vi "Gel Tugging Force Mode_Controller v15.20.vi"() -> ()   [LabVIEW 2015]
doc: "This example demonstrates how to continuously acquire voltage measurements from a DAQmx device using hardware timed, single point reads using a timed loop structure. The timed loop is controlled by the sample clock of the DAQ device. The device will read data on each tick of the sample clock. If an additional sample clock tick occurs before the current data point is read from the device or if the timed loop does not receive any sample clock ticks, a dialog will indicate that this has happened. \n\nHardware Timed Single Point acquisition works best when using a deterministic operating system (such as LabVIEW Real-Time). Because of the less deterministic nature of general purpose operating systems (such as Microsoft Windows), the software loop will not always take the exact same amount of time to execute, and this may lead to the occasional missed sample clock. \n\nFor instructions on how to connect your signals to the DAQ device, refer to your device documentation."
uses:
  <vilib>/Platform/TimedLoop/XDataNode/timing_clust.ctl
  <vilib>/Platform/TimedLoop/XDataNode/nitl_modes.ctl
  <vilib>/Platform/TimedLoop/XDataNode/wakeup.ctl
  <vilib>/dex/Flush And Wait Empty Condition.ctl
  <vilib>/DAQmx/read.llb/DAQmx Read (Analog 1D DBL NChan 1Samp).vi
  <vilib>/DAQmx/write.llb/DAQmx Write (Analog DBL 1Chan 1Samp).vi
  <vilib>/DAQmx/read.llb/DAQmx Read (Analog 2D DBL NChan NSamp).vi
  <vilib>/Analysis/baseanly.llb/Mean (DBL).vi
  <vilib>/DAQmx/create/channels.llb/DAQmx Create Channel (AI-Voltage-Basic).vi
  <vilib>/DAQmx/create/channels.llb/DAQmx Create Channel (AO-Voltage-Basic).vi
  <vilib>/DAQmx/configure/timing.llb/DAQmx Timing (Sample Clock).vi
  <vilib>/DAQmx/create/timing.llb/DAQmx Create Timing Source (Control Loop From Task).vi
  <vilib>/DAQmx/miscellaneous.llb/DAQmx Fill In Error Info.vi
  <vilib>/addons/control/pid/pid.llb/PID (DBL).vi
  <vilib>/addons/control/pid/pid.llb/PID Gain Schedule (DBL).vi
  <vilib>/platform/TimedLoop/XDataNode/XDataNode.xnode
  <vilib>/Analysis/NI_AALBase.lvlib
  <vilib>/addons/control/pid/NI_PID_pid.lvlib
  <vilib>/Platform/TimedLoop/XDataNode/XDNodeRunTimeDep.lvlib
  <vilib>/ptbypt/NI_PtbyPt.lvlib
panel:
  in  "1st OFF Length (s)":dbl=2.0
  out "Calibrating Sensor":bool
  out "Waveform Graph 2":dbl[](graph)
  in  "Ramp Total Interval (ms)":u32=490
  in  "# Ramp Steps":u32=7
  in  "9.            Step(s) Force Ramp in              (ms)?":bool=TRUE
  in  "ON":dbl=3.0
  out "DigitalTrigger":bool
  out "Corrective \nNull Flux (Gs)":dbl
  in  "7. Correct Null Flux after Cycle #1?":bool=TRUE
  out "# of Data Points":i64
  out "Loop Index":i32
  in  "6. Mini DeGauss cycles in OFF segments?":bool
  in  "Measure Flux Sensor Zero?":bool=TRUE
  out "PID gains ON Chosen":T1
  in  "Keep Null Flux Running \n       Until Next Step? 2":bool
  in  "Start Null Flux Adjustment 2":bool
  out "PID gains OFF Chosen":T1
  in  "Tweaked PID gains ON":T1={"proportional gain (Kc)"=0.7, "integral time (Ti, min)"=3.5e-06, "derivative time (Td, min)"=0.0}
  in  "Tweaked PID gains OFF":T1={"proportional gain (Kc)"=0.078, "integral time (Ti, min)"=3.5e-06, "derivative time (Td, min)"=0.0}
  out "Ready?":bool
  in  "4. Aggressiveness:":i32(listbox)
  out "of":i32
  in  "3. PID Parameters:":i32(listbox)
  out "ON Absolute\nFlux Setpoint (Gs)":dbl
  out "Suggested PID gains OFF":T1
  out "Suggested PID gains ON":T1
  out "Measured Magnetic Sensor 1 Zero, Mean (V)":dbl format="%_7g"
  in  "OFF (s)":dbl=4.0
  out "Round:":i32
  out "Ready?":bool
  out "Ready?":bool
  in  "Proceed with Parameters":bool
  out "Final Flux Running at End?":bool
  out "Sensor Sensitivity \n(V/Gs)":dbl
  in  "1. Sensor:":i32(listbox)
  out "Ready?":bool
  in  "2. Needle:":i32(listbox)
  in  "Proceed with Selection":bool
  in  "Ready?&\nData Logger Running":bool
  out "Null Flux \nCurrently\nRunning?":bool
  out "Real-Time Flux Control Currently Running?":bool
  out "Ready?":bool
  out "DeGaussing?":bool
  in  "Start DeGaussing":bool
  in  "Start Null Flux Adjustment":bool
  in  "1. Number of rounds":i32=3
  in  "Post-Wave Null Flux Interval (s)":dbl=4.0 format="%#_13g"
  in  "Pre-Wave Null Flux Interval (s)":dbl format="%#_13g"
  in  "8. Keep Final Flux Running at End?":bool=TRUE
  out "Flux Control Sequence Running & Uploading Data?":bool
  in  "3. Keep Null Flux Running \n       Until Next Step?":bool=TRUE
  in  "2. Adjust Magnetic Flux (GS):":dbl=3.5 min=-350.0 max=350.0 step=0.02 format="%#_13g"
  in  "4. Click Rocker to finish Null Flux Adjustment":bool
  in  "Number of Cycles":i32=3
  in  "Flux ON relative setpoint (Gs)":dbl=-175.0 format="%#_13g"
  # "For Gel Tugging Experiments v15.20 (Controlled-Flux or Force Mode)"
  # "WARNING: This program crashes the first 2 or 3 times it runs after the target has been shut down. \nWARNING: Do NOT run the power supply unattended with the needle attached. Always look at the amount of current periodically."
  # "Step 0-1: Place the needle at Z ~ 7000 micron in the field of view. Inclincation Angle= 25º for HyMu80#1 Needle"
  # "(Hit \"Enter\" \nor Toggle)"
  # "Step 0-2: DeGauss Needle:"
  # "Step 0-3: Measure the Value of Flux Sensor \"Zero\"?"
  # "Yes"
  # "No"
  # "(Note: Check if it is around 2.47±0.02 (V)):"
  # "Step 1: Choose Sensor & \nNeedle/PID Parameters\nfor This Experiment:"
  # "Step 2: Adjust Flux: \n(in Real-Time)"
  # "(Hit \"Enter\" \nor Toggle)"
  # "Yes"
  # "No"
  # "Make sure upper side of Rocker\n is pressed down before Program Starts"
  # "Step 3: Specify Control \n     Sequence Parameters:"
  # "1. Pre-Wave Null Flux Interval (s) (choose 0 if none desired):"
  # "2. Length of 2nd to end OFF"
  # "& ON"
  # "segments (s)."
  # "Length of 1st OFF"
  # "3. Number of OFF & ON Square-Wave Cycles:"
  # "Note 1: Use Negative Flux for waves in opposite direction\nNote 2: Linear Range is (±0-175 Gs) for Null Flux + Flux ON Setpoint\nNote 3: Check ON Absolute Flux Setpoint & PID Gains on first run.\nSometimes they can be glitchy. Abort & Re-run"
  # "4. Flux ON relative setpoint (Gs):"
  # "5. Post-Wave Null Flux Inteval (s) (choose 0 if none desired):"
  # "No"
  # "Yes"
  # "No"
  # "Yes"
  # "No"
  # "Yes"
  # "No"
  # "Yes"
  # "Step 4: Do you want to tweak these PID parameters?"
  # "Yes"
  # "No"
  # "vs."
  # "Step 5: Run Data Logger: Gel Tugging Force Mode_Data Logger_Auto-Manual Triggers v15.20.vi\n            Needs to be running to start the control sequence"
  # "Step 6-1: Lower the needle to the desired level for the experiment. Z ~ 3400 microns with TI-SH-U stage.\nStep 6-2: Click TRGR or Run Macro in Nikon Elements"
  # "datapoints uploaded"
  # "out of"
  # "Close the VI and start over. The VI sometimes freezes upon subsequent runs"
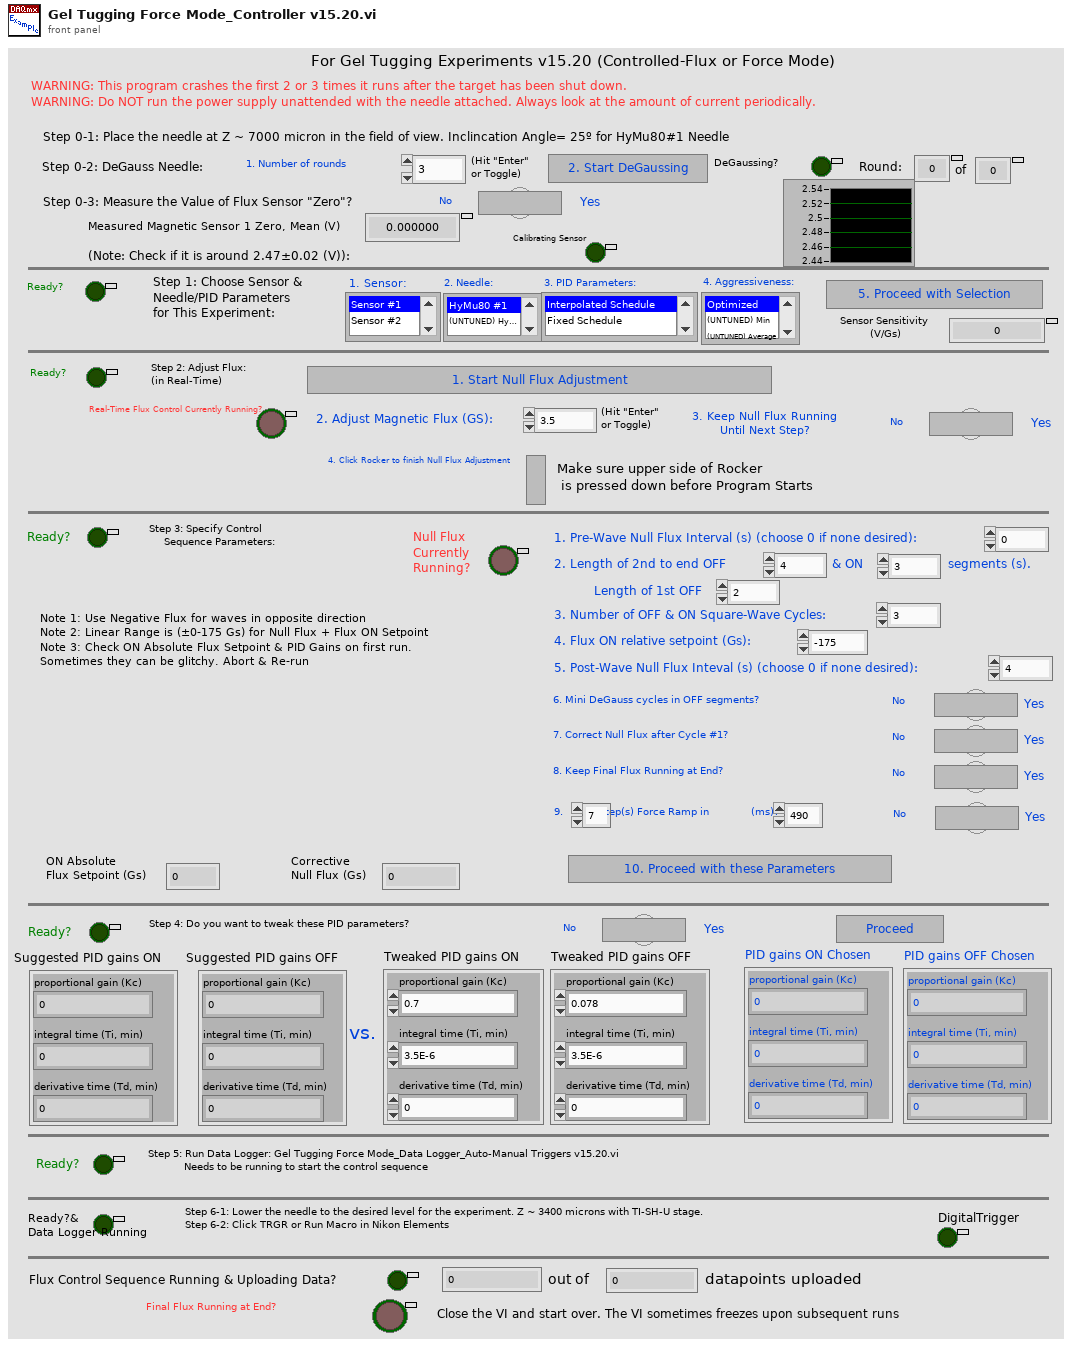
[diagram p1: front panel]
types:
  T1 = cluster{"proportional gain (Kc)":dbl, "integral time (Ti, min)":dbl, "derivative time (Td, min)":dbl}
  T2 = cluster{"PID gains":cluster{"proportional gain (Kc)":dbl, "integral time (Ti, min)":dbl, "derivative time (Td, min)":dbl}, "max value":dbl}[]
  T3 = typedef "XDNodeRunTimeDep.lvlib/timing_clust.ctl" = cluster{"Expected End [f-1]":u64, "Actual End [f-1]":u64, "Finished Late? [f-1]":bool, "Expected End [i-1]":u64, "Actual End [i-1]":u64, "Finished Late? [i-1]":bool, "Expected Start [i]":u64, "Actual Start [i]":u64, "Expected Start [f]":u64, "Actual Start [f]":u64, "Source Name":string, "Structure Name":string, "Period":i64, "Deadline":i64, "Offset":i64, "Start":i64, "Priority":i32, "Timeout":i32, "Mode":T4, "Wakeup Reason":T5, "Error":errorcluster, "Source Type":string, "Secondary Source Type":string, "Global End Time":u64, "Global Start Time":u64, "Frame Duration":u64, "Iteration Duration":u64, "Assigned CPU":i32, "I/O Scan Engine Mode":u32}
  T4 = typedef "XDNodeRunTimeDep.lvlib/nitl_modes.ctl" = enum32{"No Change", "Process missed periods, maintain original phase", "Discard missed periods, maintain original phase", "Process missed periods, ignore original phase", "Discard missed periods, ignore original phase"}
  T5 = typedef "XDNodeRunTimeDep.lvlib/wakeup.ctl" = enum32{"Normal", "Aborted", "Asynchronous wakeup", "Timing source error", "Timed loop error", "Timeout"}
  T6 = cluster{"Max/Min \ncontroller outputs":dbl, "output low":dbl}
  T7 = cluster{"PID gains":cluster{"proportional gain (Kc)":dbl, "integral time (Ti, min)":dbl, "derivative time (Td, min)":dbl}, "max value":dbl}
  T8 = typedef "Flush And Wait Empty Condition.ctl" = u8
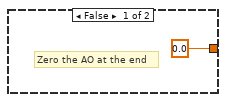
[diagram p2: hidden frame]
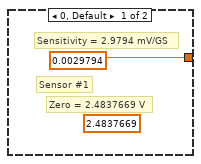
[diagram p4: hidden frame]
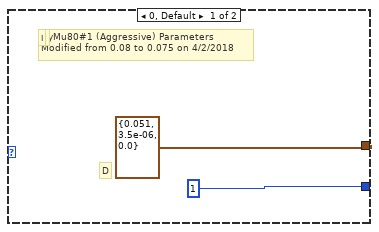
[diagram p5: hidden frame]
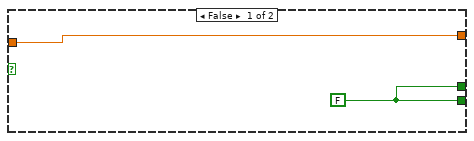
[diagram p6: hidden frame]
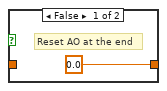
[diagram p7: hidden frame]
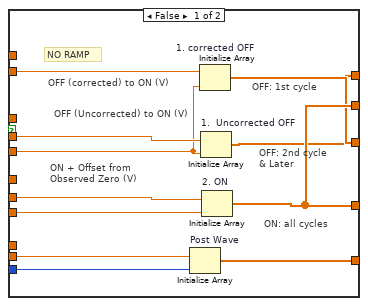
[diagram p9: hidden frame]
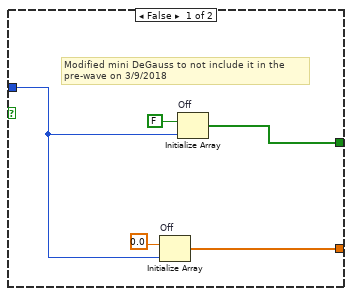
[diagram p11: hidden frame]
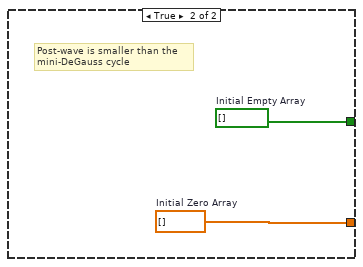
[diagram p12: hidden frame]
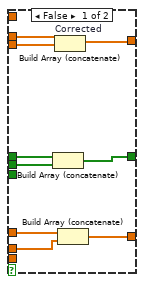
[diagram p14: hidden frame]
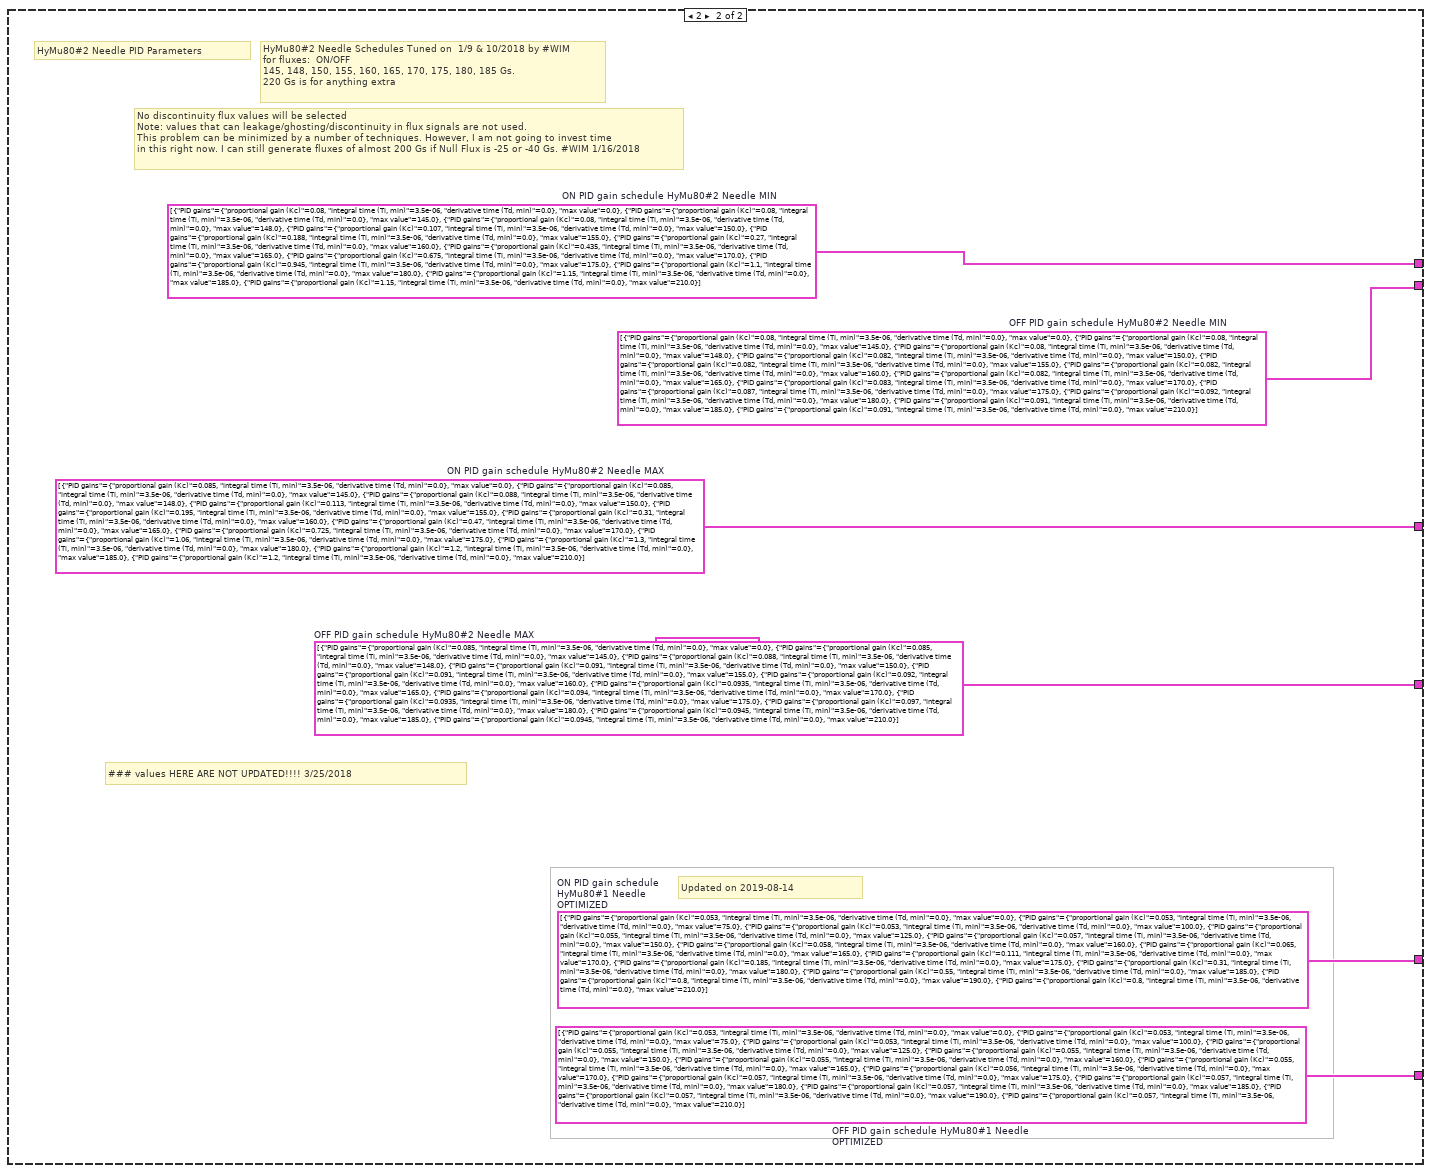
[diagram p18: hidden frame]
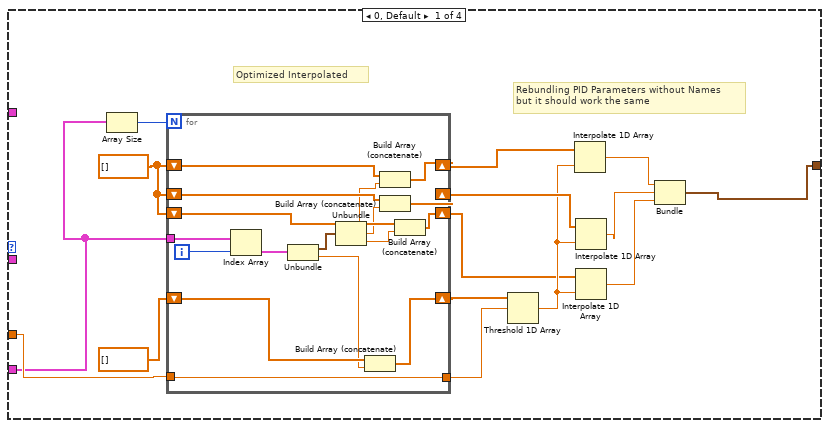
[diagram p19: hidden frame]
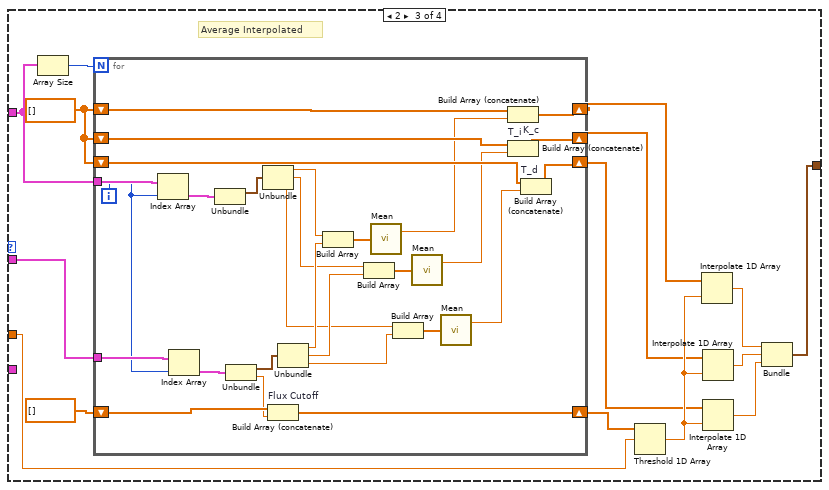
[diagram p20: hidden frame]
diagram:
  (unwired) T2 [{"PID gains"={"proportional gain (Kc)"=0.07, "integral time (Ti, min)"=3.5e-06, "derivative time (Td, min)"=0.0}, "max value"=0.0}, {"PID gains"={"proportional gain (Kc)"=0.07, "integral time (Ti, min)"=3.5e-06, "derivative time (Td, min)"=0.0}, "max value"=143.0}, {"PID gains"={"proportional gain (Kc)"=0.078, "integral time (Ti, min)"=3.5e-06, "derivative time (Td, min)"=0.0}, "max value"=148.0}, {"PID gains"={"proportional gain (Kc)"=0.078, "integral time (Ti, min)"=3.5e-06, "derivative time (Td, min)"=0.0}, "max value"=150.0}, {"PID gains"={"proportional gain (Kc)"=0.078, "integral time (Ti, min)"=3.5e-06, "derivative time (Td, min)"=0.0}, "max value"=155.0}, {"PID gains"={"proportional gain (Kc)"=0.078, "integral time (Ti, min)"=3.5e-06, "derivative time (Td, min)"=0.0}, "max value"=160.0}, {"PID gains"={"proportional gain (Kc)"=0.078, "integral time (Ti, min)"=3.5e-06, "derivative time (Td, min)"=0.0}, "max value"=165.0}, {"PID gains"={"proportional gain (Kc)"=0.078, "integral time (Ti, min)"=3.5e-06, "derivative time (Td, min)"=0.0}, "max value"=170.0}, {"PID gains"={"proportional gain (Kc)"=0.081, "integral time (Ti, min)"=3.5e-06, "derivative time (Td, min)"=0.0}, "max value"=175.0}, {"PID gains"={"proportional gain (Kc)"=0.081, "integral time (Ti, min)"=3.5e-06, "derivative time (Td, min)"=0.0}, "max value"=180.0}, {"PID gains"={"proportional gain (Kc)"=0.085, "integral time (Ti, min)"=3.5e-06, "derivative time (Td, min)"=0.0}, "max value"=185.0}, {"PID gains"={"proportional gain (Kc)"=0.086, "integral time (Ti, min)"=3.5e-06, "derivative time (Td, min)"=0.0}, "max value"=190.0}, {"PID gains"={"proportional gain (Kc)"=0.086, "integral time (Ti, min)"=0.01, "derivative time (Td, min)"=0.0}, "max value"=195.0}, {"PID gains"={"proportional gain (Kc)"=0.086, "integral time (Ti, min)"=0.01, "derivative time (Td, min)"=0.0}, "max value"=220.0}]  # OFF PID gain schedule HyMu80#1 Needle OPTIMIZED
  (unwired) T2 [{"PID gains"={"proportional gain (Kc)"=0.065, "integral time (Ti, min)"=3.5e-06, "derivative time (Td, min)"=0.0}, "max value"=0.0}, {"PID gains"={"proportional gain (Kc)"=0.065, "integral time (Ti, min)"=3.5e-06, "derivative time (Td, min)"=0.0}, "max value"=143.0}, {"PID gains"={"proportional gain (Kc)"=0.083, "integral time (Ti, min)"=3.5e-06, "derivative time (Td, min)"=0.0}, "max value"=148.0}, {"PID gains"={"proportional gain (Kc)"=0.084, "integral time (Ti, min)"=3.5e-06, "derivative time (Td, min)"=0.0}, "max value"=150.0}, {"PID gains"={"proportional gain (Kc)"=0.0875, "integral time (Ti, min)"=3.5e-06, "derivative time (Td, min)"=0.0}, "max value"=155.0}, {"PID gains"={"proportional gain (Kc)"=0.123, "integral time (Ti, min)"=3.5e-06, "derivative time (Td, min)"=0.0}, "max value"=160.0}, {"PID gains"={"proportional gain (Kc)"=0.187, "integral time (Ti, min)"=3.5e-06, "derivative time (Td, min)"=0.0}, "max value"=165.0}, {"PID gains"={"proportional gain (Kc)"=0.315, "integral time (Ti, min)"=3.5e-06, "derivative time (Td, min)"=0.0}, "max value"=170.0}, {"PID gains"={"proportional gain (Kc)"=0.46, "integral time (Ti, min)"=3.5e-06, "derivative time (Td, min)"=0.0}, "max value"=175.0}, {"PID gains"={"proportional gain (Kc)"=0.59, "integral time (Ti, min)"=3.5e-06, "derivative time (Td, min)"=0.0}, "max value"=180.0}, {"PID gains"={"proportional gain (Kc)"=0.8875, "integral time (Ti, min)"=3.5e-06, "derivative time (Td, min)"=0.0}, "max value"=185.0}, {"PID gains"={"proportional gain (Kc)"=1.04, "integral time (Ti, min)"=3.5e-06, "derivative time (Td, min)"=0.0}, "max value"=190.0}, {"PID gains"={"proportional gain (Kc)"=1.04, "integral time (Ti, min)"=0.01, "derivative time (Td, min)"=0.0}, "max value"=195.0}, {"PID gains"={"proportional gain (Kc)"=1.04, "integral time (Ti, min)"=0.01, "derivative time (Td, min)"=0.0}, "max value"=220.0}]  # ON PID gain schedule HyMu80#1 Needle OPTIMIZED
  (unwired) T2 [{"PID gains"={"proportional gain (Kc)"=0.07, "integral time (Ti, min)"=3.5e-06, "derivative time (Td, min)"=0.0}, "max value"=0.0}, {"PID gains"={"proportional gain (Kc)"=0.07, "integral time (Ti, min)"=3.5e-06, "derivative time (Td, min)"=0.0}, "max value"=116.0}, {"PID gains"={"proportional gain (Kc)"=0.078, "integral time (Ti, min)"=3.5e-06, "derivative time (Td, min)"=0.0}, "max value"=117.0}, {"PID gains"={"proportional gain (Kc)"=0.08, "integral time (Ti, min)"=3.5e-06, "derivative time (Td, min)"=0.0}, "max value"=120.0}, {"PID gains"={"proportional gain (Kc)"=0.08, "integral time (Ti, min)"=3.5e-06, "derivative time (Td, min)"=0.0}, "max value"=122.0}, {"PID gains"={"proportional gain (Kc)"=0.08, "integral time (Ti, min)"=3.5e-06, "derivative time (Td, min)"=0.0}, "max value"=125.0}, {"PID gains"={"proportional gain (Kc)"=0.08, "integral time (Ti, min)"=3.5e-06, "derivative time (Td, min)"=0.0}, "max value"=130.0}, {"PID gains"={"proportional gain (Kc)"=0.08, "integral time (Ti, min)"=3.5e-06, "derivative time (Td, min)"=0.0}, "max value"=135.0}, {"PID gains"={"proportional gain (Kc)"=0.08, "integral time (Ti, min)"=3.5e-06, "derivative time (Td, min)"=0.0}, "max value"=140.0}, {"PID gains"={"proportional gain (Kc)"=0.086, "integral time (Ti, min)"=3.5e-06, "derivative time (Td, min)"=0.0}, "max value"=145.0}, {"PID gains"={"proportional gain (Kc)"=0.096, "integral time (Ti, min)"=3.5e-06, "derivative time (Td, min)"=0.0}, "max value"=150.0}, {"PID gains"={"proportional gain (Kc)"=0.096, "integral time (Ti, min)"=3.5e-06, "derivative time (Td, min)"=0.0}, "max value"=200.0}]  # OFF PID gain schedule HyMu80#1 Needle OPTIMIZED
  (unwired) T2 [{"PID gains"={"proportional gain (Kc)"=0.07, "integral time (Ti, min)"=3.5e-06, "derivative time (Td, min)"=0.0}, "max value"=0.0}, {"PID gains"={"proportional gain (Kc)"=0.07, "integral time (Ti, min)"=3.5e-06, "derivative time (Td, min)"=0.0}, "max value"=116.0}, {"PID gains"={"proportional gain (Kc)"=0.08, "integral time (Ti, min)"=3.5e-06, "derivative time (Td, min)"=0.0}, "max value"=117.0}, {"PID gains"={"proportional gain (Kc)"=0.085, "integral time (Ti, min)"=3.5e-06, "derivative time (Td, min)"=0.0}, "max value"=120.0}, {"PID gains"={"proportional gain (Kc)"=0.115, "integral time (Ti, min)"=3.5e-06, "derivative time (Td, min)"=0.0}, "max value"=122.0}, {"PID gains"={"proportional gain (Kc)"=0.18, "integral time (Ti, min)"=3.5e-06, "derivative time (Td, min)"=0.0}, "max value"=125.0}, {"PID gains"={"proportional gain (Kc)"=0.31, "integral time (Ti, min)"=3.5e-06, "derivative time (Td, min)"=0.0}, "max value"=130.0}, {"PID gains"={"proportional gain (Kc)"=0.55, "integral time (Ti, min)"=3.5e-06, "derivative time (Td, min)"=0.0}, "max value"=135.0}, {"PID gains"={"proportional gain (Kc)"=0.95, "integral time (Ti, min)"=3.5e-06, "derivative time (Td, min)"=0.0}, "max value"=140.0}, {"PID gains"={"proportional gain (Kc)"=1.2, "integral time (Ti, min)"=3.5e-06, "derivative time (Td, min)"=0.0}, "max value"=145.0}, {"PID gains"={"proportional gain (Kc)"=1.3, "integral time (Ti, min)"=3.5e-06, "derivative time (Td, min)"=0.0}, "max value"=150.0}, {"PID gains"={"proportional gain (Kc)"=1.3, "integral time (Ti, min)"=3.5e-06, "derivative time (Td, min)"=0.0}, "max value"=200.0}]  # ON PID gain schedule HyMu80#1 Needle OPTIMIZED
  # "Note: Some quirks when running the program are: (as of 2/7/2018):\n1. First time you run it for the day, it will ask if you want to use the newer version instead of the old one already on the Remote Desktop computer\n2. Also, at the end of the first run, it will not stop. You will have to abort it. Some of the data points will be lost near the end. You might have to repeat that run.\n3. Do run the Data Reduction file or any other VIs in the DeGaussing stage. Otherwise, the program will crash."
  # "v15.20 Modified from v15.10 by Waddah Moghram on 2019-08-16 and thereafter:\n*Update based on Calibration_Core Flux Controller v11.00.vi\n\nv15.10 modified from v15.00 by  #Waddah #Moghram on 11/5/2018 and thereafter:\nTo be used with Data Logger v15.00 & Reduction v15.00: \n1. Modified it so that it can select PID gains from inside the loop\n2. Modified some PID gains at 170 Gs and higher.\n3.  Fixed the problem with the Post-wave zero Ramp 11/28/2019. WIM\n\nv 15.00 Modified from v12.00 by #Waddah #Moghram on 10/10/2018 and thereafter. To be used with Data Logger v1500 & Reduction v15.00: \n1. Replaced the Mini-DeGauss Routine with a Force Ramp (Linear vs. Steps?) since a step force function will be difficult to image-track. \n((Please refer to Linear and Step Ramps v1.00.vi for both linear and step ramps).\n*** Amount of step jump is assumed to be from ON-to-OFF and OFF-to-ON. That information is known\n2. Some of the parameters that will be used for the force ramp:\n*** Time interval: Assume that ON-to-OFF and OFF-to-ON ramps will have the same time frames.\n*** If discrete step are chosen. Choose the number of steps that it will take.\n\nv 11.00 Modified from v10.00 by #Waddah #Moghram on 4/26/2018 and thereafter. To be used with Data Logger v11.00 & Reduction v11.00: \n1. Resolve the issue of Digital Trigger automatically being released due to ground loop. Most likely due to construction that is happening around.\n* The Network digital trigger is released from the Master DAQ in the Data Logger, where it will be passed into here as a real-time global variable.\n2. For some reason, the first two runs usually crash, and the program still crashes a lot. I need to find a work around this one. \n\nv 10.00 Modified from v9.60 and v9.40 by #Waddah #Moghram on 4/4/2018 and thereafter: To be used with Data Logger v10.00 & Reduction v10.00\n1. Increased DeGauss Cycle to 2,000 milliseconds from 500 ms.\n2. Corrected the Dialog Boxes\n3. Added a switch for the Corrective Null Flux on the front panel, display it and send it to the Data Logger\n4. Corrected Mini-DeGauss Sampling Glitch where it was wired to the sampling rate directly instead of the one adjusted by the period 4/4/2018\n5. Based on a sigmoidal curve fit 4/18/2018.\nThe Equation is Y = Vmax * X^h /(K_prime + X^h), where Vmax = 10.7369, h = 1.91107, and Kprime = 3499.9. (and K_half = 71.5294))\n\n\nv 9.60 Modified from v9.50 by #Waddah #Moghram on 4/1/2018: \n1. It will correct for the Null Flux shift based on the Sigmoidal Fit that was collected from bead in front of the needle data,\nbased on a sigmoidal curve fit 4/2/2018. Experiments conducted 3/29/2018-4/2/2018. \nThe Equation is Y = Vmax * X^h /(K_prime + X^h), where Vmax = 11.4533, h = 1.69622, and Kprime = 1256.11)\n2. New Global Variable \"FluxObservedZeroGsCorrected\" to be inserted into the Data Logger v9.60\n\nv 9.50 Modified from v9.40 by #Waddah #Moghram on 3/29/2018:\n1. Used AI7 to hook up the 2nd Magnetic Sensor that will be placed in front of the sensor.\n2. Zero of 2nd Sensor is measured in the first step as well. The sensitivity is embedded in the data logger as well. \n3. Accompanies by v9.50 Data Logger.\n4. (GO BACK TO OLDER VERSION and add more details about modifications)\nFixed datapoints lost in the end due to the determinstic loop ending before the other loop. \n\nv 9.40 Modified from v9.20 by #Waddah #Moghram on 3/19/2018\n1. Removed Offset and kept amplitude +/- 10V for MiniDeGauss waveforms from inside the deterrministic loop.\n2. Shuffled the Suggested PID Loop parameters until before the \"Proceed button to allow the user to take a look at them. \n3. 3/22/2018. Reverted back to unshielded magnetic sensor, but with wire propped away from sensor.\nAlso, TI-SH-U is used and the needle is placed at Z~4600 microns for PID tuning with an inclination angle of 20 degrees\n(#OLD: 3. Re-optimized on 3/20/2018 for HyMu80#1 after shielding the sensor. The values were shifted down by 23 Gs   3/20/2018 )\n(#OLD: 4. Relocated PID Gains Selected on the front panel for more clarity 3/21/2018.)\n\nv 9.20 Modified from v9.05 and v9.10 by #Waddah #Moghram on 3/12/2018 and thereafter:\n1. It is back to OFF/ON Sequences, except first OFF segment and pre-waves have no DeGauss. It turns out to be an easy fix. \n2. Modified mini-DeGauss time \n3. Tied variables to make the wave sample properly. See notes for calculations.\n4. Turn OFF \"Null Flux Running Middle\" when control sequence starts. 3/17/2018 WIM \n5. Modified PID Parameters for #Interpolated #Optimized #HyMu80#1. Other parameters will need to be modified later on. \n6. Updated front panel to indicate inclination Angle, and Z-level for both Sensor Zero Measurement and Control Sequence.   3/18/2018\n****It turns out the PID parameters are sensitive to both z-level and inclination angle (which affect the Sensor Zero Measurement).*****\n***NOTE: First run usually does not end by itself. You will have to abort it. It will result in the loss of the last few hundred data points, but that is not too critical. Otherwise, run once, then run again. It should run smoothly every time afterwards. This is one of the quirks of working with LabVIEW. 3/18/2018\n\nv 9.05 Modified from v9.00 by #Waddah #Moghram on 3/12/2018:\n1. Modified Magnitude of Mini-DeGauss cycle from ** Maximum of (AO of Null Flux (AO_nf) or AO of ON (AO_on)) ** to **AO_nf + AO_on**\n2. The mini DeGauss oscillates about AO_nf instead of 0\n\nv 9.00 Modified from v8.40 by #Waddah #Moghram on 3/7/2018 and thereafter:\n1. It will include mini-DeGauss Cycles in the beginning of the OFF segments before PID control kicks back in. This is in an effort to minimize Magnetic Sensor hysteresis at Null Flux Observed\n(Sinusoidally Decaying Waveform Embedded in Control Sequence v1.0.vi is used for initially testing of mini-DeGauss waveforms).\n** So far, the selected waveform is about ~ 15 cycles that exponentially decay under 30 milliseconds. Used a Cosine waveform instead of sine (Sin with 90 degree phase shift).\n** Middle point is AO = 0, Magnitude between max and middle point is AO_last**    (3/12/2018)\n2. Sequence is created externally to minimize Loop calculation time. The AO Mini-DeGauss will only to be multiplied by the amplitude of the last AO out. \n3. Switched #AI6 to #AI3. Some errors with AI6 signal on the DAQ on 3/8/2018\n4. Fixed the glitch where the PID loop overreacted when the PID starts again and the Setpoint point is close to the Process variable. (Kudos to #Dr. #Selby for catching it!). on 3/8/2018\n5. Replaced \"Zero Flux\" with \"Null Flux\" for labels to avoid confusion since it is not really zero\n\nv 8.40 Modified from v8.30 by #Waddah #Moghram on 3/1/2018, and thereafter: \n1. Added a toggle to allow the re-calibration of magnetic sensor Zero or not\n2. Global Variables for DeGauss Cycles Total & Round\n3. Modified Tabbing order on 3/4/2018\n4. Fixed AO 0 initialized before PID loop to keep the value saved from \"keep Null Flux Running\" step on 3/5/2018. It was creating a blip in PID response. However, that does not seem to resolve the problem.\n\nv 8.30 Modified from v8.20 by #Waddah #Moghram on 2/22/2018:\n1. Using the measured magnetic sensor zero to create the control sequence after DeGaussing instead of the one recorded a while back inside a shielded data.\nThis is because it will change a lot over time with thermal drift and so forth. \n2. Reset the value of the sensor zero every time even no deGaussing was done.\n\nv 8.20 Modified from v8.10 by #Waddah #Moghram on 2/2/2018: \n1. This will allow the user to tweak the PID Parameters one more time before the actual experiment. This was found because it turns out that PID parameters can shift with time especially for values in the non-linear range.\n\nv. 8.10 Modified from v8.00 by #Waddah #Moghram on 1/10/2018 and thereafter:\n1. Scrapped fitted PID gains and used interpolated schedules in addition to schedules\n2. Updated PID Values for Gains and so forth.\n\nv 8.00 Modified from v7.40 by #Waddah #Moghram on 1/1/2018 and thereafter:\n1. Used the PID Gains from PID Tuning experiments \n2. Removed Normal vs. Aggressive and now will only use one set of parameters such that only one set of parameters are used\n3. Created a choice of Scheduled vs. Fitted Parameters. 1/8/2018.\n4. Fixed glitch that passed old values of waveform parameters to the global variable 1/8/2018. \n\nv 7.40 Modified from v 7.30 by #Waddah #Moghram on 12/22/2017 to including the following:\n1. Shifting the flux check and current reset only if DeGuassing Cycle required is not equal to zero. Otherwise, skip it, and keep the current running. I did this in case I need more than one run without removing the needle from the sample\n2. corrected total number of data points to allow for more than 2 seconds 1/4/2018 by #WIM\n\nv 7.30 Modified from v 7.20 by #Waddah #Moghram on 12/21/2017 to including the following:\n1. Removed Magnetic Flux Sensor Zero Calibration step, and embedded that value in the sensor section. The idea for doing that is that I want the flux values stated to be absolute. Thermal drift of sensor should not matter since PID should still work regardless of where the zero lies. Moreover, if I am accounting for the Null Flux observed, it should not matter what the absolute flux zero is.\n2. However, I kept the AO reset and used the AI2 to keep it running and also measured sensor values for 2 seconds to make sure that my values are controlled properly.\n3. Steps were re-numbered\n\nv 7.20 Modified from v7.10 by #Waddah #Moghram on 12/18/2017 to include the following:\n1. Custom-Length Waveforms. Data Reduction & Logger will be changed accordingly.\n2. Added Normal (~40 ms response time) vs. Aggressive (~22 ms response time) PID Parameters on 12/20/2017\n\nV 7.10 Modified from v7.00 by #Waddah #Moghram on 12/18/2017 to include the following:\n1. Switch order of DeGaussing & Calibrating Zero of Sensor. First Ensure that there is no residual magnetic. And secondly, reset AO just in case!\n\nv 7.00 Modified from v6.00 by #Waddah #Moghram on 12/18/2017 to include the following:\n1. Calibrated Null Flux at the beginning of the experiment without shielding to account for thermal drifts:\n*** Imported from \"01 Magnetic Sensor Zero Calibration v2.0 - Target.vi\"\n2. Included Second per Cycle\n3. Cleanup interface & Changed Step Numbers.\n\nv 6.00 Modified from v5.22 by #Waddah #Moghram on 12/5/2017 to include the following: \n1. Newer Magnetic Sensor Sensitivities: Sensor 1 is 2.9794 mV/GS and Sensor 2 is 3.0418 mV/GS\n2. Newer Magnetic Sensor Zeroes when unshielded: Sensor 1 is 2.4837669 V and Sensor 2 is 2.4928421 V\nThis program will also be used also to tune the PID in addition Magnetic Needle Choices\nOn 12/13/2017, I overhauled the interface to streamline the proceess and fixed a few glitches that allowed the program to \nchose parameters before clicking on the digital trigger\n\nv 5.22 Modified from v.5.20 by #Waddah #Moghram on 9/25/2017 to include the following:\n1. Remove prompt to calibrate the magnetic sensor and run Null Flux program\n2. Embedded the calibrated Null Flux value into the program, now that the sensor is fixed to the HyMu80 needle #1\n\n\nv5.00 modified from v.3.70 and v.4.10 by #Waddah #Moghram. It should integrate variables from both VIs.\nOther modification include:\n1. User-Defined Pre-experiment Null Flux Period\n2. User-Defined Post-experiment Null Flux Period\nModified on 8/14&15/2017 to streamline the VI even more. Ran into some Ground Loop Issues in the meantime. See Lab Notes for details.\n\nv4.10 Modified on 8/8/2017 to:\n* account for AI5 only for flux sensor values being fed to PID control.\nNotice the PID control scheme process variable is different in that it is not subtracted from the setpoint as in v.3.70 in the first PID Loop\n*modified PID parameters to the optimized ones found (subject to verification)."
  # "Re-optimized on 3/21/2018 for HyMu80#1 after shielding the sensor. The cutoff values were shifted down by ~23-27 Gs\nPreviously Optimized on 3/17/2018 for HyMu80#1 Optimized. The rest will need to be updated later\nAdded 139 Gs to keep fixed values in between 0 and 140 Gs.   Flux at 150 Gs has a response time of ~80 ms. \nAny higher PID gains will result in spike"
  # "Unshielded Previously"
  # "TOTALLY SHIELDED PARAMETERS"
  # "AI"
  # "AO"
  n1 = flat-sequence {
    tunnel: [w332] -> w96
    tunnel: [w331] -> w95
    tunnel: [w330] -> w88
    tunnel: [w329] -> w76
    tunnel: [w344] -> w104
    tunnel: w96 -> [w342]
    tunnel: w95 -> [w341]
    tunnel: w88 -> [w340]
    tunnel: [w340] -> w87
    tunnel: [w339] -> w77
    tunnel: w76 -> [w339]
    tunnel: [w354] -> w105
    tunnel: w104 -> [w354]
    tunnel: w87 -> [w353]
    tunnel: [w353] -> w86
    tunnel: [w352] -> w78
    tunnel: w77 -> [w352]
    tunnel: w105 -> [w360]
    tunnel: [w359] -> w102
    tunnel: [w358] -> w90
    tunnel: w86 -> [w358]
    tunnel: [w357] -> w79
    tunnel: w78 -> [w357]
    tunnel: [w371] -> w114
    tunnel: [w370] -> w113
    tunnel: [w369] -> w112
    tunnel: [w368] -> w103
    tunnel: w102 -> [w368]
    tunnel: w90 -> [w367]
    tunnel: [w367] -> w89
    tunnel: [w365] -> w85
    tunnel: w79 -> [w366]
    tunnel: [w366] -> w75
    tunnel: w114 -> [w413]
    tunnel: w113 -> [w412]
    tunnel: w112 -> [w411]
    tunnel: [w410] -> w108
    tunnel: [w409] -> w107
    tunnel: [w408] -> w106
    tunnel: w103 -> [w399]
    tunnel: [w397] -> w92
    tunnel: w89 -> [w397]
    tunnel: w85 -> [w396]
    tunnel: w75 -> [w395]
    tunnel: [w395] -> w73
    tunnel: [w394] -> w58
    tunnel: w108 -> [w488]
    tunnel: w107 -> [w487]
    tunnel: w106 -> [w486]
    tunnel: w92 -> [w485]
    tunnel: [w485] -> w91
    tunnel: [w484] -> w74
    tunnel: w73 -> [w484]
    tunnel: [w483] -> w59
    tunnel: w58 -> [w483]
    tunnel: [w496] -> w94
    tunnel: w91 -> [w496]
    tunnel: w74 -> [w495]
    tunnel: [w495] -> w71
    tunnel: w59 -> [w494]
    tunnel: [w494] -> w56
    tunnel: [w508] -> w101
    tunnel: [w507] -> w100
    tunnel: [w506] -> w99
    tunnel: [w505] -> w98
    tunnel: [w504] -> w97
    tunnel: w94 -> [w503]
    tunnel: [w503] -> w93
    tunnel: [w502] -> w72
    tunnel: w71 -> [w502]
    tunnel: [w501] -> w57
    tunnel: w56 -> [w501]
    tunnel: [w500] -> w11
    tunnel: [w499] -> w10
    tunnel: [w518] -> w83
    tunnel: [w535] -> w84
    tunnel: [w680] -> w82
    tunnel: [w672] -> w81
    tunnel: w101 -> [w601]
    tunnel: w100 -> [w671]
    tunnel: w99 -> [w670]
    tunnel: w98 -> [w669]
    tunnel: w97 -> [w668]
    tunnel: [w667] -> w80
    tunnel: w93 -> [w667]
    tunnel: w72 -> [w666]
    tunnel: [w666] -> w70
    tunnel: w57 -> [w665]
    tunnel: [w665] -> w55
    tunnel: [w651] -> w50
    tunnel: [w637] -> w49
    tunnel: [w616] -> w46
    tunnel: [w610] -> w43
    tunnel: w11 -> [w520]
    tunnel: w10 -> [w595]
    tunnel: [w520] -> w1
    tunnel: w84 -> [w814]
    tunnel: [w813] -> w69
    tunnel: w83 -> [_]
    tunnel: w82 -> [w810]
    tunnel: [w809] -> w67
    tunnel: [w827] -> w65
    tunnel: w81 -> [w818]
    tunnel: [w817] -> w63
    tunnel: [w826] -> w61
    tunnel: w80 -> [w832]
    tunnel: w70 -> [w831]
    tunnel: w55 -> [w811]
    tunnel: [w811] -> w53
    tunnel: [w819] -> w52
    tunnel: w50 -> [w820]
    tunnel: w49 -> [w816]
    tunnel: [w815] -> w48
    tunnel: w46 -> [w829]
    tunnel: [w829] -> w45
    tunnel: w43 -> [w828]
    tunnel: [w828] -> w42
    tunnel: [w825] -> w9
    tunnel: [w824] -> w8
    tunnel: w1 -> [w822]
    tunnel: w69 -> [w1250]
    tunnel: [w1250] -> w68
    tunnel: w67 -> [w1249]
    tunnel: [w1249] -> w66
    tunnel: w65 -> [w1247]
    tunnel: [w1243] -> w64
    tunnel: w63 -> [w1248]
    tunnel: [w1248] -> w62
    tunnel: w61 -> [w1246]
    tunnel: [w1242] -> w60
    tunnel: [w1241] -> w54
    tunnel: w53 -> [w1241]
    tunnel: w52 -> [w1240]
    tunnel: [w1240] -> w51
    tunnel: w48 -> [w1239]
    tunnel: [w1239] -> w47
    tunnel: w45 -> [w1238]
    tunnel: [w1238] -> w44
    tunnel: w42 -> [w1237]
    tunnel: [w1237] -> w41
    tunnel: w9 -> [w1234]
    tunnel: w8 -> [w1233]
    tunnel: [w1234] -> w7
    tunnel: [w1233] -> w6
    tunnel: w68 -> [w1288]
    tunnel: [w1290] -> w40
    tunnel: [w1291] -> w38
    tunnel: [w1283] -> w36
    tunnel: [w1288] -> w34
    tunnel: [w1272] -> w33
    tunnel: [w1287] -> w32
    tunnel: w66 -> [w1280]
    tunnel: [w1280] -> w30
    tunnel: [w1284] -> w28
    tunnel: w64 -> [w1284]
    tunnel: w62 -> [w1286]
    tunnel: [w1286] -> w26
    tunnel: w60 -> [w1285]
    tunnel: [w1285] -> w25
    tunnel: w54 -> [w1281]
    tunnel: [w1281] -> w24
    tunnel: w51 -> [w1279]
    tunnel: [w1279] -> w22
    tunnel: w47 -> [w1278]
    tunnel: [w1278] -> w20
    tunnel: [w1277] -> w18
    tunnel: w44 -> [w1277]
    tunnel: w41 -> [w1276]
    tunnel: [w1276] -> w17
    tunnel: w7 -> [w1274]
    tunnel: w6 -> [w1275]
    tunnel: [w1275] -> w5
    tunnel: [w1274] -> w4
    tunnel: w40 -> [w1316]
    tunnel: [w1315] -> w39
    tunnel: w38 -> [w1318]
    tunnel: [w1317] -> w37
    tunnel: w36 -> [w1320]
    tunnel: [w1319] -> w35
    tunnel: w34 -> [w1322]
    tunnel: w33 -> [w1324]
    tunnel: w32 -> [w1342]
    tunnel: [w1341] -> w31
    tunnel: w30 -> [w1328]
    tunnel: [w1327] -> w29
    tunnel: w28 -> [w1335]
    tunnel: [w1336] -> w27
    tunnel: w26 -> [w1334]
    tunnel: w25 -> [w1338]
    tunnel: w24 -> [w1340]
    tunnel: [w1339] -> w23
    tunnel: w22 -> [w1332]
    tunnel: [w1331] -> w21
    tunnel: w20 -> [w1330]
    tunnel: [w1329] -> w19
    tunnel: w18 -> [_]
    tunnel: w17 -> [w1326]
    tunnel: [w1325] -> w16
    tunnel: [w1337] -> w15
    tunnel: [w1333] -> w14
    tunnel: [w1323] -> w13
    tunnel: [w1321] -> w12
    tunnel: w5 -> [w1314]
    tunnel: w4 -> [w1313]
    tunnel: [w1312] -> w3
    tunnel: [w1311] -> w2
    tunnel: w39 -> [w1428]
    tunnel: w37 -> [w1429]
    tunnel: w35 -> [w1425]
    tunnel: w31 -> [w1391]
    tunnel: [w1411] -> w111
    tunnel: [w1394] -> w110
    tunnel: w29 -> [w1393]
    tunnel: [w1383] -> w109
    tunnel: w27 -> [w1382]
    tunnel: w23 -> [w1374]
    tunnel: w21 -> [w1381]
    tunnel: w19 -> [w1379]
    tunnel: w16 -> [w1371]
    tunnel: w15 -> [w1387]
    tunnel: w14 -> [w1389]
    tunnel: w13 -> [w1380]
    tunnel: w12 -> [w1421]
    tunnel: w3 -> [w1364]
    tunnel: w2 -> [w1362]
    tunnel: w111 -> [w1648]
    tunnel: w110 -> [w1647]
    tunnel: w109 -> [w1649]
    frame #0 {
      # "Removed the thermocouple  * AI2 is connected to Thermocouple cable."
      # "Switched Ai6 to AI3 on 3/8/2018 \nSome issues with AI6 on DEV2"
      # "1. SPECIFY the number of DeGaussing Cycle. CLICK \"Start DeGaussing.\"\n2. SPECIFY the Sensor & Needle in use for this experiment."
      n2 = One Button Dialog(message="BEFORE YOU START: \n* VERIFY these DAQ-2/Slave cables are connected as the following:\n   * AI5 is connected to Magnetic Flux \"Sensor Output - RAW\" on the Magnetic sensor box.   \n   * AI3 is connected to \"Current Sensor (1A/V)\" on the Load Box.\n   * AI7 is connected to Camera \"Exposure Sensor.\"\n   * Digital Trigger from DAQ-3/Master Output \"PF0.0\" is connected to Digital Trigger Input \"PFI0.\"\n* VERIFY these DAQ-3/Master Cables are connected as the following:\n   * Digital Trigger is connected to \"PF0.0\" BOTH \"PFI0\" on the same board and to \"PFI0\" on DAQ2/Slave.\n  \n* TURN ON power supply for half an hour. TURN ON fan control for load box (if needed).\n           WARNING: Check load is connected at the back of the load box to the back of the  power supply.\n           WARNING: Check if magnetic coil is connected to the load box if the toggle is switched to \"COIL+1OHM RESISTOR\" on the Load Box.\n           WARNING: Do NOT Position Needle in solution/cells just yet.\n           WARNING: Do NOT Position Needle in solution/cells just yet.\nIf you have not done these steps. Stop the program, then run it when ready.\n===============================\nClick OK then follow the steps", button name ("OK")="OK!") -> ()  [unwired: 1 out]
    }
    frame #1 {
      w117 = 0.0 ("DataRT Index")
      w126 = tag "Dev2/ai4, Dev2/ai5, Dev2/ai7, Dev2/ai2, Dev2/ai3"  # AI2:Dummy,AI3: Current, AI4: Dummy,AI5:Flux, AI7: Camera  Changed Ai5 to Ai1 on 2021-04-13
      w130 = FALSE ("DeGuassing Needle")
      # "Added on 4/24/2018"
      # "RESET VARIABLES"
      n3 = shared-variable ".\\Kopco PS Project Target Variables Library.lvlib\\Data Logger Running RT"(w130) -> ()  [unwired: 1 in, 1 out]
      n4 = shared-variable "NI-GenericDesktopPC-3A84958E\\Kopco PS Project Target Variables Library.lvlib\\Needle Selection Finished"(w130) -> ()  [unwired: 1 in, 1 out]
      n5 = shared-variable "NI-GenericDesktopPC-3A84958E\\Kopco PS Project Target Variables Library.lvlib\\Control Parameters Selected"(w130) -> ()  [unwired: 1 in, 1 out]
      n6 = shared-variable "NI-GenericDesktopPC-3A84958E\\Kopco PS Project Target Variables Library.lvlib\\DeGuassing Finished"(w130) -> ()  [unwired: 1 in, 1 out]
      n7 = shared-variable "NI-GenericDesktopPC-3A84958E\\Kopco PS Project Target Variables Library.lvlib\\DeGuassing Needle"(w130) -> ()  [unwired: 1 in, 1 out]
      n8 = shared-variable "NI-GenericDesktopPC-3A84958E\\Kopco PS Project Target Variables Library.lvlib\\Null Flux Selected"(w130) -> ()  [unwired: 1 in, 1 out]
      n9 = shared-variable ".\\Kopco PS Project Target Variables Library.lvlib\\Data Upload"(w130) -> ()  [unwired: 1 in, 1 out]
      n10 = shared-variable "NI-GenericDesktopPC-3A84958E\\Kopco PS Project Target Variables Library.lvlib\\Flux RT Control"(w130) -> ()  [unwired: 1 in, 1 out]
      n11 = shared-variable "NI-GenericDesktopPC-3A84958E\\Kopco PS Project Target Variables Library.lvlib\\Flux Control Sequence Running"(w130) -> ()  [unwired: 1 in, 1 out]
      n12 = shared-variable "NI-GenericDesktopPC-3A84958E\\Kopco PS Project Target Variables Library.lvlib\\Null Flux Running Middle"(w130) -> ()  [unwired: 1 in, 1 out]
      n13 = shared-variable "NI-GenericDesktopPC-3A84958E\\Kopco PS Project Target Variables Library.lvlib\\Null Flux Running End"(w130) -> ()  [unwired: 1 in, 1 out]
      n14 = shared-variable "NI-GenericDesktopPC-3A84958E\\Kopco PS Project Target Variables Library.lvlib\\Zero Flux Calibrated Found"(w130) -> ()  [unwired: 1 in, 1 out]
      n15 = shared-variable "NI-GenericDesktopPC-3A84958E\\Kopco PS Project Target Variables Library.lvlib\\PID Parameters Selected"(w130) -> ()  [unwired: 1 in, 1 out]
      n16 = shared-variable "NI-GenericDesktopPC-3A84958E\\Kopco PS Project Target Variables Library.lvlib\\Digital Trigger"(w130) -> ()  [unwired: 1 in, 1 out]
      n17 = shared-variable ".\\Kopco PS Project Target Variables Library.lvlib\\Data Logger Running"(w130) -> ()  [unwired: 1 in, 1 out]
      n18 = shared-variable ".\\Kopco PS Project Target Variables Library.lvlib\\Data RT Flux"(w117) -> ()  [unwired: 1 in, 1 out]
      n19 = shared-variable ".\\Kopco PS Project Target Variables Library.lvlib\\Data RT Exposure"(w117) -> ()  [unwired: 1 in, 1 out]
      n20 = shared-variable ".\\Kopco PS Project Target Variables Library.lvlib\\Data RT Current"(w117) -> ()  [unwired: 1 in, 1 out]
      n21 = shared-variable ".\\Kopco PS Project Target Variables Library.lvlib\\Data RT Index"(i64 0 ("DataRT Index")) -> ()  [unwired: 1 in, 1 out]
      n22 = shared-variable ".\\Kopco PS Project Target Variables Library.lvlib\\Last Current AO"(0.0 ("Last Current AO")) -> ()  [unwired: 1 in, 1 out]
      n23 = shared-variable "NI-GenericDesktopPC-3A84958E\\Kopco PS Project Target Variables Library.lvlib\\Experiment Settings Entered"(w130) -> ()  [unwired: 1 in, 1 out]
      n24 = shared-variable "NI-GenericDesktopPC-3A84958E\\Kopco PS Project Target Variables Library.lvlib\\Sensor Zero Calibrating"(w130) -> ()  [unwired: 1 in, 1 out]
      n25 = shared-variable "NI-GenericDesktopPC-3A84958E\\Kopco PS Project Target Variables Library.lvlib\\Ramp Total Interval (ms)"(i16 0 ("Ramp Total Interval (ms)")) -> ()  [unwired: 1 in, 1 out]
      n26 = shared-variable "NI-GenericDesktopPC-3A84958E\\Kopco PS Project Target Variables Library.lvlib\\Ramp Steps"(i16 0 ("Ramp Steps")) -> ()  [unwired: 1 in, 1 out]
      n27 = shared-variable "NI-GenericDesktopPC-3A84958E\\Kopco PS Project Target Variables Library.lvlib\\DeGauss Round Num"(i16 0 ("DeGauss Round Num")) -> ()  [unwired: 1 in, 1 out]
      n28 = shared-variable "NI-GenericDesktopPC-3A84958E\\Kopco PS Project Target Variables Library.lvlib\\DeGauss Total"(i16 0 ("DeGauss Total")) -> ()  [unwired: 1 in, 1 out]
      n29 = shared-variable "NI-GenericDesktopPC-3A84958E\\Kopco PS Project Target Variables Library.lvlib\\Cycles"(i16 0 ("Cycles")) -> ()  [unwired: 1 in, 1 out]
      n30 = shared-variable "NI-GenericDesktopPC-3A84958E\\Kopco PS Project Target Variables Library.lvlib\\Channels AI List"(w126) -> ()  [unwired: 1 in, 1 out]
      n31 = shared-variable "NI-GenericDesktopPC-3A84958E\\Kopco PS Project Target Variables Library.lvlib\\Sampling Rate"(30000.0 ("Sampling Rate")) -> ()  [unwired: 1 in, 1 out]
      n32 = shared-variable "NI-GenericDesktopPC-3A84958E\\Kopco PS Project Target Variables Library.lvlib\\Sensor Index Flux Core"(i8 1 ("Sensor Index Flux Core")) -> ()  [unwired: 1 in, 1 out]
      n33 = shared-variable "NI-GenericDesktopPC-3A84958E\\Kopco PS Project Target Variables Library.lvlib\\Sensor Index Camera"(i8 2 ("Sensor Index Flux Core")) -> ()  [unwired: 1 in, 1 out]
      n34 = shared-variable "NI-GenericDesktopPC-3A84958E\\Kopco PS Project Target Variables Library.lvlib\\Sensor Index Current"(i8 4 ("Sensor Index Flux Core")) -> ()  [unwired: 1 in, 1 out]
    }
    frame #2 {
      # "#STEP #0"
      n35 = while {
        tunnel: ["Start DeGaussing"] -> w131
        stop <- "Start DeGaussing" stop-if-true
      }
      n36 = shared-variable "NI-GenericDesktopPC-3A84958E\\Kopco PS Project Target Variables Library.lvlib\\DeGuassing Needle"(w131) -> ()  [unwired: 1 in, 1 out]
    }
    frame #3 {
      # "bound to \n\"DeGaussing Needle\"\nshared global variable"
      # "Bound to \n\"DeGauss Round Num\""
      # "Bound to \"DeGauss Total\""
      n37 = shared-variable "NI-GenericDesktopPC-3A84958E\\Kopco PS Project Target Variables Library.lvlib\\DeGauss Total"("1. Number of rounds") -> ()  [unwired: 1 in, 1 out]
      n38 = for {
        N: "1. Number of rounds" -> [_]
        i -> [w140]
        # "Wait half a second\nbetween repititions \nto allow the system \nto stabilize\n\nAdded by WIM on \n12/18/2017\n\nUpdated to 2 Seconds\nfrom 500 ms"
        # "First Index is 0"
        n39 = Add(x=1, y=w140) -> (x+y=w134:i32)
        n40 = shared-variable "NI-GenericDesktopPC-3A84958E\\Kopco PS Project Target Variables Library.lvlib\\DeGauss Round Num"(w134) -> ()  [unwired: 1 in, 1 out]
        n41 = Wait (ms)(milliseconds to wait=u32 2000) -> ()  [unwired: 1 out]
        n42 = flat-sequence {
          tunnel: [w152] -> w149
          tunnel: [w150] -> w148
          tunnel: w134 -> [w151]
          tunnel: [w151] -> w137
          tunnel: w149 -> [w174]
          tunnel: [w181] -> w147
          tunnel: [w173] -> w146
          tunnel: [w187] -> w145
          tunnel: w148 -> [w172]
          tunnel: [w172] -> w144
          tunnel: w137 -> [w171]
          tunnel: [w171] -> w136
          tunnel: w147 -> [w204]
          tunnel: w146 -> [w205]
          tunnel: w145 -> [w212]
          tunnel: [w211] -> w143
          tunnel: [w210] -> w142
          tunnel: [w209] -> w141
          tunnel: w144 -> [w202]
          tunnel: w136 -> [w200]
          tunnel: [w200] -> w135
          tunnel: w143 -> [w247]
          tunnel: w142 -> [w246]
          tunnel: w141 -> [w242]
          tunnel: w135 -> [_]
          frame #0 {
            w153 = 5  # Time in Seconds
            w152 = 6000  # Sampling Rate (Samples/Seconds)
            # "Step 0 DeGaussing"
            # "Hardware-Time control loop cannot keep up\nwith 50,000 Hz frequence."
            n43 = Multiply(x=w153, y=w152) -> (x*y=w154:i32)
            n44 = for "A Single DeGuassing Waveform" {
              N: w154 -> [_]
              tunnel: w152 -> [w158]
              tunnel: [w155] -> w150 mode=indexing
              i -> [w157]
              (unwired) 0.3 ("y")
              w161 = 1.0  # A_0
              w164 = 1.0  # Lambda
              w168 = 0.0  # No phase
              w169 = 60.0  # Frequency, 60 Hz
              w170 = 10.0  # 4 amps = 10V
              # "Minimized 10 V to 5 V on 3/19/2018\nadd an offset of 0.3V for now"
              # "Lambda = ln(2)/(halflife time)^2"
              n45 = To Double Precision Float(number=w157) -> (double precision float=w159:dbl)
              n46 = Divide "dT"(x=w159, y=w158) -> (x/y=w156:dbl)
              n47 = Square(x=w156) -> (x^2=w162:dbl)
              n48 = Negate(x=w162) -> (-x=w163:dbl)
              n49 = call <vilib>:"Sine Wave PtByPt.vi"("time"=w156, "phase"=w168, "frequency"=w169, "amplitude"=w170) -> ("sine wave"=w167:dbl)
              n50 = Divide(x=w163, y=w164) -> (x/y=w165:dbl)
              n51 = Exponential(1:w165) -> (0:w166:dbl)
              n52 = Multiply(x=w166, y=w161) -> (x*y=w160:dbl)
              n53 = Multiply(x=w167, y=w160) -> (x*y=w155:dbl)
            }
          }
          frame #1 {
            w182 = -1 items=["default"=-1, "RSE"=10083, "NRSE"=10078, "Differential"=10106, "Pseudodifferential"=12529] ("Terminal Configuration")
            w188 = 12522 items=["Finite Samples"=10178, "Continuous Samples"=10123, "Hardware Timed Single Point"=12522]  # Sample Mode
            w195 = 10106 items=["default"=-1, "RSE"=10083, "NRSE"=10078, "Differential"=10106, "Pseudodifferential"=12529] ("Terminal Configuration")
            w198 = 12522 items=["Finite Samples"=10178, "Continuous Samples"=10123, "Hardware Timed Single Point"=12522]  # Sample Mode
            # "Step 0 DeGaussing"
            # "Power Supply Control"
            # "Magnetic Flux Sensor Signals\nOnly initiated to control \ndeterministic loop"
            n54 = call-poly <vilib>:"DAQmx Create Virtual Channel.vi"("maximum value"=5.0 ("Max Voltage"), "minimum value"=0.0 ("Min Voltage"), "input terminal configuration"=w195, "physical channels"="Dev2/ai5") -> ("task out"=w196:refnum<k21>, "error out"=w197:errorcluster)  [unwired: 10 in]
            n55 = call-poly <vilib>:"DAQmx Create Virtual Channel.vi"("maximum value"=10.0, "minimum value"=-10.0, "output terminal configuration"=w182, "physical channels"="Dev2/ao0") -> ("task out"=w192:refnum<k21>, "error out"=w191:errorcluster)  [unwired: 10 in]
            n56 = call-poly <vilib>:"DAQmx Timing.vi"("task/channels in"=w196, "sample mode"=w198, "rate"=w174, "error in"=w197) -> ("task out"=w185:refnum<k21>, "error out"=w180:errorcluster)  [unwired: 10 in]
            n57 = call "Get Terminal Name with Device Prefix.vi"("error in"=w180, "Local Terminal Name"="ai/SampleClock", "task/channels in"=w185) -> ("error out"=w179:errorcluster, "Terminal Name with Device Prefix"=w178:tag, "task out"=w181:refnum<k21>)  [unwired: 6 in]
            n58 = call-poly <vilib>:"DAQmx Timing.vi"("task/channels in"=w192, "sample mode"=w188, "rate"=w174, "source"=w178, "error in"=w191) -> ("task out"=w175:refnum<k21>, "error out"=w176:errorcluster)  [unwired: 9 in]
            n59 = call <vilib>:"DAQmx Start Task.vi"("task/channels in"=w175, "error in"=w176) -> ("task out"=w187:refnum<k21>, "error out"=w186:errorcluster)  [unwired: 12 in]
            n60 = Merge Errors(w179, w186) -> (w173:errorcluster)
          }
          frame #2 {
            # "Step 0 DeGaussing"
            n61 = call-poly <vilib>:"DAQmx Create Timing Source.vi"("task/channels in"=w204, "sleep time (us)"=1.0, "error in"=w205) -> ("task out"=w201:refnum<k21>, "timing source out"=w203:string, "error out"=w199:errorcluster)  [unwired: 10 in]
            n62 = node-c288(w203, w199) -> (w208:T3)  [unwired: 8 in]
            n63 = timed-loop "DeGuassing Control" {
              tunnel: w201 -> [w231]
              tunnel: [w224] -> w210
              tunnel: w212 -> [w214]
              tunnel: [w229] -> w209
              tunnel: w199 -> [w228]
              tunnel: [w227] -> w211
              timing: w208 -> [_]
              timing-out: [_] -> w207
              tunnel: w202 -> [w216]
              i -> [w220]
              stop <- w213 continue-if-true
              # "PS does not turn off unless two values are written."
              # "Offset by 1 to eliminate\nextra datapoint at end"
              n64 = node-c288() -> ()  [unwired: 1 in, 1 out]
              n65 = Array Size(array=w216) -> (size(s)=w221:i32)
              n66 = Index Array "Index Array"(array=w216, index=w220) -> (element=w217:dbl)
              n67 = call-poly <vilib>:"DAQmx Read.vi"("task/channels in"=w231, "error in"=w228) -> ("task out"=w224:refnum<k21>, "error out"=w230:errorcluster)  [unwired: 11 in, 1 out]
              n68 = Less?(x=w220, y=w221) -> (x < y?=w219:bool)
              n69 = Subtract(x=w221, y=10) -> (x-y=w223:i32)
              n70 = Less?(x=w220, y=w223) -> (x < y?=w218:bool)
              n71 = case shown="True" w218 {
                tunnel: [0.0 ("output") w234] -> w215
                tunnel: w217 -> [_ w234]
                frame False {
                  # "Zero the AO at the end"
                }
                frame True {
                }
              }
              n72 = call-poly <vilib>:"DAQmx Write.vi"("task/channels in"=w214, "data"=w215, "error in"=w230) -> ("task out"=w229:refnum<k21>, "error out"=w227:errorcluster)  [unwired: 10 in, 1 out]
              n73 = Unbundle By Name(w227) -> ("status"=w232:bool)  [unwired: 2 out]
              n74 = Not Or(1:FALSE ("Stop"), 2:w232) -> (0:w225:bool)
              n75 = And(x=w225, y=w219) -> (x .and. y?=w213:bool)
              n76 = shared-variable "NI-GenericDesktopPC-3A84958E\\Kopco PS Project Target Variables Library.lvlib\\DeGuassing Needle"(w213) -> ()  [unwired: 1 in, 1 out]
              n77 = node-c288() -> ()  [unwired: 1 in, 1 out]
            }
            n78 = node-c288(w207) -> ()  [unwired: 1 out]
          }
          frame #3 {
            n79 = call <vilib>:"DAQmx Stop Task.vi"("task/channels in"=w246, "error in"=w247) -> ("task out"=w249:refnum<k21>, "error out"=w248:errorcluster)  [unwired: 12 in]
            n80 = call <vilib>:"DAQmx Clear Task.vi"("task in"=w249, "error in"=w248) -> ("error out"=w243:errorcluster)  [unwired: 13 in]
            n81 = call <vilib>:"DAQmx Stop Task.vi"("task/channels in"=w242, "error in"=w243) -> ("task out"=w245:refnum<k21>, "error out"=w244:errorcluster)  [unwired: 12 in]
            n82 = call <vilib>:"DAQmx Clear Task.vi"("task in"=w245, "error in"=w244) -> ()  [unwired: 13 in, 1 out]
          }
        }
      }
    }
    frame #4 {
      # "Step 0 Reset the Magnetic Sensor"
      n83 = case shown="True" "Measure Flux Sensor Zero?" {
        frame False {
        }
        frame True {
          w258 = 12522 items=["Finite Samples"=10178, "Continuous Samples"=10123, "Hardware Timed Single Point"=12522] ("sample mode")
          w272 = 3.0  # Time (s)
          w271 = 10000  # Samples read  per loop
          w291 = -1 items=["default"=-1, "RSE"=10083, "NRSE"=10078, "Differential"=10106, "Pseudodifferential"=12529] ("Terminal Configuration")
          w288 = 12522 items=["Finite Samples"=10178, "Continuous Samples"=10123, "Hardware Timed Single Point"=12522]  # Sample Mode
          w280 = 10106 items=["Default"=-1, "RSE"=10083, "NRSE"=10078, "Differential"=10106, "Pseudodifferential"=12529]  # input terminal configuration
          w283 = 0
          # "Changed on 3/29/2018 to include Sensor 2 placed in front of the needle. Added Global Variable \"Flux Calibrated Zero 2\""
          # "Reset AO to 0. Sometimes it overshoot after DeGaussing\nAdded by #WIM on 12/18/2017"
          # "Power Supply Control"
          n84 = shared-variable "NI-GenericDesktopPC-3A84958E\\Kopco PS Project Target Variables Library.lvlib\\Channels AI List"() -> (w274:string)  [unwired: 1 in, 1 out]
          n85 = shared-variable "NI-GenericDesktopPC-3A84958E\\Kopco PS Project Target Variables Library.lvlib\\Sampling Rate"() -> (w253:dbl)  [unwired: 1 in, 1 out]
          n86 = call-poly <vilib>:"DAQmx Create Virtual Channel.vi"("maximum value"=5.0, "minimum value"=0.0, "input terminal configuration"=w280, "physical channels"=w274) -> ("task out"=w254:refnum<k21>, "error out"=w255:errorcluster)  [unwired: 10 in]
          n87 = call-poly <vilib>:"DAQmx Create Virtual Channel.vi"("maximum value"=10.0, "minimum value"=-10.0, "output terminal configuration"=w291, "physical channels"="Dev2/ao0") -> ("task out"=w285:refnum<k21>, "error out"=w286:errorcluster)  [unwired: 10 in]
          n88 = call-poly <vilib>:"DAQmx Timing.vi"("task/channels in"=w254, "sample mode"=w258, "rate"=w253, "error in"=w255) -> ("task out"=w257:refnum<k21>, "error out"=w256:errorcluster)  [unwired: 10 in]
          n89 = Multiply "Total Samples \nper Channel"(x=w253, y=w272) -> (x*y=w273:dbl)
          n90 = call "Get Terminal Name with Device Prefix.vi"("error in"=w256, "Local Terminal Name"="ai/SampleClock", "task/channels in"=w257) -> ("error out"=w268:errorcluster, "Terminal Name with Device Prefix"=w267:tag, "task out"=w263:refnum<k21>)  [unwired: 6 in]
          n91 = call-poly <vilib>:"DAQmx Timing.vi"("task/channels in"=w285, "sample mode"=w288, "rate"=w253, "source"=w267, "error in"=w286) -> ("task out"=w293:refnum<k21>, "error out"=w292:errorcluster)  [unwired: 9 in]
          n92 = call <vilib>:"DAQmx Start Task.vi"("task/channels in"=w293, "error in"=w292) -> ("task out"=w296:refnum<k21>, "error out"=w295:errorcluster)  [unwired: 12 in]
          n93 = Merge Errors(w268, w295) -> (w261:errorcluster)
          n94 = Subtract "Almost Total"(x=w273, y=w271) -> (x-y=w270:dbl)
          n95 = shared-variable "NI-GenericDesktopPC-3A84958E\\Kopco PS Project Target Variables Library.lvlib\\Sensor Index Flux Core"() -> (w252:i8)  [unwired: 1 in, 1 out]
          n96 = call-poly <vilib>:"DAQmx Create Timing Source.vi"("task/channels in"=w263, "sleep time (us)"=1.0, "error in"=w261) -> ("task out"=w264:refnum<k21>, "timing source out"=w259:string, "error out"=w262:errorcluster)  [unwired: 10 in]
          n97 = Initialize Array(w283, w283) -> (w276:i32[])
          n98 = node-c288(w259) -> (w266:T3)  [unwired: 3 in]
          n99 = timed-loop {
            tunnel: w264 -> [w317]
            tunnel: w262 -> [w312]
            tunnel: [w318] -> w300
            shift-right: [w319] -> _
            shift-left: 0 -> [w320]
            tunnel: [w316] -> w294
            shift-right: [w314] -> w251
            shift-left: w276 -> [w309]
            tunnel: [w309] -> _
            tunnel: w296 -> [w313]
            tunnel: [w308] -> w301
            tunnel: w271 -> [w306]
            tunnel: w270 -> [w305]
            timing: w266 -> [_]
            timing-out: [_] -> w265
            shift-right: [w304] -> _
            shift-left: _ -> [_]
            tunnel: w252 -> [w302]
            i -> [w304]
            stop <- w303 continue-if-true
            w321 = 10.0  # timeout
            # "Magnetic Sensor 2"
            # "Magnetic Sensor 1"
            n100 = node-c288() -> ()  [unwired: 1 in, 1 out]
            n101 = call-poly <vilib>:"DAQmx Write.vi"("task/channels in"=w313, "data"=0.0, "error in"=w312) -> ("task out"=w308:refnum<k21>, "error out"=w311:errorcluster)  [unwired: 10 in, 1 out]
            n102 = call-poly <vilib>:"DAQmx Read.vi"("task/channels in"=w317, "number of samples per channel"=w306, "timeout"=w321, "error in"=w311) -> ("task out"=w316:refnum<k21>, "data"=w307:dbl[][], "error out"=w318:errorcluster)  [unwired: 9 in]
            n103 = Add(x=w320, y=w306) -> (x+y=w319:i32)
            n104 = Unbundle By Name(w318) -> ()  [unwired: 1 out]
            n105 = Less Or Equal?(x=w319, y=w305) -> (x <= y?=w303:bool)
            n106 = Delete From Array(array=w307, index (row)=w302) -> (deleted portion=w315:dbl[])  [unwired: 2 in, 1 out]
            n107 = shared-variable "NI-GenericDesktopPC-3A84958E\\Kopco PS Project Target Variables Library.lvlib\\Sensor Zero Calibrating"(w303) -> ()  [unwired: 1 in, 1 out]
            n108 = Build Array (concatenate)(w309, w315) -> (w314:dbl[])
            n109 = node-c288() -> ()  [unwired: 1 in, 1 out]
          }
          "Waveform Graph 2" <- w251
          n110 = node-c288(w265) -> ()  [unwired: 1 out]
          n111 = call <vilib>:"Std Deviation and Variance.vi"("X"=w251) -> ("mean"=w277:dbl)  [unwired: 1 in, 2 out]
          n112 = call <vilib>:"DAQmx Stop Task.vi"("task/channels in"=w301, "error in"=w300) -> ("task out"=w297:refnum<k21>, "error out"=w298:errorcluster)  [unwired: 12 in]
          n113 = shared-variable "NI-GenericDesktopPC-3A84958E\\Kopco PS Project Target Variables Library.lvlib\\Zero Flux Calibrated Core"(w277) -> ()  [unwired: 1 in, 1 out]
          n114 = call <vilib>:"DAQmx Clear Task.vi"("task in"=w297, "error in"=w298) -> ("error out"=w299:errorcluster)  [unwired: 13 in]
          n115 = call <vilib>:"DAQmx Stop Task.vi"("task/channels in"=w294, "error in"=w299) -> ("task out"=w282:refnum<k21>, "error out"=w281:errorcluster)  [unwired: 12 in]
          n116 = call <vilib>:"DAQmx Clear Task.vi"("task in"=w282, "error in"=w281) -> ("error out"=w275:errorcluster)  [unwired: 13 in]
          n117 = call <vilib>:"General Error Handler.vi"("error in (no error)"=w275) -> ()  [unwired: 10 in, 5 out]
        }
      }
    }
    frame #5 {
      # "Bound to \"Flux Calibrated Zero 2\" \nglobal Variable"
      # "Bound to \"Flux Calibrated Zero\" \nglobal Variable"
      # "Bound to \"DeGaussing Finished\""
      # "Ensure that the correct value is displayed\n(2.49±0.05 (V))"
      n118 = shared-variable "NI-GenericDesktopPC-3A84958E\\Kopco PS Project Target Variables Library.lvlib\\DeGuassing Finished"(TRUE ("DeGuassing Finished")) -> ()  [unwired: 1 in, 1 out]
    }
    frame #6 {
      # "Bound to \"Needle Selection Finished\" \nshared global variable."
      # "Step 1 Selecting Needle & Sensor\n& PID Parameters"
      n119 = while {
        tunnel: ["Proceed with Selection"] -> w333
        tunnel: ["2. Needle:"] -> w332
        tunnel: ["1. Sensor:"] -> w331
        tunnel: ["3. PID Parameters:"] -> w330
        tunnel: ["4. Aggressiveness:"] -> w329
        stop <- "Proceed with Selection" stop-if-true
        # "Added on 1/16/2018"
      }
      n120 = shared-variable "NI-GenericDesktopPC-3A84958E\\Kopco PS Project Target Variables Library.lvlib\\Needle Selection Finished"(w333) -> ()  [unwired: 1 in, 1 out]
    }
    frame #7 {
      # "Step 1 Selecting Needle & Sensor\n& PID Parameters"
      # "1/5/2018\nGot rid of \"normal\" PID Gains, Only kept Aggressive..\n\nFrom now on, that name will be dropped."
      # "Needle Used no needed so far\nbut might be used in future versinos\n12/20/2017"
      # "More precisely measured Magnetic Sensor value for Sensors 1 & 2 on 11/28/2017"
      # "Older Magnetic Sensitivity Measured before 11/2017 for Sensor 2 very crudely\n0.003112 V/GS.\nPreviously sensor 2 zero was 2.4942892 V based on 10-minute experiments on 7/12/2017"
      # "Coupled with Shared Variable Sensor 1"
      n121 = case shown="1" w342 {
        tunnel: [T1 {"proportional gain (Kc)"=0.051, "integral time (Ti, min)"=3.5e-06, "derivative time (Td, min)"=0.0} ("PID gains HyMu80 #1 (Aggressive)") T1 {"proportional gain (Kc)"=0.051, "integral time (Ti, min)"=3.5e-06, "derivative time (Td, min)"=0.0} ("PID gains HyMu80 #2 (Aggressive)")] -> w344
        tunnel: [i8 1 ("Needle Used") i8 2 ("Needle Used")] -> w345
        frame 0, Default {
          # "HyMu80#1 (Aggressive) Parameters\nModified from 0.08 to 0.075 on 4/2/2018"
          # "D"
          # "I"
          # "P"
        }
        frame 1 {
          # "D"
          # "I"
          # "P"
        }
      }
      n122 = case shown="1" w341 {
        tunnel: [0.0029794 0.0030418] -> w343
        frame 0, Default {
          (unwired) 2.4837669
          # "Zero = 2.4837669 V"
          # "Sensor #1"
          # "Sensitivity = 2.9794 mV/GS"
        }
        frame 1 {
          (unwired) 2.4928421
          # "Zero = 2.4928421 V"
          # "Sensor #2"
          # "Sensor 2 = 3.0418 mV/GS"
        }
      }
      n123 = shared-variable "NI-GenericDesktopPC-3A84958E\\Kopco PS Project Target Variables Library.lvlib\\Sensor Sensitivity Core"(w343) -> ()  [unwired: 1 in, 1 out]
      n124 = shared-variable "NI-GenericDesktopPC-3A84958E\\Kopco PS Project Target Variables Library.lvlib\\Needle Used"(w345) -> ()  [unwired: 1 in, 1 out]
    }
    frame #8 {
      w356 = "1. SET-UP & RUN \"LIVE-FAST\" image acquisition in Nikon Elements. \n2. POSITION the magnetic needle in the glycerol sample within 100 micron of several beads. (Please refer to latest calibration protocol for more details). \n3. Click OK then follow the Steps 3:\n      1. CLICK \"Start Null Flux Adjustment.\"\n      2. Adjust the Magnetic Flux until beads are no longer attacted to the needle.\n      3. Select if you want the flux to stay running until the control sequence is used in Step 4\n      3. CLICK \"FINISH Null Flux Adjustment?\" to Move to Step 4 \n"  # 1. SET-UP & RUN "LIVE-FAST" image acquisition in Nikon Elements.  2. POSITION the magnetic needle in the glycerol sample within 100 micron of several beads. (Please refer to latest calibration protocol for more details).  3. Click OK then follow the Steps 3:       1. CLICK "Start Null Flux Adjustment."       2. Adjust the Magnetic Flux until beads are no longer attacted to the needle.       3. Select if you want the flux to stay running until the control sequence is used in Step 4       3. CLICK "FINISH Null Flux Adjustment?" to Move to Step 4
      n125 = One Button Dialog(message=w356, button name ("OK")="OK!") -> ()  [unwired: 1 out]
    }
    frame #9 {
      # "Bound to \"Flux RT Control\" \nglobal shared variable?"
      # "Step 2 Finding Null Flux in Real Time"
      n126 = while {
        tunnel: ["Start Null Flux Adjustment"] -> w361
        tunnel: [w362] -> w359
        tunnel: w360 -> [w362]
        stop <- "Start Null Flux Adjustment" stop-if-true
      }
      n127 = shared-variable "NI-GenericDesktopPC-3A84958E\\Kopco PS Project Target Variables Library.lvlib\\Flux RT Control"(w361) -> ()  [unwired: 1 in, 1 out]
    }
    frame #10 {
      w378 = -1 items=["default"=-1, "RSE"=10083, "NRSE"=10078, "Differential"=10106, "Pseudodifferential"=12529] ("Terminal Configuration")
      w383 = 12522 items=["Finite Samples"=10178, "Continuous Samples"=10123, "Hardware Timed Single Point"=12522]  # Sample Mode
      w389 = 10106 items=["default"=-1, "RSE"=10083, "NRSE"=10078, "Differential"=10106, "Pseudodifferential"=12529] ("Terminal Configuration")
      w392 = 12522 items=["Finite Samples"=10178, "Continuous Samples"=10123, "Hardware Timed Single Point"=12522]  # Sample Mode
      # "Step 2 Finding Null Flux in Real Time"
      # "Hardware-Time control loop cannot keep up\nwith 50,000 Hz frequence."
      # "Power Supply Control"
      # "Magnetic Flux Sensor Signals\nRelayed over three channels."
      n128 = shared-variable "NI-GenericDesktopPC-3A84958E\\Kopco PS Project Target Variables Library.lvlib\\Channels AI List"() -> (w364:string)  [unwired: 1 in, 1 out]
      n129 = shared-variable "NI-GenericDesktopPC-3A84958E\\Kopco PS Project Target Variables Library.lvlib\\Sampling Rate"() -> (w365:dbl)  [unwired: 1 in, 1 out]
      n130 = call-poly <vilib>:"DAQmx Create Virtual Channel.vi"("maximum value"=5.0 ("Max Voltage"), "minimum value"=0.0 ("Min Voltage"), "input terminal configuration"=w389, "physical channels"=w364) -> ("task out"=w390:refnum<k21>, "error out"=w391:errorcluster)  [unwired: 10 in]
      n131 = call-poly <vilib>:"DAQmx Create Virtual Channel.vi"("maximum value"=10.0, "minimum value"=-10.0, "output terminal configuration"=w378, "physical channels"="Dev2/ao0") -> ("task out"=w386:refnum<k21>, "error out"=w385:errorcluster)  [unwired: 10 in]
      n132 = call-poly <vilib>:"DAQmx Timing.vi"("task/channels in"=w390, "sample mode"=w392, "rate"=w365, "error in"=w391) -> ("task out"=w381:refnum<k21>, "error out"=w377:errorcluster)  [unwired: 10 in]
      n133 = call "Get Terminal Name with Device Prefix.vi"("error in"=w377, "Local Terminal Name"="ai/SampleClock", "task/channels in"=w381) -> ("error out"=w374:errorcluster, "Terminal Name with Device Prefix"=w376:tag, "task out"=w371:refnum<k21>)  [unwired: 6 in]
      n134 = call-poly <vilib>:"DAQmx Timing.vi"("task/channels in"=w386, "sample mode"=w383, "rate"=w365, "source"=w376, "error in"=w385) -> ("task out"=w373:refnum<k21>, "error out"=w372:errorcluster)  [unwired: 9 in]
      n135 = call <vilib>:"DAQmx Start Task.vi"("task/channels in"=w373, "error in"=w372) -> ("task out"=w369:refnum<k21>, "error out"=w382:errorcluster)  [unwired: 12 in]
      n136 = Merge Errors(w374, w382) -> (w370:errorcluster)
    }
    frame #11 {
      w405 = 30  # # of samples pushed to PID loop
      # "Bound to \"Null Flux Running Middle\" \nshared global variable."
      # "Bound to \"Null Flux Selected\"\nshared global variable"
      # "Step 2 Finding Null Flux in Real Time"
      # "Step 2 Finding Null Flux in Real Time"
      # "12/13/2017. Cannot turn on flux control sequence inside Real-time loop. That is why I have used the trigger in the Datalogger to turn th is on. \nOtherwise, it will remain off"
      # "PID is 30 times slower"
      n137 = shared-variable "NI-GenericDesktopPC-3A84958E\\Kopco PS Project Target Variables Library.lvlib\\Zero Flux Calibrated Core"() -> (w400:dbl)  [unwired: 1 in, 1 out]
      n138 = shared-variable "NI-GenericDesktopPC-3A84958E\\Kopco PS Project Target Variables Library.lvlib\\Sensor Sensitivity Core"() -> (w398:dbl)  [unwired: 1 in, 1 out]
      n139 = call-poly <vilib>:"DAQmx Create Timing Source.vi"("task/channels in"=w413, "sleep time (us)"=1.0, "error in"=w412) -> ("task out"=w419:refnum<k21>, "timing source out"=w416:string, "error out"=w417:errorcluster)  [unwired: 10 in]
      n140 = shared-variable "NI-GenericDesktopPC-3A84958E\\Kopco PS Project Target Variables Library.lvlib\\Sensor Index Flux Core"() -> (w393:i8)  [unwired: 1 in, 1 out]
      n141 = Reciprocal(x=w396) -> (1/x=w407:dbl)
      n142 = Multiply(x=w405, y=w407) -> (x*y=w406:dbl)
      n143 = Initialize Array "Initialize Array"(0, 0 ("level 3 duration 0.1ms")) -> (w414:i32[])
      n144 = node-c288(w416, w417) -> (w423:T3)  [unwired: 8 in]
      n145 = timed-loop {
        tunnel: w419 -> [w453]
        tunnel: [w448] -> w410
        tunnel: w411 -> [w452]
        tunnel: [w450] -> w409
        tunnel: w417 -> [w449]
        tunnel: [w439] -> w408
        timing: w423 -> [_]
        timing-out: [_] -> w422
        shift-right: [w435] -> _
        shift-left: 0 -> [w445]
        shift-right: [w442] -> _
        shift-left: w414 -> [w443]
        tunnel: w405 -> [w433]
        tunnel: w406 -> [w432]
        tunnel: w400 -> [w431]
        tunnel: w398 -> [w430]
        tunnel: ["2. Adjust Magnetic Flux (GS):"] -> w404
        tunnel: [w428] -> _
        tunnel: [w428] -> w403
        tunnel: [w427] -> w402
        tunnel: w399 -> [w426]
        tunnel: [w425] -> w394
        tunnel: w393 -> [w424]
        stop <- w428 continue-if-true
        # "Observed Flux (V)"
        # "Keep this control inside the loop so that changed in \nreal time under live imaging"
        # "Flux Sensor Calibrated Zero value (V)"
        n146 = node-c288() -> ()  [unwired: 1 in, 1 out]
        n147 = call-poly <vilib>:"DAQmx Read.vi"("task/channels in"=w453, "error in"=w449) -> ("task out"=w448:refnum<k21>, "data"=w440:dbl[], "error out"=w451:errorcluster)  [unwired: 11 in]
        n148 = Delete From Array "Choose 1st Channel"(array=w440, index=w424) -> (deleted portion=w444:dbl)  [unwired: 1 in, 1 out]
        n149 = Build Array (concatenate) "AI Array"(w444, w443) -> (w441:dbl[])
        n150 = Array Size(array=w441) -> (size(s)=w447:i32)
        n151 = Equal?(x=w447, y=w433) -> (x = y?=w446:bool)
        n152 = Multiply(x="2. Adjust Magnetic Flux (GS):", y=w430) -> (x*y=w434:dbl)
        n153 = Add "Zero Offset"(x=w431, y=w434) -> (x+y=w438:dbl)
        n154 = case shown="True" w446 {
          tunnel: w432 -> [_ w466]
          tunnel: w438 -> [_ w471]
          tunnel: [w464 w469] -> w435
          tunnel: w445 -> [w464 _]
          tunnel: w441 -> [w463 w468]
          tunnel: [w463 w467] -> w442
          tunnel: w426 -> [_ w465]
          frame False {
          }
          frame True {
            # "Max/Min controller outputs"
            n155 = call-poly <vilib>:"Mean.vi"("X"=w468) -> ("mean"=w470:dbl)  [unwired: 1 out]
            n156 = call-poly <vilib>:"PID.vi"("reinitialize? (F)"=FALSE, "output range"=cluster{"output high":dbl, "output low":dbl} {"output high"=10.0, "output low"=-10.0}, "dt (s)"=w466, "PID gains"=w465, "process variable"=w470, "setpoint"=w471) -> ("output"=w469:dbl)  [unwired: 4 in, 1 out]
            n157 = Initialize Array(0, 0) -> (w467:i32[])
          }
        }
        n158 = case shown="True" "4. Click Rocker to finish Null Flux Adjustment" {
          tunnel: [w455 TRUE ("y")] -> w436
          tunnel: [w456 w458] -> w425
          tunnel: w435 -> [w456 w459]
          tunnel: [w455 "3. Keep Null Flux Running \n       Until Next Step?"] -> w427
          frame False {
            w455 = FALSE ("y")
          }
          frame True {
            # "A Toggle fixed the problem!"
            n159 = case shown="True" "3. Keep Null Flux Running \n       Until Next Step?" {
              tunnel: [0.0 ("output") w462] -> w458
              tunnel: w459 -> [_ w462]
              frame False {
                # "Reset AO at the end"
              }
              frame True {
                # "Keep Flux the same"
              }
            }
          }
        }
        n160 = call-poly <vilib>:"DAQmx Write.vi"("task/channels in"=w452, "data"=w425, "error in"=w451) -> ("task out"=w450:refnum<k21>, "error out"=w439:errorcluster)  [unwired: 10 in, 1 out]
        n161 = Unbundle By Name(w439) -> ("status"=w454:bool)  [unwired: 2 out]
        n162 = Not Or(1:w436, 2:w454) -> (0:w428:bool)
        n163 = node-c288() -> ()  [unwired: 1 in, 1 out]
      }
      n164 = Not(x=w403) -> (.not. x?=w401:bool)
      n165 = node-c288(w422) -> ()  [unwired: 1 out]
      n166 = shared-variable "NI-GenericDesktopPC-3A84958E\\Kopco PS Project Target Variables Library.lvlib\\Null Flux Running Middle"(w402) -> ()  [unwired: 1 in, 1 out]
      n167 = shared-variable "NI-GenericDesktopPC-3A84958E\\Kopco PS Project Target Variables Library.lvlib\\Zero Flux Observed GS"(w404) -> ()  [unwired: 1 in, 1 out]
      n168 = shared-variable "NI-GenericDesktopPC-3A84958E\\Kopco PS Project Target Variables Library.lvlib\\Null Flux Selected"(w401) -> ()  [unwired: 1 in, 1 out]
      n169 = shared-variable "NI-GenericDesktopPC-3A84958E\\Kopco PS Project Target Variables Library.lvlib\\Flux RT Control"(w403) -> ()  [unwired: 1 in, 1 out]
    }
    frame #12 {
      # "Zeroing the PS Output at the end with a STOP botton.\nReplacing it with a Toggle seemed to do the trick.\n \nSwitch the toggle \"mechanical action\" to \n\"Latch when Released\" so that it will reset to FALSE \nat the end every time."
      n170 = call <vilib>:"DAQmx Stop Task.vi"("task/channels in"=w488, "error in"=w486) -> ("task out"=w493:refnum<k21>, "error out"=w492:errorcluster)  [unwired: 12 in]
      n171 = call <vilib>:"DAQmx Clear Task.vi"("task in"=w493, "error in"=w492) -> ("error out"=w489:errorcluster)  [unwired: 13 in]
      n172 = call <vilib>:"DAQmx Stop Task.vi"("task/channels in"=w487, "error in"=w489) -> ("task out"=w491:refnum<k21>, "error out"=w490:errorcluster)  [unwired: 12 in]
      n173 = call <vilib>:"DAQmx Clear Task.vi"("task in"=w491, "error in"=w490) -> ()  [unwired: 13 in, 1 out]
    }
    frame #13 {
      w498 = "1. REMOVE the needle from the sample (if needed).\n2. PREPARE for the next experiment.\n3. Click OK in this dialog box!\n4. ENTER the required variables here: (Flux Setpoint & Number of Cycles, & Length of Pre-and Post-Periods of Null Flux). Click \"Proceed with these Parameters.\"\n5. OPEN Data Logger (if you have not done so), ENTER file name, and RUN program. \n6. ADJUST the number of frames in the Fast Timelapse Macro (if a macro is used). Otherwise, skip this step. \n7. RUN the macro (if a macro is used). Otherwise, click \"TRGR\" button in Nikon Elements to initiate Fast Timelapse Image Capture, Data Acquisition, and PID-Controlled Sequence.\n"  # 1. REMOVE the needle from the sample (if needed). 2. PREPARE for the next experiment. 3. Click OK in this dialog box! 4. ENTER the required variables here: (Flux Setpoint & Number of Cycles, & Length of Pre-and Post-Periods of Null Flux). Click "Proceed with these Parameters." 5. OPEN Data Logger (if you have not done so), ENTER file name, and RUN program.  6. ADJUST the number of frames in the Fast Timelapse Macro (if a macro is used). Otherwise, skip this step.  7. RUN the macro (if a macro is used). Otherwise, click "TRGR" button in Nikon Elements to initiate Fast Timelapse Image Capture, Data Acquisition, and PID-Controlled Sequence.
      # "AO values of current"
      n174 = One Button Dialog(message=w498, button name ("OK")="OK!") -> ()  [unwired: 1 out]
    }
    frame #14 {
      # "AO values of current"
      # "Bound to \"PID Parameters Selected\"\nshared global variable"
      # "Step 3 Specifying Waveform Parameters"
      # "Step 3 Specifying Waveform Parameters"
      n175 = while {
        tunnel: ["Proceed with Parameters"] -> w509
        tunnel: ["Flux ON relative setpoint (Gs)"] -> w508
        tunnel: [w510] -> w507
        tunnel: ["Number of Cycles"] -> w506
        tunnel: ["Pre-Wave Null Flux Interval (s)"] -> w505
        tunnel: ["Post-Wave Null Flux Interval (s)"] -> w504
        tunnel: ["OFF (s)"] -> w500
        tunnel: ["ON"] -> w499
        stop <- "Proceed with Parameters" stop-if-true
        # "Updated code on \nto vary ON/OFF cycle"
        # "You can use a #negative #sign to go to the opposite end\nto extend the linear range if neeed."
        # "Changed Cycles type from double\nto integer-16bit on 1/8/2018"
        # "Global variables were moved inside this while loop to resolve\nthe problem of updating them. For whatever reason, LabVIEW\nseems to only pass to the variable the previous values but \nnot the updated ones for variable (but passes the updated version for \nan indicator). Verified on 1/8/2018 by #WIM"
        n176 = shared-variable "NI-GenericDesktopPC-3A84958E\\Kopco PS Project Target Variables Library.lvlib\\Cycles"("Number of Cycles") -> ()  [unwired: 1 in, 1 out]
        n177 = Add "Total Period Time (s)"(x="OFF (s)", y="ON") -> (x+y=w510:dbl)
        n178 = shared-variable "NI-GenericDesktopPC-3A84958E\\Kopco PS Project Target Variables Library.lvlib\\Flux Setpoint ON Gs Relative"("Flux ON relative setpoint (Gs)") -> ()  [unwired: 1 in, 1 out]
        n179 = shared-variable "NI-GenericDesktopPC-3A84958E\\Kopco PS Project Target Variables Library.lvlib\\Null Flux Post Period"("Post-Wave Null Flux Interval (s)") -> ()  [unwired: 1 in, 1 out]
        n180 = shared-variable "NI-GenericDesktopPC-3A84958E\\Kopco PS Project Target Variables Library.lvlib\\Null Flux Pre Period"("Pre-Wave Null Flux Interval (s)") -> ()  [unwired: 1 in, 1 out]
        n181 = shared-variable "NI-GenericDesktopPC-3A84958E\\Kopco PS Project Target Variables Library.lvlib\\Period Per Cycle"(w510) -> ()  [unwired: 1 in, 1 out]
      }
      n182 = shared-variable "NI-GenericDesktopPC-3A84958E\\Kopco PS Project Target Variables Library.lvlib\\Control Parameters Selected"(w509) -> ()  [unwired: 1 in, 1 out]
    }
    frame #15 {
      (unwired) 1.0 ("Double")
      w561 = 0 ("index")
      w590 = u32 1000  # ms/sec
      w600 = bool[] []  # Initial Empty Array
      w604 = 747.0  # K_Prime
      w607 = 13.91  # V_max
      w608 = 1.9431  # h
      w643 = dbl[] []  # Initial Zero Array
      w625 = 0.031  # Time Length (s)
      w674 = FALSE
      w656 = bool[] []  # Initial Empty Array
      w685 = dbl[] []  # Initial Zero Array
      # "Post Wave might need to be\nfixed with Ramp"
      # "No need for this"
      # "Number of Cycles"
      # "ON per Cycle (s)"
      # "OFF per Cycle (s)"
      # "Corrected Null Flux/OFF Observed (Gs):\n2nd Cycle OFF & Later & Postwave Corrected"
      # "1/4 wave to get the main points of the\n mini DeGauss waveform 3/12/2018"
      # "AO values of current"
      # "Into the Data Logger"
      # "Null Flux Observed:\n2nd Cycle OFF & Later & Postwave Corrected(V)"
      # "Null Flux Observed:\nPrewave & 1st Cycle OFF Uncorrected (V)\nNO CHANGE!"
      # "Initial Null Flux Observed (Gs)"
      # "5. Based on a sigmoidal curve fit 2019-08-08\nThe Equation is Y = Vmax * X^h /(K_prime + X^h), where Vmax = 13.91, h = 1.9431, and Kprime = 747"
      # "# of samples of Mini DeGauss"
      # "Three choices for mini DeGauss\nwaveform? \n0.030 ms @ 500 Hz   (No AI leakage at \nhigher fluxes ~ 200 Gs. Moreoever, flux\nvariation is higher = more atoms are recruited)\n0.030 ms @ 1000 Hz\n0.015 ms @ 1000 Hz"
      # "Added 3/12/2018"
      # "Amplitude will need to be modified later"
      # "OFF = 2 * 1/2 Cycle - samples of ON Mini DeGauss"
      # "30,000 @ 500 Hz\n\n1000 Hz for PID \nsampling rate of 1 ms\ncreate aliasing/roundoff error\n\nSampling at higher rate, and then\nchoose your points of interest"
      # "OFF = - samples of ON Mini DeGauss"
      # "Period per Cycle (s)"
      # "Flux Setpoint/On (V)"
      # "Flux Relative ON Setpoint (Gs)"
      # "Step 3 Building Waveforms for PID control and for mini-DeGauss Cycles"
      # "Step 3 Creating Waveforms"
      # "1/4/2018. It checks the maximum of either the observed zero or the \nsuperimposed ON setpoints for my OFF/ON square wave"
      # "ON/OFF PID Parameters. In order for this to work, the OFF flux needs to be near the linear range."
      # "Note: Max point is included in that given PID Gain schedule. it is the cut-off point"
      # "I was able to build a PID gain schedule by matching the types.\nThis way I will be able to customize the values based on sensor sensitivities\nand so forth 1/2/2017."
      # "Corrected on 1/4/2018"
      # "N cycles of High/Low\nCreate A Control Array in terms \nof flux sensor voltage"
      n183 = shared-variable "NI-GenericDesktopPC-3A84958E\\Kopco PS Project Target Variables Library.lvlib\\Sampling Rate"() -> (w519:dbl)  [unwired: 1 in, 1 out]
      n184 = shared-variable "NI-GenericDesktopPC-3A84958E\\Kopco PS Project Target Variables Library.lvlib\\Zero Flux Observed GS"() -> (w596:dbl)  [unwired: 1 in, 1 out]
      n185 = To Quad Integer(1:w519) -> (0:w518:i64)
      n186 = Absolute Value(x=w601) -> (abs(x)=w599:dbl)
      n187 = shared-variable "NI-GenericDesktopPC-3A84958E\\Kopco PS Project Target Variables Library.lvlib\\Sensor Sensitivity Core"() -> (w539:dbl)  [unwired: 1 in, 1 out]
      n188 = Divide "ms to sec"(x="Ramp Total Interval (ms)", y=w590) -> (x/y=w589:dbl)
      n189 = shared-variable "NI-GenericDesktopPC-3A84958E\\Kopco PS Project Target Variables Library.lvlib\\Zero Flux Observed GS"() -> (w584:dbl)  [unwired: 1 in, 1 out]
      n190 = Power Of X "X^h"(1:w599, 2:w608) -> (0:w605:dbl)
      n191 = shared-variable "NI-GenericDesktopPC-3A84958E\\Kopco PS Project Target Variables Library.lvlib\\Ramp Total Interval (ms)"("Ramp Total Interval (ms)") -> ()  [unwired: 1 in, 1 out]
      n192 = shared-variable "NI-GenericDesktopPC-3A84958E\\Kopco PS Project Target Variables Library.lvlib\\Ramp Steps"("# Ramp Steps") -> ()  [unwired: 1 in, 1 out]
      n193 = Multiply(x=w607, y=w605) -> (x*y=w606:dbl)
      n194 = Add(x=w605, y=w604) -> (x+y=w603:dbl)
      n195 = Divide "Shift in Null Flux Observed (Gs)"(x=w606, y=w603) -> (x/y=w602:dbl)
      n196 = shared-variable "NI-GenericDesktopPC-3A84958E\\Kopco PS Project Target Variables Library.lvlib\\Flux Setpoint ON Gs Relative"() -> (w571:dbl)  [unwired: 1 in, 1 out]
      n197 = Add "Correcting Null Flux Observed (Gs)"(x=w602, y=w596) -> (x+y=w585:dbl)
      n198 = shared-variable "NI-GenericDesktopPC-3A84958E\\Kopco PS Project Target Variables Library.lvlib\\Zero Flux Observed Gs Corrected"(w585) -> ()  [unwired: 1 in, 1 out]
      n199 = Multiply "# Total ramp\nSamples"(x=w589, y=w518) -> (x*y=w593:dbl)
      n200 = shared-variable "NI-GenericDesktopPC-3A84958E\\Kopco PS Project Target Variables Library.lvlib\\Sensor Sensitivity Core"() -> (w540:dbl)  [unwired: 1 in, 1 out]
      n201 = Multiply "# of Samples"(x=w625, y=w518) -> (x*y=w615:dbl)
      n202 = Divide(x=750.0, y=900.0) -> (x/y=w614:dbl)
      n203 = To Unsigned Long Integer(number=w615) -> (unsigned 32bit integer=w609:u32)
      n204 = To Unsigned Long Integer "# total ramp\nsamples (int)"(number=w593) -> (unsigned 32bit integer=w574:u32)
      n205 = Multiply(x=w615, y=w614) -> (x*y=w611:dbl)
      n206 = Subtract "Uncorrected to Corrected\n OFF Shift (Gs)"(x=w585, y=w584) -> (x-y=w572:dbl)
      n207 = for "One Mini DeGauss Cycle" {
        N: w609 -> [_]
        tunnel: w518 -> [w736]
        tunnel: [w752] -> w635 mode=indexing
        tunnel: w625 -> [w737]
        tunnel: [w736] -> w624
        tunnel: [w735] -> w623
        i -> [w751]
        w740 = 7.5  # amplitude
        w742 = 1.0  # Starting Amplitude
        w756 = 90.0  # Phase, Deg
        w735 = u64 480  # Frequency, Hz
        # "It seems 0.3 * Time will give \na decay around 20 ms."
        # "samples/sec"
        n208 = To Double Precision Float(number=w751) -> (double precision float=w753:dbl)
        n209 = Multiply(x=w737, y=0.3) -> (x*y=w738:dbl)
        n210 = Divide(x=w753, y=w736) -> (x/y=w747:dbl)
        n211 = Square(x=w747) -> (x^2=w749:dbl)
        n212 = Square(x=w738) -> (x^2=w745:dbl)
        n213 = Natural Logarithm(1:2.0 ("x")) -> (0:w743:dbl)
        n214 = Divide(x=w743, y=w745) -> (x/y=w744:dbl)
        n215 = Negate(x=w749) -> (-x=w748:dbl)
        n216 = Multiply(x=w748, y=w744) -> (x*y=w754:dbl)
        n217 = call <vilib>:"Sine Wave PtByPt.vi"("time"=w747, "phase"=w756, "frequency"=w735, "amplitude"=w740) -> ("sine wave"=w741:dbl)
        n218 = Exponential "Exp(-t^2*k)"(1:w754) -> (0:w755:dbl)
        n219 = Multiply(x=w755, y=w742) -> (x*y=w750:dbl)
        n220 = Multiply(x=w741, y=w750) -> (x*y=w752:dbl)
      }
      n221 = Increment "Make one extra to trim"(x="# Ramp Steps") -> (x+1=w583:u32)
      n222 = To Unsigned Long Integer(number=w611) -> (unsigned 32bit integer=w610:u32)
      n223 = Multiply "OFF (Corrected)\nGs to V"(x=w585, y=w539) -> (x*y=w597:dbl)
      n224 = Multiply "OFF (Uncorrected) \nGs to V"(x=w596, y=w539) -> (x*y=w586:dbl)
      n225 = Divide "Jump/Step \nON to Uncorrected \nOFF (Gs)"(x=w571, y="# Ramp Steps") -> (x/y=w573:dbl)
      n226 = Multiply "ON\nGs to V"(x=w601, y=w539) -> (x*y=w664:dbl)
      n227 = Quotient & Remainder "Samples # \nper step"(x=w574, y="# Ramp Steps") -> (floor(x/y)=w568:u32)  [unwired: 1 out]
      n228 = Add "ON + Offset from \nObserved Zero (V)"(x=w586, y=w664) -> (x+y=w684:dbl)
      n229 = case "Correct Null \nFlux?" shown="False" "7. Correct Null Flux after Cycle #1?" {
        tunnel: [w725 w727] -> w527
        tunnel: w597 -> [_ w727]
        tunnel: w586 -> [w725 _]
        tunnel: [w724 w726] -> w588
        tunnel: w596 -> [w724 _]
        tunnel: w585 -> [_ w726]
        frame False {
          # "ON"
          # "OFF"
          # "Uncorrected"
        }
        frame True {
          # "Corrected"
        }
      }
      "Corrective \nNull Flux (Gs)" <- w588
      n230 = Subtract "Jump ON to \nCorrected OFF (Gs)"(x=w571, y=w572) -> (x-y=w569:dbl)
      n231 = Divide "Jump/Step\nON to Corrected\nOFF (Gs)"(x=w569, y="# Ramp Steps") -> (x/y=w570:dbl)
      n232 = for "Create Ramp Steps" {
        N: w583 -> [_]
        shift-right: [w721] -> w562
        shift-left: dbl[] [] -> [w723]
        tunnel: w585 -> [w707]
        tunnel: w584 -> [w706]
        tunnel: w540 -> [w713]
        shift-right: [w718] -> w567
        shift-left: dbl[] [] -> [w717]
        tunnel: [w712] -> w560
        tunnel: w568 -> [w712]
        tunnel: w573 -> [w711]
        tunnel: w570 -> [w710]
        i -> [w714]
        n233 = To Double Precision Float(number=w714) -> (double precision float=w716:dbl)
        n234 = Multiply "Going thru\nSteps"(x=w716, y=w710) -> (x*y=w715:dbl)
        n235 = Multiply "Going thru\nSteps"(x=w716, y=w711) -> (x*y=w720:dbl)
        n236 = Add "UnCorrected Null flux Offset"(x=w720, y=w706) -> (x+y=w709:dbl)
        n237 = Add "Corrected Null Flux\nOffset"(x=w715, y=w707) -> (x+y=w708:dbl)
        n238 = Multiply "V to Gs"(x=w709, y=w713) -> (x*y=w705:dbl)
        n239 = Multiply "V to Gs"(x=w713, y=w708) -> (x*y=w704:dbl)
        n240 = Initialize Array "Current \nStep"(w705, w712) -> (w722:dbl[])
        n241 = Initialize Array "Current \nStep"(w704, w712) -> (w719:dbl[])
        n242 = Build Array (concatenate) "Uncorrected OFF\n to ON Ramp (V)"(w723, w722) -> (w721:dbl[])
        n243 = Build Array (concatenate) "Corrected OFF \nto ON Ramp (V)"(w717, w719) -> (w718:dbl[])
      }
      n244 = Multiply "# samples: OFF"(x=w518, y=w520) -> (x*y=w578:dbl)
      n245 = Multiply "# samples ON"(x=w518, y=w595) -> (x*y=w582:dbl)
      n246 = Multiply "Pre-wave Zero Inteval Samples"(x=w669, y=w518) -> (x*y=w682:dbl)
      n247 = Multiply "Post-wave Zero Interval Samples"(x=w668, y=w518) -> (x*y=w526:dbl)
      n248 = Reciprocal "period (s)"(x=w623) -> (1/x=w620:dbl)
      n249 = To Quad Integer(1:w526) -> (0:w524:i64)
      n250 = To Quad Integer(1:w682) -> (0:w525:i64)
      n251 = Multiply "Samples/wave"(x=w624, y=w620) -> (x*y=w621:dbl)
      n252 = Quotient & Remainder "1/4 wave"(x=w621, y=u8 4) -> (floor(x/y)=w617:dbl)  [unwired: 1 out]
      n253 = To Unsigned Long Integer(number=w617) -> (unsigned 32bit integer=w616:u32)
      n254 = Reverse 1D Array "ON to Uncorrected OFF"(array=w562) -> (reversed array=w566:dbl[])
      n255 = Reverse 1D Array "ON to corrected OFF"(array=w567) -> (reversed array=w565:dbl[])
      n256 = Delete From Array "Remove ON"(array=w566, length=w560, index=w561) -> (array with subset deleted=w551:dbl[])  [unwired: 1 out]
      n257 = Delete From Array "Remove ON"(array=w565, length=w560, index=w561) -> (array with subset deleted=w530:dbl[])  [unwired: 1 out]
      n258 = Delete From Array "Remove First \ncorrected OFF step\nto ON"(array=w567, length=w560, index=w561) -> (array with subset deleted=w552:dbl[])  [unwired: 1 out]
      n259 = Delete From Array "Remove First \nUncorrected OFF step\nto ON"(array=w562, length=w560, index=w561) -> (array with subset deleted=w559:dbl[])  [unwired: 1 out]
      n260 = Array Size(array=w559) -> (size(s)=w576:i32)
      n261 = Array Size(array=w530) -> (size(s)=w555:i32)
      n262 = Array Size(array=w552) -> (size(s)=w558:i32)
      n263 = Array Size(array=w551) -> (size(s)=w553:i32)
      n264 = Decrement "last item"(x=w576) -> (x-1=w575:i32)
      n265 = Array Size "Size ON Ramp"(array=w530) -> (size(s)=w554:i32)
      n266 = Array Size "Size OFF Ramp"(array=w552) -> (size(s)=w532:i32)
      n267 = Decrement "last item"(x=w558) -> (x-1=w557:i32)
      n268 = Decrement "last item"(x=w555) -> (x-1=w547:i32)
      n269 = Decrement "last item"(x=w553) -> (x-1=w548:i32)
      n270 = Index Array "ON"(array=w559, index=w575) -> (element=w581:dbl)
      n271 = Index Array "ON"(array=w552, index=w557) -> (element=w580:dbl)
      n272 = Index Array "Corrected OFF"(array=w530, index=w547) -> (element=w528:dbl)
      n273 = Index Array "Uncorrected OFF"(array=w551, index=w548) -> (element=w579:dbl)
      n274 = Subtract "OFF Ramp Samples #"(x=w578, y=w532) -> (x-y=w564:dbl)
      n275 = Subtract "ON Ramp Samples #"(x=w582, y=w554) -> (x-y=w563:dbl)
      n276 = Subtract "Post-Wave OFF Sample #"(x=w524, y=w532) -> (x-y=w529:i64)
      n277 = Initialize Array "Extend PostOFF"(w528, w529) -> (w531:dbl[])
      n278 = Initialize Array "Extend OFF"(w528, w564) -> (w549:dbl[])
      n279 = Initialize Array "Extend ON"(w581, w563) -> (w577:dbl[])
      n280 = Initialize Array "Extend OFF"(w579, w564) -> (w550:dbl[])
      n281 = Initialize Array "Extend ON"(w580, w563) -> (w556:dbl[])
      n282 = Build Array (concatenate) "ON to Corrected OFF (V) First Step Removed\nPost-Wave"(w530, w531) -> (w521:dbl[])
      n283 = Build Array (concatenate) "UnCorrected OFF\n to ON (V)\nFirst Step Removed"(w559, w577) -> (w543:dbl[])
      n284 = Build Array (concatenate) "ON to UnCorrected OFF (V)\nFirst Step Removed"(w551, w550) -> ()  [unwired: 1 out]
      n285 = Build Array (concatenate) "Corrected OFF\n to ON (V)\nFirst Step Removed"(w552, w556) -> (w542:dbl[])
      n286 = Build Array (concatenate) "ON to Corrected OFF (V)\nFirst Step Removed"(w530, w549) -> (w522:dbl[])
      n287 = case "Force Step Ramps" shown="True" "9.            Step(s) Force Ramp in              (ms)?" {
        tunnel: [w690 w700] -> w546
        tunnel: w684 -> [w693 _]
        tunnel: [w691 w699] -> w544
        tunnel: [w689 w703] -> w545
        tunnel: w586 -> [w695 w698]
        tunnel: w527 -> [w696 _]
        tunnel: w582 -> [w692 _]
        tunnel: w578 -> [w694 w702]
        tunnel: w542 -> [_ w699]
        tunnel: w543 -> [_ w701]
        tunnel: w522 -> [_ w700]
        tunnel: [w691 w701] -> w541
        tunnel: w521 -> [_ w697]
        tunnel: w527 -> [w688 _]
        tunnel: w524 -> [w687 _]
        tunnel: [w686 w697] -> w523
        frame False {
          # "OFF: 1st cycle"
          # "ON: all cycles"
          # "OFF: 2nd cycle\n& Later"
          # "NO RAMP"
          # "OFF (corrected) to ON (V)"
          # "OFF (Uncorrected) to ON (V)"
          # "ON + Offset from \nObserved Zero (V)"
          n288 = Initialize Array "Post Wave"(w688, w687) -> (w686:dbl[])
          n289 = Initialize Array "1. corrected OFF"(w696, w694) -> (w690:dbl[])
          n290 = Initialize Array "1.  Uncorrected OFF"(w695, w694) -> (w689:dbl[])
          n291 = Initialize Array "2. ON"(w693, w692) -> (w691:dbl[])
        }
        frame True {
          # "OFF: Post-wave Zero"
          # "OFF: 1st cycle"
          # "OFF: 2nd Cycle & Later"
          # "ON: 2nd Cycle & Later"
          # "ON: 1st cycle"
          # "2. On to corrected OFF (V)"
          # "1. uncorrected OFF to ON (V)"
          # "WITH Steps RAMP"
          # "1. corrected OFF to ON (V)"
          n292 = Initialize Array "1. Uncorrected OFF"(w698, w702) -> (w703:dbl[])
        }
      }
      n293 = Subtract(x=w578, y=w609) -> (x-y=w644:dbl)
      n294 = Initialize Array "1. Off"(FALSE, w578) -> (w679:bool[])
      n295 = Initialize Array "2. On"(TRUE, w582) -> (w678:bool[])
      n296 = Initialize Array "2. Off"(0.0 ("dimension size"), w644) -> (w646:dbl[])
      n297 = Initialize Array "2. Off"(FALSE, w644) -> (w662:bool[])
      n298 = Initialize Array "2. Off"(FALSE, w578) -> (w632:bool[])
      n299 = Initialize Array "1. On"(TRUE, w582) -> (w663:bool[])
      n300 = Initialize Array "2. Off"(0.0 ("dimension size"), w578) -> (w630:dbl[])
      n301 = Build Array (concatenate) "1st Cycle\nOne cycle: OFF/ON"(w545, w541) -> (w538:dbl[])
      n302 = Build Array (concatenate) "2nd Cycle & later\nOne Cycle: OFF/ON"(w546, w544) -> (w537:dbl[])
      n303 = Build Array (concatenate) "Magnetic Flux Control\nWaveform OFF/ON? Array"(w679, w678) -> (w675:bool[])
      n304 = Build Array (concatenate) "Mini DeGauss\nAO Waveform Array"(w635, w646) -> (w634:dbl[])
      n305 = To Quad Integer(1:w525) -> (0:w629:i64)
      n306 = Build Array (concatenate) "Mini DeGauss\nWaveform OFF/ON? Array"(w663, w662) -> (w659:bool[])
      n307 = Less?(x=w524, y=w609) -> (x < y?=w647:bool)
      n308 = Less?(x=w629, y=w609) -> (x < y?=w628:bool)
      n309 = case "Pre-Mini DeGauss?" shown="True" w628 {
        tunnel: [w728 w734] -> w627
        tunnel: w629 -> [w729 _]
        tunnel: [w730 w733] -> w626
        frame False {
          # "Modified mini DeGauss to not include it in the \npre-wave on 3/9/2018"
          n310 = Initialize Array "Off"(0.0 ("dimension size"), w729) -> (w730:dbl[])
          n311 = Initialize Array "Off"(FALSE, w729) -> (w728:bool[])
        }
        frame True {
          w733 = dbl[] []  # Initial Zero Array
          w734 = bool[] []  # Initial Empty Array
          # "Pre-wave is smaller than the \nmini-DeGauss cycle"
        }
      }
      n312 = case "Post-Mini DeGauss" shown="False" w647 {
        tunnel: [w764 w770] -> w655
        tunnel: w524 -> [w763 _]
        tunnel: w609 -> [w762 _]
        tunnel: w635 -> [w759 _]
        tunnel: [w757 w769] -> w636
        frame False {
          n313 = Subtract(x=w763, y=w762) -> (x-y=w758:i64)
          n314 = Initialize Array "2. Off"(0.0 ("dimension size"), w758) -> (w761:dbl[])
          n315 = Initialize Array "1. On"(TRUE, w762) -> (w768:bool[])
          n316 = Initialize Array "2. Off"(FALSE, w758) -> (w767:bool[])
          n317 = Build Array (concatenate) "Mini DeGauss\nWaveform OFF/ON? Array"(w759, w761) -> (w757:dbl[])
          n318 = Build Array (concatenate) "Post-Mini DeGauss\nWave"(w768, w767) -> (w764:bool[])
        }
        frame True {
          w769 = dbl[] []  # Initial Zero Array
          w770 = bool[] []  # Initial Empty Array
          # "Post-wave is smaller than the \nmini-DeGauss cycle"
        }
      }
      n319 = for "Building N Cycles of OFF/ON Wavefform" {
        N: w670 -> [_]
        tunnel: w537 -> [w777]
        shift-right: [w775] -> w536
        shift-left: w685 -> [w778]
        shift-right: [w790] -> w673
        shift-left: w656 -> [w792]
        tunnel: w675 -> [w791]
        shift-right: [w789] -> w648
        shift-left: w600 -> [w788]
        tunnel: w659 -> [w787]
        shift-right: [w786] -> w642
        shift-left: w643 -> [w784]
        tunnel: w634 -> [w785]
        tunnel: w632 -> [w780]
        tunnel: w630 -> [w779]
        tunnel: w538 -> [w776]
        i -> [w783]
        n320 = Equal? "First Cycle?"(x=0, y=w783) -> (x = y?=w781:bool)
        n321 = case "First Cycle?" shown="True" w781 {
          tunnel: [w801 w806] -> w789
          tunnel: w788 -> [w800 _]
          tunnel: w787 -> [w799 _]
          tunnel: [w798 w805] -> w786
          tunnel: w785 -> [w797 _]
          tunnel: w784 -> [w796 _]
          tunnel: w780 -> [_ w806]
          tunnel: w779 -> [_ w805]
          tunnel: w778 -> [w795 w804]
          tunnel: [w794 w802] -> w775
          tunnel: w777 -> [w793 _]
          tunnel: w776 -> [_ w803]
          frame False {
            n322 = Build Array (concatenate) "Build Array"(w800, w799) -> (w801:bool[])
            n323 = Build Array (concatenate) "Corrected"(w795, w793) -> (w794:dbl[])
            n324 = Build Array (concatenate) "Build Array"(w796, w797) -> (w798:dbl[])
          }
          frame True {
            n325 = Build Array (concatenate) "Uncorrected"(w804, w803) -> (w802:dbl[])
          }
        }
        n326 = Build Array (concatenate) "Build Array"(w792, w791) -> (w790:bool[])
      }
      n327 = Initialize Array "Pre-Wave"(w586, w629) -> (w594:dbl[])
      n328 = Initialize Array "Pre-Wave Zero"(w674, w629) -> (w658:bool[])
      n329 = Initialize Array "Post Wave Zero"(w674, w524) -> (w657:bool[])
      n330 = Build Array (concatenate) "Mini-DeGauss  \n Waveform OFF/ON? Array"(w627, w648, w655) -> (w652:bool[])
      n331 = Build Array (concatenate) "Mini-DeGauss  \n Waveform AO Sequence"(w626, w642, w636) -> (w640:dbl[])
      n332 = Build Array (concatenate) "Magnetic Flux \nControl Waveform OFF/ON? Array"(w658, w673, w657) -> (w672:bool[])
      n333 = Array Size(array=w640) -> (size(s)=w641:i32)
      n334 = Multiply "Samples/cycle"(x=w518, y=w671) -> (x*y=w683:dbl)
      n335 = Array Size(array=w652) -> (size(s)=w653:i32)
      n336 = Add "Pre & Post Samples"(x=w629, y=w524) -> (x+y=w681:i64)
      n337 = Build Array (concatenate) "Magnetic Flux \nControl Array"(w594, w536, w523) -> (w535:dbl[])
      n338 = Initialize Array "1. Off"(0.0, w641) -> (w638:dbl[])
      n339 = Initialize Array "1. Off"(FALSE, w653) -> (w650:bool[])
      n340 = Multiply "Total Number of OFF/ON Samples"(x=w683, y=w670) -> (x*y=w619:dbl)
      n341 = To Unsigned Long Integer(number=w619) -> (unsigned 32bit integer=w618:u32)
      n342 = case "Mini DeGauss? YES/NO?" shown="False" "6. Mini DeGauss cycles in OFF segments?" {
        tunnel: w652 -> [_ w774]
        tunnel: [w772 w774] -> w651
        tunnel: w650 -> [w772 _]
        tunnel: w640 -> [_ w773]
        tunnel: w638 -> [w771 _]
        tunnel: [w771 w773] -> w637
        frame False {
          # "NO mini\nDeGauss \ncycles"
        }
        frame True {
          # "Mini DeGauss\ncycles"
        }
      }
      n343 = Add "Total # of Samples"(x=w618, y=w681) -> (x+y=w680:i64)
    }
    frame #16 {
      # "1/4 wave to get the main points of the\n mini DeGauss waveform 3/12/2018"
      # "# of samples of Mini DeGauss"
      # "Flux ON/OFF Logical"
      # "Sampling Rate"
      # "Flux Control Sequence"
      # "Mini DeGauss AO Sequence, Normalized"
      # "Mini DeGauss Logical"
      # "AO values of current"
      # "1 for #1\n2 for #2"
      # "#WIM 1/16/2018\nPID Aggressiveness\n0 = Optimized\n1 = Minimum\n2 = Average\n3 = Maximum"
      # "Step 4 Specifying PID Parameters"
      # "Total Number of Samples"
      # "#WIM 1/10/2018\nPID Parameters List Selection:\n0 = Fixed Schedule\n1 = Interpolated Schedule"
      n344 = shared-variable "NI-GenericDesktopPC-3A84958E\\Kopco PS Project Target Variables Library.lvlib\\Needle Used"() -> (w830:i8)  [unwired: 1 in, 1 out]
      n345 = case "Needle Chosen: #1 or #2" shown="1, Default" w830 {
        tunnel: [w870 w876] -> w837
        tunnel: [w869 w875] -> w836
        tunnel: [w868 w871] -> w835
        tunnel: [w867 w874] -> w834
        tunnel: [w866 w872] -> w825
        tunnel: [w865 w873] -> w824
        frame 1, Default {
          w865 = T2 [{"PID gains"={"proportional gain (Kc)"=0.053, "integral time (Ti, min)"=3.5e-06, "derivative time (Td, min)"=0.0}, "max value"=0.0}, {"PID gains"={"proportional gain (Kc)"=0.053, "integral time (Ti, min)"=3.5e-06, "derivative time (Td, min)"=0.0}, "max value"=75.0}, {"PID gains"={"proportional gain (Kc)"=0.053, "integral time (Ti, min)"=3.5e-06, "derivative time (Td, min)"=0.0}, "max value"=100.0}, {"PID gains"={"proportional gain (Kc)"=0.055, "integral time (Ti, min)"=3.5e-06, "derivative time (Td, min)"=0.0}, "max value"=125.0}, {"PID gains"={"proportional gain (Kc)"=0.055, "integral time (Ti, min)"=3.5e-06, "derivative time (Td, min)"=0.0}, "max value"=150.0}, {"PID gains"={"proportional gain (Kc)"=0.055, "integral time (Ti, min)"=3.5e-06, "derivative time (Td, min)"=0.0}, "max value"=160.0}, {"PID gains"={"proportional gain (Kc)"=0.056, "integral time (Ti, min)"=3.5e-06, "derivative time (Td, min)"=0.0}, "max value"=165.0}, {"PID gains"={"proportional gain (Kc)"=0.056, "integral time (Ti, min)"=3.5e-06, "derivative time (Td, min)"=0.0}, "max value"=170.0}, {"PID gains"={"proportional gain (Kc)"=0.058, "integral time (Ti, min)"=3.5e-06, "derivative time (Td, min)"=0.0}, "max value"=175.0}, {"PID gains"={"proportional gain (Kc)"=0.058, "integral time (Ti, min)"=3.5e-06, "derivative time (Td, min)"=0.0}, "max value"=180.0}, {"PID gains"={"proportional gain (Kc)"=0.058, "integral time (Ti, min)"=3.5e-06, "derivative time (Td, min)"=0.0}, "max value"=185.0}, {"PID gains"={"proportional gain (Kc)"=0.058, "integral time (Ti, min)"=3.5e-06, "derivative time (Td, min)"=0.0}, "max value"=190.0}, {"PID gains"={"proportional gain (Kc)"=0.058, "integral time (Ti, min)"=3.5e-06, "derivative time (Td, min)"=0.0}, "max value"=210.0}]  # OFF PID gain schedule HyMu80#1 Needle OPTIMIZED
          w866 = T2 [{"PID gains"={"proportional gain (Kc)"=0.053, "integral time (Ti, min)"=3.5e-06, "derivative time (Td, min)"=0.0}, "max value"=0.0}, {"PID gains"={"proportional gain (Kc)"=0.053, "integral time (Ti, min)"=3.5e-06, "derivative time (Td, min)"=0.0}, "max value"=75.0}, {"PID gains"={"proportional gain (Kc)"=0.053, "integral time (Ti, min)"=3.5e-06, "derivative time (Td, min)"=0.0}, "max value"=100.0}, {"PID gains"={"proportional gain (Kc)"=0.055, "integral time (Ti, min)"=3.5e-06, "derivative time (Td, min)"=0.0}, "max value"=125.0}, {"PID gains"={"proportional gain (Kc)"=0.057, "integral time (Ti, min)"=3.5e-06, "derivative time (Td, min)"=0.0}, "max value"=150.0}, {"PID gains"={"proportional gain (Kc)"=0.058, "integral time (Ti, min)"=3.5e-06, "derivative time (Td, min)"=0.0}, "max value"=160.0}, {"PID gains"={"proportional gain (Kc)"=0.065, "integral time (Ti, min)"=3.5e-06, "derivative time (Td, min)"=0.0}, "max value"=165.0}, {"PID gains"={"proportional gain (Kc)"=0.111, "integral time (Ti, min)"=3.5e-06, "derivative time (Td, min)"=0.0}, "max value"=170.0}, {"PID gains"={"proportional gain (Kc)"=0.27, "integral time (Ti, min)"=3.5e-06, "derivative time (Td, min)"=0.0}, "max value"=175.0}, {"PID gains"={"proportional gain (Kc)"=0.32, "integral time (Ti, min)"=3.5e-06, "derivative time (Td, min)"=0.0}, "max value"=180.0}, {"PID gains"={"proportional gain (Kc)"=0.72, "integral time (Ti, min)"=3.5e-06, "derivative time (Td, min)"=0.0}, "max value"=185.0}, {"PID gains"={"proportional gain (Kc)"=0.8, "integral time (Ti, min)"=3.5e-06, "derivative time (Td, min)"=0.0}, "max value"=190.0}, {"PID gains"={"proportional gain (Kc)"=0.8, "integral time (Ti, min)"=3.5e-06, "derivative time (Td, min)"=0.0}, "max value"=210.0}]  # ON PID gain schedule HyMu80#1 Needle OPTIMIZED
          w867 = T2 [{"PID gains"={"proportional gain (Kc)"=0.08, "integral time (Ti, min)"=3.5e-06, "derivative time (Td, min)"=0.0}, "max value"=0.0}, {"PID gains"={"proportional gain (Kc)"=0.08, "integral time (Ti, min)"=3.5e-06, "derivative time (Td, min)"=0.0}, "max value"=145.0}, {"PID gains"={"proportional gain (Kc)"=0.075, "integral time (Ti, min)"=3.5e-06, "derivative time (Td, min)"=0.0}, "max value"=148.0}, {"PID gains"={"proportional gain (Kc)"=0.075, "integral time (Ti, min)"=3.5e-06, "derivative time (Td, min)"=0.0}, "max value"=150.0}, {"PID gains"={"proportional gain (Kc)"=0.075, "integral time (Ti, min)"=3.5e-06, "derivative time (Td, min)"=0.0}, "max value"=155.0}, {"PID gains"={"proportional gain (Kc)"=0.075, "integral time (Ti, min)"=3.5e-06, "derivative time (Td, min)"=0.0}, "max value"=160.0}, {"PID gains"={"proportional gain (Kc)"=0.078, "integral time (Ti, min)"=3.5e-06, "derivative time (Td, min)"=0.0}, "max value"=165.0}, {"PID gains"={"proportional gain (Kc)"=0.078, "integral time (Ti, min)"=3.5e-06, "derivative time (Td, min)"=0.0}, "max value"=170.0}, {"PID gains"={"proportional gain (Kc)"=0.081, "integral time (Ti, min)"=3.5e-06, "derivative time (Td, min)"=0.0}, "max value"=175.0}, {"PID gains"={"proportional gain (Kc)"=0.08, "integral time (Ti, min)"=3.5e-06, "derivative time (Td, min)"=0.0}, "max value"=180.0}, {"PID gains"={"proportional gain (Kc)"=0.085, "integral time (Ti, min)"=3.5e-06, "derivative time (Td, min)"=0.0}, "max value"=185.0}, {"PID gains"={"proportional gain (Kc)"=0.086, "integral time (Ti, min)"=3.5e-06, "derivative time (Td, min)"=0.0}, "max value"=190.0}, {"PID gains"={"proportional gain (Kc)"=0.086, "integral time (Ti, min)"=3.5e-06, "derivative time (Td, min)"=0.0}, "max value"=195.0}, {"PID gains"={"proportional gain (Kc)"=0.086, "integral time (Ti, min)"=3.5e-06, "derivative time (Td, min)"=0.0}, "max value"=220.0}]  # OFF PID gain schedule HyMu80#1 Needle MAX
          w868 = T2 [{"PID gains"={"proportional gain (Kc)"=0.08, "integral time (Ti, min)"=3.5e-06, "derivative time (Td, min)"=0.0}, "max value"=0.0}, {"PID gains"={"proportional gain (Kc)"=0.08, "integral time (Ti, min)"=3.5e-06, "derivative time (Td, min)"=0.0}, "max value"=145.0}, {"PID gains"={"proportional gain (Kc)"=0.075, "integral time (Ti, min)"=3.5e-06, "derivative time (Td, min)"=0.0}, "max value"=148.0}, {"PID gains"={"proportional gain (Kc)"=0.075, "integral time (Ti, min)"=3.5e-06, "derivative time (Td, min)"=0.0}, "max value"=150.0}, {"PID gains"={"proportional gain (Kc)"=0.075, "integral time (Ti, min)"=3.5e-06, "derivative time (Td, min)"=0.0}, "max value"=155.0}, {"PID gains"={"proportional gain (Kc)"=0.075, "integral time (Ti, min)"=3.5e-06, "derivative time (Td, min)"=0.0}, "max value"=160.0}, {"PID gains"={"proportional gain (Kc)"=0.078, "integral time (Ti, min)"=3.5e-06, "derivative time (Td, min)"=0.0}, "max value"=165.0}, {"PID gains"={"proportional gain (Kc)"=0.078, "integral time (Ti, min)"=3.5e-06, "derivative time (Td, min)"=0.0}, "max value"=170.0}, {"PID gains"={"proportional gain (Kc)"=0.081, "integral time (Ti, min)"=3.5e-06, "derivative time (Td, min)"=0.0}, "max value"=175.0}, {"PID gains"={"proportional gain (Kc)"=0.08, "integral time (Ti, min)"=3.5e-06, "derivative time (Td, min)"=0.0}, "max value"=180.0}, {"PID gains"={"proportional gain (Kc)"=0.085, "integral time (Ti, min)"=3.5e-06, "derivative time (Td, min)"=0.0}, "max value"=185.0}, {"PID gains"={"proportional gain (Kc)"=0.086, "integral time (Ti, min)"=3.5e-06, "derivative time (Td, min)"=0.0}, "max value"=190.0}, {"PID gains"={"proportional gain (Kc)"=0.086, "integral time (Ti, min)"=3.5e-06, "derivative time (Td, min)"=0.0}, "max value"=195.0}, {"PID gains"={"proportional gain (Kc)"=0.086, "integral time (Ti, min)"=3.5e-06, "derivative time (Td, min)"=0.0}, "max value"=220.0}]  # OFF PID gain schedule HyMu80#1 Needle MIN
          w869 = T2 [{"PID gains"={"proportional gain (Kc)"=0.08, "integral time (Ti, min)"=3.5e-06, "derivative time (Td, min)"=0.0}, "max value"=0.0}, {"PID gains"={"proportional gain (Kc)"=0.08, "integral time (Ti, min)"=3.5e-06, "derivative time (Td, min)"=0.0}, "max value"=145.0}, {"PID gains"={"proportional gain (Kc)"=0.083, "integral time (Ti, min)"=3.5e-06, "derivative time (Td, min)"=0.0}, "max value"=148.0}, {"PID gains"={"proportional gain (Kc)"=0.085, "integral time (Ti, min)"=3.5e-06, "derivative time (Td, min)"=0.0}, "max value"=150.0}, {"PID gains"={"proportional gain (Kc)"=0.0875, "integral time (Ti, min)"=3.5e-06, "derivative time (Td, min)"=0.0}, "max value"=155.0}, {"PID gains"={"proportional gain (Kc)"=0.123, "integral time (Ti, min)"=3.5e-06, "derivative time (Td, min)"=0.0}, "max value"=160.0}, {"PID gains"={"proportional gain (Kc)"=0.207, "integral time (Ti, min)"=3.5e-06, "derivative time (Td, min)"=0.0}, "max value"=165.0}, {"PID gains"={"proportional gain (Kc)"=0.315, "integral time (Ti, min)"=3.5e-06, "derivative time (Td, min)"=0.0}, "max value"=170.0}, {"PID gains"={"proportional gain (Kc)"=0.46, "integral time (Ti, min)"=3.5e-06, "derivative time (Td, min)"=0.0}, "max value"=175.0}, {"PID gains"={"proportional gain (Kc)"=0.65, "integral time (Ti, min)"=3.5e-06, "derivative time (Td, min)"=0.0}, "max value"=180.0}, {"PID gains"={"proportional gain (Kc)"=0.925, "integral time (Ti, min)"=3.5e-06, "derivative time (Td, min)"=0.0}, "max value"=185.0}, {"PID gains"={"proportional gain (Kc)"=1.04, "integral time (Ti, min)"=3.5e-06, "derivative time (Td, min)"=0.0}, "max value"=190.0}, {"PID gains"={"proportional gain (Kc)"=1.04, "integral time (Ti, min)"=3.5e-06, "derivative time (Td, min)"=0.0}, "max value"=195.0}, {"PID gains"={"proportional gain (Kc)"=1.04, "integral time (Ti, min)"=3.5e-06, "derivative time (Td, min)"=0.0}, "max value"=220.0}]  # ON PID gain schedule HyMu80#1 Needle MAX
          w870 = T2 [{"PID gains"={"proportional gain (Kc)"=0.075, "integral time (Ti, min)"=3.5e-06, "derivative time (Td, min)"=0.0}, "max value"=0.0}, {"PID gains"={"proportional gain (Kc)"=0.075, "integral time (Ti, min)"=3.5e-06, "derivative time (Td, min)"=0.0}, "max value"=145.0}, {"PID gains"={"proportional gain (Kc)"=0.075, "integral time (Ti, min)"=3.5e-06, "derivative time (Td, min)"=0.0}, "max value"=148.0}, {"PID gains"={"proportional gain (Kc)"=0.075, "integral time (Ti, min)"=3.5e-06, "derivative time (Td, min)"=0.0}, "max value"=150.0}, {"PID gains"={"proportional gain (Kc)"=0.0775, "integral time (Ti, min)"=3.5e-06, "derivative time (Td, min)"=0.0}, "max value"=155.0}, {"PID gains"={"proportional gain (Kc)"=0.117, "integral time (Ti, min)"=3.5e-06, "derivative time (Td, min)"=0.0}, "max value"=160.0}, {"PID gains"={"proportional gain (Kc)"=0.187, "integral time (Ti, min)"=3.5e-06, "derivative time (Td, min)"=0.0}, "max value"=165.0}, {"PID gains"={"proportional gain (Kc)"=0.28, "integral time (Ti, min)"=3.5e-06, "derivative time (Td, min)"=0.0}, "max value"=170.0}, {"PID gains"={"proportional gain (Kc)"=0.425, "integral time (Ti, min)"=3.5e-06, "derivative time (Td, min)"=0.0}, "max value"=175.0}, {"PID gains"={"proportional gain (Kc)"=0.615, "integral time (Ti, min)"=3.5e-06, "derivative time (Td, min)"=0.0}, "max value"=180.0}, {"PID gains"={"proportional gain (Kc)"=0.85, "integral time (Ti, min)"=3.5e-06, "derivative time (Td, min)"=0.0}, "max value"=185.0}, {"PID gains"={"proportional gain (Kc)"=1.0, "integral time (Ti, min)"=3.5e-06, "derivative time (Td, min)"=0.0}, "max value"=190.0}, {"PID gains"={"proportional gain (Kc)"=1.0, "integral time (Ti, min)"=3.5e-06, "derivative time (Td, min)"=0.0}, "max value"=195.0}, {"PID gains"={"proportional gain (Kc)"=1.0, "integral time (Ti, min)"=3.5e-06, "derivative time (Td, min)"=0.0}, "max value"=220.0}]  # ON PID gain schedule HyMu80#1 Needle MIN
          # "Updated on 2019-08-27"
          # "11/5/2018. Modified the PID gains for values 170 Gs and higher to make it more aggressive near the end."
          # "### values ABOVE ARE NOT UPDATED!!!! 3/25/2018"
          # "No discontinuity flux values will be selected\nNote: values that can leakage/ghosting/discontinuity in flux signals are not used.\nThis problem can be minimized by a number of techniques. However, I am not going to invest time \nin this right now. I can still generate fluxes of almost 200 Gs if Null Flux is -25 or -40 Gs. #WIM 1/16/2018"
          # "HyMu80#1 Needle Schedules Tuned on  1/11 & 12/2018 by #WIM\nfor fluxes:  ON/OFF\n145, 148, 150, 155, 160, 165, 170, 175, 180, 185, 190, 195 Gs\n220 Gs is for anything extra"
          # "HyMu80#1 Needle PID Parameters"
        }
        frame 2 {
          w873 = T2 [{"PID gains"={"proportional gain (Kc)"=0.053, "integral time (Ti, min)"=3.5e-06, "derivative time (Td, min)"=0.0}, "max value"=0.0}, {"PID gains"={"proportional gain (Kc)"=0.053, "integral time (Ti, min)"=3.5e-06, "derivative time (Td, min)"=0.0}, "max value"=75.0}, {"PID gains"={"proportional gain (Kc)"=0.053, "integral time (Ti, min)"=3.5e-06, "derivative time (Td, min)"=0.0}, "max value"=100.0}, {"PID gains"={"proportional gain (Kc)"=0.055, "integral time (Ti, min)"=3.5e-06, "derivative time (Td, min)"=0.0}, "max value"=125.0}, {"PID gains"={"proportional gain (Kc)"=0.055, "integral time (Ti, min)"=3.5e-06, "derivative time (Td, min)"=0.0}, "max value"=150.0}, {"PID gains"={"proportional gain (Kc)"=0.055, "integral time (Ti, min)"=3.5e-06, "derivative time (Td, min)"=0.0}, "max value"=160.0}, {"PID gains"={"proportional gain (Kc)"=0.055, "integral time (Ti, min)"=3.5e-06, "derivative time (Td, min)"=0.0}, "max value"=165.0}, {"PID gains"={"proportional gain (Kc)"=0.056, "integral time (Ti, min)"=3.5e-06, "derivative time (Td, min)"=0.0}, "max value"=170.0}, {"PID gains"={"proportional gain (Kc)"=0.057, "integral time (Ti, min)"=3.5e-06, "derivative time (Td, min)"=0.0}, "max value"=175.0}, {"PID gains"={"proportional gain (Kc)"=0.057, "integral time (Ti, min)"=3.5e-06, "derivative time (Td, min)"=0.0}, "max value"=180.0}, {"PID gains"={"proportional gain (Kc)"=0.057, "integral time (Ti, min)"=3.5e-06, "derivative time (Td, min)"=0.0}, "max value"=185.0}, {"PID gains"={"proportional gain (Kc)"=0.057, "integral time (Ti, min)"=3.5e-06, "derivative time (Td, min)"=0.0}, "max value"=190.0}, {"PID gains"={"proportional gain (Kc)"=0.057, "integral time (Ti, min)"=3.5e-06, "derivative time (Td, min)"=0.0}, "max value"=210.0}]  # OFF PID gain schedule HyMu80#1 Needle OPTIMIZED
          w872 = T2 [{"PID gains"={"proportional gain (Kc)"=0.053, "integral time (Ti, min)"=3.5e-06, "derivative time (Td, min)"=0.0}, "max value"=0.0}, {"PID gains"={"proportional gain (Kc)"=0.053, "integral time (Ti, min)"=3.5e-06, "derivative time (Td, min)"=0.0}, "max value"=75.0}, {"PID gains"={"proportional gain (Kc)"=0.053, "integral time (Ti, min)"=3.5e-06, "derivative time (Td, min)"=0.0}, "max value"=100.0}, {"PID gains"={"proportional gain (Kc)"=0.055, "integral time (Ti, min)"=3.5e-06, "derivative time (Td, min)"=0.0}, "max value"=125.0}, {"PID gains"={"proportional gain (Kc)"=0.057, "integral time (Ti, min)"=3.5e-06, "derivative time (Td, min)"=0.0}, "max value"=150.0}, {"PID gains"={"proportional gain (Kc)"=0.058, "integral time (Ti, min)"=3.5e-06, "derivative time (Td, min)"=0.0}, "max value"=160.0}, {"PID gains"={"proportional gain (Kc)"=0.065, "integral time (Ti, min)"=3.5e-06, "derivative time (Td, min)"=0.0}, "max value"=165.0}, {"PID gains"={"proportional gain (Kc)"=0.111, "integral time (Ti, min)"=3.5e-06, "derivative time (Td, min)"=0.0}, "max value"=170.0}, {"PID gains"={"proportional gain (Kc)"=0.185, "integral time (Ti, min)"=3.5e-06, "derivative time (Td, min)"=0.0}, "max value"=175.0}, {"PID gains"={"proportional gain (Kc)"=0.31, "integral time (Ti, min)"=3.5e-06, "derivative time (Td, min)"=0.0}, "max value"=180.0}, {"PID gains"={"proportional gain (Kc)"=0.55, "integral time (Ti, min)"=3.5e-06, "derivative time (Td, min)"=0.0}, "max value"=185.0}, {"PID gains"={"proportional gain (Kc)"=0.8, "integral time (Ti, min)"=3.5e-06, "derivative time (Td, min)"=0.0}, "max value"=190.0}, {"PID gains"={"proportional gain (Kc)"=0.8, "integral time (Ti, min)"=3.5e-06, "derivative time (Td, min)"=0.0}, "max value"=210.0}]  # ON PID gain schedule HyMu80#1 Needle OPTIMIZED
          w874 = T2 [{"PID gains"={"proportional gain (Kc)"=0.085, "integral time (Ti, min)"=3.5e-06, "derivative time (Td, min)"=0.0}, "max value"=0.0}, {"PID gains"={"proportional gain (Kc)"=0.085, "integral time (Ti, min)"=3.5e-06, "derivative time (Td, min)"=0.0}, "max value"=145.0}, {"PID gains"={"proportional gain (Kc)"=0.088, "integral time (Ti, min)"=3.5e-06, "derivative time (Td, min)"=0.0}, "max value"=148.0}, {"PID gains"={"proportional gain (Kc)"=0.091, "integral time (Ti, min)"=3.5e-06, "derivative time (Td, min)"=0.0}, "max value"=150.0}, {"PID gains"={"proportional gain (Kc)"=0.091, "integral time (Ti, min)"=3.5e-06, "derivative time (Td, min)"=0.0}, "max value"=155.0}, {"PID gains"={"proportional gain (Kc)"=0.092, "integral time (Ti, min)"=3.5e-06, "derivative time (Td, min)"=0.0}, "max value"=160.0}, {"PID gains"={"proportional gain (Kc)"=0.0935, "integral time (Ti, min)"=3.5e-06, "derivative time (Td, min)"=0.0}, "max value"=165.0}, {"PID gains"={"proportional gain (Kc)"=0.094, "integral time (Ti, min)"=3.5e-06, "derivative time (Td, min)"=0.0}, "max value"=170.0}, {"PID gains"={"proportional gain (Kc)"=0.0935, "integral time (Ti, min)"=3.5e-06, "derivative time (Td, min)"=0.0}, "max value"=175.0}, {"PID gains"={"proportional gain (Kc)"=0.097, "integral time (Ti, min)"=3.5e-06, "derivative time (Td, min)"=0.0}, "max value"=180.0}, {"PID gains"={"proportional gain (Kc)"=0.0945, "integral time (Ti, min)"=3.5e-06, "derivative time (Td, min)"=0.0}, "max value"=185.0}, {"PID gains"={"proportional gain (Kc)"=0.0945, "integral time (Ti, min)"=3.5e-06, "derivative time (Td, min)"=0.0}, "max value"=210.0}]  # OFF PID gain schedule HyMu80#2 Needle MAX
          w871 = T2 [{"PID gains"={"proportional gain (Kc)"=0.08, "integral time (Ti, min)"=3.5e-06, "derivative time (Td, min)"=0.0}, "max value"=0.0}, {"PID gains"={"proportional gain (Kc)"=0.08, "integral time (Ti, min)"=3.5e-06, "derivative time (Td, min)"=0.0}, "max value"=145.0}, {"PID gains"={"proportional gain (Kc)"=0.08, "integral time (Ti, min)"=3.5e-06, "derivative time (Td, min)"=0.0}, "max value"=148.0}, {"PID gains"={"proportional gain (Kc)"=0.082, "integral time (Ti, min)"=3.5e-06, "derivative time (Td, min)"=0.0}, "max value"=150.0}, {"PID gains"={"proportional gain (Kc)"=0.082, "integral time (Ti, min)"=3.5e-06, "derivative time (Td, min)"=0.0}, "max value"=155.0}, {"PID gains"={"proportional gain (Kc)"=0.082, "integral time (Ti, min)"=3.5e-06, "derivative time (Td, min)"=0.0}, "max value"=160.0}, {"PID gains"={"proportional gain (Kc)"=0.082, "integral time (Ti, min)"=3.5e-06, "derivative time (Td, min)"=0.0}, "max value"=165.0}, {"PID gains"={"proportional gain (Kc)"=0.083, "integral time (Ti, min)"=3.5e-06, "derivative time (Td, min)"=0.0}, "max value"=170.0}, {"PID gains"={"proportional gain (Kc)"=0.087, "integral time (Ti, min)"=3.5e-06, "derivative time (Td, min)"=0.0}, "max value"=175.0}, {"PID gains"={"proportional gain (Kc)"=0.092, "integral time (Ti, min)"=3.5e-06, "derivative time (Td, min)"=0.0}, "max value"=180.0}, {"PID gains"={"proportional gain (Kc)"=0.091, "integral time (Ti, min)"=3.5e-06, "derivative time (Td, min)"=0.0}, "max value"=185.0}, {"PID gains"={"proportional gain (Kc)"=0.091, "integral time (Ti, min)"=3.5e-06, "derivative time (Td, min)"=0.0}, "max value"=210.0}]  # OFF PID gain schedule HyMu80#2 Needle MIN
          w875 = T2 [{"PID gains"={"proportional gain (Kc)"=0.085, "integral time (Ti, min)"=3.5e-06, "derivative time (Td, min)"=0.0}, "max value"=0.0}, {"PID gains"={"proportional gain (Kc)"=0.085, "integral time (Ti, min)"=3.5e-06, "derivative time (Td, min)"=0.0}, "max value"=145.0}, {"PID gains"={"proportional gain (Kc)"=0.088, "integral time (Ti, min)"=3.5e-06, "derivative time (Td, min)"=0.0}, "max value"=148.0}, {"PID gains"={"proportional gain (Kc)"=0.113, "integral time (Ti, min)"=3.5e-06, "derivative time (Td, min)"=0.0}, "max value"=150.0}, {"PID gains"={"proportional gain (Kc)"=0.195, "integral time (Ti, min)"=3.5e-06, "derivative time (Td, min)"=0.0}, "max value"=155.0}, {"PID gains"={"proportional gain (Kc)"=0.31, "integral time (Ti, min)"=3.5e-06, "derivative time (Td, min)"=0.0}, "max value"=160.0}, {"PID gains"={"proportional gain (Kc)"=0.47, "integral time (Ti, min)"=3.5e-06, "derivative time (Td, min)"=0.0}, "max value"=165.0}, {"PID gains"={"proportional gain (Kc)"=0.725, "integral time (Ti, min)"=3.5e-06, "derivative time (Td, min)"=0.0}, "max value"=170.0}, {"PID gains"={"proportional gain (Kc)"=1.06, "integral time (Ti, min)"=3.5e-06, "derivative time (Td, min)"=0.0}, "max value"=175.0}, {"PID gains"={"proportional gain (Kc)"=1.3, "integral time (Ti, min)"=3.5e-06, "derivative time (Td, min)"=0.0}, "max value"=180.0}, {"PID gains"={"proportional gain (Kc)"=1.2, "integral time (Ti, min)"=3.5e-06, "derivative time (Td, min)"=0.0}, "max value"=185.0}, {"PID gains"={"proportional gain (Kc)"=1.2, "integral time (Ti, min)"=3.5e-06, "derivative time (Td, min)"=0.0}, "max value"=210.0}]  # ON PID gain schedule HyMu80#2 Needle MAX
          w876 = T2 [{"PID gains"={"proportional gain (Kc)"=0.08, "integral time (Ti, min)"=3.5e-06, "derivative time (Td, min)"=0.0}, "max value"=0.0}, {"PID gains"={"proportional gain (Kc)"=0.08, "integral time (Ti, min)"=3.5e-06, "derivative time (Td, min)"=0.0}, "max value"=145.0}, {"PID gains"={"proportional gain (Kc)"=0.08, "integral time (Ti, min)"=3.5e-06, "derivative time (Td, min)"=0.0}, "max value"=148.0}, {"PID gains"={"proportional gain (Kc)"=0.107, "integral time (Ti, min)"=3.5e-06, "derivative time (Td, min)"=0.0}, "max value"=150.0}, {"PID gains"={"proportional gain (Kc)"=0.188, "integral time (Ti, min)"=3.5e-06, "derivative time (Td, min)"=0.0}, "max value"=155.0}, {"PID gains"={"proportional gain (Kc)"=0.27, "integral time (Ti, min)"=3.5e-06, "derivative time (Td, min)"=0.0}, "max value"=160.0}, {"PID gains"={"proportional gain (Kc)"=0.435, "integral time (Ti, min)"=3.5e-06, "derivative time (Td, min)"=0.0}, "max value"=165.0}, {"PID gains"={"proportional gain (Kc)"=0.675, "integral time (Ti, min)"=3.5e-06, "derivative time (Td, min)"=0.0}, "max value"=170.0}, {"PID gains"={"proportional gain (Kc)"=0.945, "integral time (Ti, min)"=3.5e-06, "derivative time (Td, min)"=0.0}, "max value"=175.0}, {"PID gains"={"proportional gain (Kc)"=1.1, "integral time (Ti, min)"=3.5e-06, "derivative time (Td, min)"=0.0}, "max value"=180.0}, {"PID gains"={"proportional gain (Kc)"=1.15, "integral time (Ti, min)"=3.5e-06, "derivative time (Td, min)"=0.0}, "max value"=185.0}, {"PID gains"={"proportional gain (Kc)"=1.15, "integral time (Ti, min)"=3.5e-06, "derivative time (Td, min)"=0.0}, "max value"=210.0}]  # ON PID gain schedule HyMu80#2 Needle MIN
          # "Updated on 2019-08-14"
          # "### values HERE ARE NOT UPDATED!!!! 3/25/2018"
          # "No discontinuity flux values will be selected\nNote: values that can leakage/ghosting/discontinuity in flux signals are not used.\nThis problem can be minimized by a number of techniques. However, I am not going to invest time \nin this right now. I can still generate fluxes of almost 200 Gs if Null Flux is -25 or -40 Gs. #WIM 1/16/2018"
          # "HyMu80#2 Needle Schedules Tuned on  1/9 & 10/2018 by #WIM\nfor fluxes:  ON/OFF\n145, 148, 150, 155, 160, 165, 170, 175, 180, 185 Gs. \n220 Gs is for anything extra"
          # "HyMu80#2 Needle PID Parameters"
        }
      }
      n346 = shared-variable "NI-GenericDesktopPC-3A84958E\\Kopco PS Project Target Variables Library.lvlib\\Sampling Rate"() -> (w821:dbl)  [unwired: 1 in, 1 out]
      n347 = Greater?(x=w822, y="1st OFF Length (s)") -> (0:w812:bool)
      n348 = case shown="True" w812 {
        tunnel: "1st OFF Length (s)" -> [_ w864]
        tunnel: w822 -> [_ w863]
        tunnel: w821 -> [_ w861]
        tunnel: w820 -> [w847 w857]
        tunnel: [w847 w858] -> w819
        tunnel: [w846 w859] -> w817
        tunnel: w818 -> [w846 w860]
        tunnel: w816 -> [w845 w855]
        tunnel: [w845 w856] -> w815
        tunnel: w814 -> [w844 w853]
        tunnel: [w844 w854] -> w813
        tunnel: w810 -> [w843 w851]
        tunnel: [w843 w850] -> w809
        frame False {
        }
        frame True {
          w852 = 0 ("index")
          n349 = Subtract(x=w863, y=w864) -> (x-y=w862:dbl)
          n350 = Multiply(x=w861, y=w862) -> (x*y=w849:dbl)
          n351 = To Quad Integer(1:w849) -> (0:w848:i64)
          n352 = Subtract(x=w851, y=w848) -> (x-y=w850:i64)
          n353 = Delete From Array(array=w857, length=w848, index=w852) -> (array with subset deleted=w858:bool[])  [unwired: 1 out]
          n354 = Delete From Array(array=w855, length=w848, index=w852) -> (array with subset deleted=w856:dbl[])  [unwired: 1 out]
          n355 = Delete From Array(array=w853, length=w848, index=w852) -> (array with subset deleted=w854:dbl[])  [unwired: 1 out]
          n356 = Delete From Array(array=w860, length=w848, index=w852) -> (array with subset deleted=w859:bool[])  [unwired: 1 out]
        }
      }
      n357 = shared-variable "NI-GenericDesktopPC-3A84958E\\Kopco PS Project Target Variables Library.lvlib\\Zero Flux Observed GS"() -> (w840:dbl)  [unwired: 1 in, 1 out]
      n358 = shared-variable "NI-GenericDesktopPC-3A84958E\\Kopco PS Project Target Variables Library.lvlib\\Flux Setpoint ON Gs Relative"() -> (w838:dbl)  [unwired: 1 in, 1 out]
      n359 = Add(x=w838, y=w840) -> (x+y=w839:dbl)
      n360 = Absolute Value(x=w839) -> (abs(x)=w833:dbl)
      "ON Absolute\nFlux Setpoint (Gs)" <- w833
      n361 = shared-variable "NI-GenericDesktopPC-3A84958E\\Kopco PS Project Target Variables Library.lvlib\\Samples Total"(w809) -> ()  [unwired: 1 in, 1 out]
      n362 = case "OFF Flux PID Gain Parameters: Interpolated vs. Fixed" shown="0, Default" w832 {
        tunnel: w833 -> [w880 w1025]
        tunnel: [w882 w1027] -> w826
        tunnel: w835 -> [w881 w1024]
        tunnel: w834 -> [w879 w1026]
        tunnel: w831 -> [w878 w1023]
        tunnel: w824 -> [w877 w1022]
        frame 0, Default {
          # "Interpolated Schedule"
          n363 = case "PID Paramter Aggressiveness" shown="1" w878 {
            tunnel: [w885 w917 w951 w992] -> w882
            tunnel: w881 -> [_ w915 w948 _]
            tunnel: w880 -> [w884 w916 w947 w991]
            tunnel: w879 -> [_ _ w949 w990]
            tunnel: w877 -> [w883 _ _ _]
            frame 0, Default {
              w895 = dbl[] []
              # "Rebundling PID Parameters without Names\nbut it should work the same"
              # "Optimized Interpolated"
              n364 = Array Size(array=w883) -> (size(s)=w897:i32)
              n365 = for {
                N: w897 -> [_]
                tunnel: w884 -> [w913]
                shift-right: [w911] -> w894
                shift-left: dbl[] [] -> [w912]
                tunnel: [w913] -> w887
                shift-right: [w909] -> w891
                shift-left: w895 -> [w910]
                shift-right: [w907] -> w893
                shift-left: w895 -> [w906]
                shift-right: [w908] -> w886
                shift-left: w895 -> [w905]
                tunnel: w883 -> [w904]
                i -> [w914]
                n366 = Index Array(array=w904, index=w914) -> (element=w903:T7)
                n367 = Unbundle(w903) -> ("PID gains"=w901:T1, "max value"=w902:dbl)
                n368 = Unbundle(w901) -> ("proportional gain (Kc)"=w898:dbl, "integral time (Ti, min)"=w900:dbl, "derivative time (Td, min)"=w899:dbl)
                n369 = Build Array (concatenate)(w912, w902) -> (w911:dbl[])
                n370 = Build Array (concatenate)(w910, w898) -> (w909:dbl[])
                n371 = Build Array (concatenate)(w906, w900) -> (w907:dbl[])
                n372 = Build Array (concatenate)(w905, w899) -> (w908:dbl[])
              }
              n373 = Threshold 1D Array(2:w887, 3:w894) -> (0:w892:dbl)  [unwired: 1 in]
              n374 = Interpolate 1D Array(1:w892, 2:w891) -> (0:w890:dbl)
              n375 = Interpolate 1D Array(1:w892, 2:w893) -> (0:w889:dbl)
              n376 = Interpolate 1D Array(1:w892, 2:w886) -> (0:w888:dbl)
              n377 = Bundle(w890, w889, w888) -> (w885:cluster{dbl, dbl, dbl})  [unwired: 1 in]
            }
            frame 1 {
              w927 = dbl[] []
              # "Rebundling PID Parameters without Names\nbut it should work the same"
              # "Minimum Interpolated"
              n378 = Array Size(array=w915) -> (size(s)=w929:i32)
              n379 = for {
                N: w929 -> [_]
                tunnel: w916 -> [w945]
                shift-right: [w943] -> w926
                shift-left: dbl[] [] -> [w944]
                tunnel: [w945] -> w919
                shift-right: [w941] -> w923
                shift-left: w927 -> [w942]
                shift-right: [w939] -> w925
                shift-left: w927 -> [w938]
                shift-right: [w940] -> w918
                shift-left: w927 -> [w937]
                tunnel: w915 -> [w936]
                i -> [w946]
                n380 = Index Array(array=w936, index=w946) -> (element=w935:T7)
                n381 = Unbundle(w935) -> ("PID gains"=w933:T1, "max value"=w934:dbl)
                n382 = Unbundle(w933) -> ("proportional gain (Kc)"=w930:dbl, "integral time (Ti, min)"=w932:dbl, "derivative time (Td, min)"=w931:dbl)
                n383 = Build Array (concatenate)(w944, w934) -> (w943:dbl[])
                n384 = Build Array (concatenate)(w942, w930) -> (w941:dbl[])
                n385 = Build Array (concatenate)(w938, w932) -> (w939:dbl[])
                n386 = Build Array (concatenate)(w937, w931) -> (w940:dbl[])
              }
              n387 = Threshold 1D Array(2:w919, 3:w926) -> (0:w924:dbl)  [unwired: 1 in]
              n388 = Interpolate 1D Array(1:w924, 2:w923) -> (0:w922:dbl)
              n389 = Interpolate 1D Array(1:w924, 2:w925) -> (0:w921:dbl)
              n390 = Interpolate 1D Array(1:w924, 2:w918) -> (0:w920:dbl)
              n391 = Bundle(w922, w921, w920) -> (w917:cluster{dbl, dbl, dbl})  [unwired: 1 in]
            }
            frame 2 {
              w959 = dbl[] []
              # "Average Interpolated"
              n392 = Array Size(array=w948) -> (size(s)=w961:i32)
              n393 = for {
                N: w961 -> [_]
                tunnel: w948 -> [w989]
                shift-right: [w985] -> w957
                shift-left: dbl[] [] -> [w986]
                shift-right: [w983] -> w954
                shift-left: w959 -> [w984]
                shift-right: [w981] -> w955
                shift-left: w959 -> [w980]
                shift-right: [w982] -> w956
                shift-left: w959 -> [w979]
                tunnel: w949 -> [w976]
                i -> [w975]
                n394 = Index Array(array=w989, index=w975) -> (element=w988:T7)
                n395 = Index Array(array=w976, index=w975) -> (element=w978:T7)
                n396 = Unbundle(w988) -> ("PID gains"=w987:T1)  [unwired: 1 out]
                n397 = Unbundle(w978) -> ("PID gains"=w974:T1, "max value"=w977:dbl)
                n398 = Unbundle(w987) -> ("proportional gain (Kc)"=w972:dbl, "integral time (Ti, min)"=w968:dbl, "derivative time (Td, min)"=w966:dbl)
                n399 = Build Array (concatenate) "Flux Cutoff"(w986, w977) -> (w985:dbl[])
                n400 = Unbundle(w974) -> ("proportional gain (Kc)"=w973:dbl, "integral time (Ti, min)"=w967:dbl, "derivative time (Td, min)"=w963:dbl)
                n401 = Build Array(w972, w973) -> (w971:dbl[])
                n402 = Build Array(w968, w967) -> (w970:dbl[])
                n403 = call-poly <vilib>:"Mean.vi"("X"=w971) -> ("mean"=w962:dbl)  [unwired: 1 out]
                n404 = Build Array(w966, w963) -> (w969:dbl[])
                n405 = call-poly <vilib>:"Mean.vi"("X"=w970) -> ("mean"=w965:dbl)  [unwired: 1 out]
                n406 = call-poly <vilib>:"Mean.vi"("X"=w969) -> ("mean"=w964:dbl)  [unwired: 1 out]
                n407 = Build Array (concatenate) "K_c"(w984, w962) -> (w983:dbl[])
                n408 = Build Array (concatenate) "T_i"(w980, w965) -> (w981:dbl[])
                n409 = Build Array (concatenate) "T_d"(w979, w964) -> (w982:dbl[])
              }
              n410 = Threshold 1D Array(2:w947, 3:w957) -> (0:w958:dbl)  [unwired: 1 in]
              n411 = Interpolate 1D Array(1:w958, 2:w954) -> (0:w953:dbl)
              n412 = Interpolate 1D Array(1:w958, 2:w955) -> (0:w952:dbl)
              n413 = Interpolate 1D Array(1:w958, 2:w956) -> (0:w950:dbl)
              n414 = Bundle(w953, w952, w950) -> (w951:cluster{dbl, dbl, dbl})  [unwired: 1 in]
            }
            frame 3 {
              w1002 = dbl[] []
              # "Maximum Interpolated"
              # "Rebundling PID Parameters without Names\nbut it should work the same"
              n415 = Array Size(array=w990) -> (size(s)=w1004:i32)
              n416 = for {
                N: w1004 -> [_]
                tunnel: w991 -> [w1020]
                shift-right: [w1018] -> w1001
                shift-left: dbl[] [] -> [w1019]
                tunnel: [w1020] -> w994
                shift-right: [w1016] -> w998
                shift-left: w1002 -> [w1017]
                shift-right: [w1014] -> w1000
                shift-left: w1002 -> [w1013]
                shift-right: [w1015] -> w993
                shift-left: w1002 -> [w1012]
                tunnel: w990 -> [w1011]
                i -> [w1021]
                n417 = Index Array(array=w1011, index=w1021) -> (element=w1010:T7)
                n418 = Unbundle(w1010) -> ("PID gains"=w1008:T1, "max value"=w1009:dbl)
                n419 = Unbundle(w1008) -> ("proportional gain (Kc)"=w1005:dbl, "integral time (Ti, min)"=w1007:dbl, "derivative time (Td, min)"=w1006:dbl)
                n420 = Build Array (concatenate)(w1019, w1009) -> (w1018:dbl[])
                n421 = Build Array (concatenate)(w1017, w1005) -> (w1016:dbl[])
                n422 = Build Array (concatenate)(w1013, w1007) -> (w1014:dbl[])
                n423 = Build Array (concatenate)(w1012, w1006) -> (w1015:dbl[])
              }
              n424 = Threshold 1D Array(2:w994, 3:w1001) -> (0:w999:dbl)  [unwired: 1 in]
              n425 = Interpolate 1D Array(1:w999, 2:w998) -> (0:w997:dbl)
              n426 = Interpolate 1D Array(1:w999, 2:w1000) -> (0:w996:dbl)
              n427 = Interpolate 1D Array(1:w999, 2:w993) -> (0:w995:dbl)
              n428 = Bundle(w997, w996, w995) -> (w992:cluster{dbl, dbl, dbl})  [unwired: 1 in]
            }
          }
        }
        frame 1 {
          # "Fixed Schedule"
          n429 = case "PID Paramter Aggressiveness" shown="2" w1023 {
            tunnel: [w1030 w1033 w1037 w1054] -> w1027
            tunnel: w1026 -> [_ _ w1035 w1053]
            tunnel: w1025 -> [w1029 w1032 w1034 w1052]
            tunnel: w1024 -> [_ w1031 w1036 _]
            tunnel: w1022 -> [w1028 _ _ _]
            frame 0, Default {
              # "Optimized Fixed"
              n430 = call-poly <vilib>:"PID Gain Schedule.vi"("PID gain schedule"=w1028, "gain scheduling value"=w1029) -> ("PID gains out"=w1030:T1)  [unwired: 2 in, 1 out]
            }
            frame 1 {
              # "Minimum Fixed"
              n431 = call-poly <vilib>:"PID Gain Schedule.vi"("PID gain schedule"=w1031, "gain scheduling value"=w1032) -> ("PID gains out"=w1033:T1)  [unwired: 2 in, 1 out]
            }
            frame 2 {
              # "Averaged Fixed"
              n432 = call-poly <vilib>:"PID Gain Schedule.vi"("PID gain schedule"=w1036, "gain scheduling value"=w1034) -> ("PID gains out"=w1042:T1)  [unwired: 2 in, 1 out]
              n433 = call-poly <vilib>:"PID Gain Schedule.vi"("PID gain schedule"=w1035, "gain scheduling value"=w1034) -> ("PID gains out"=w1041:T1)  [unwired: 2 in, 1 out]
              n434 = Unbundle(w1042) -> ("proportional gain (Kc)"=w1050:dbl, "integral time (Ti, min)"=w1046:dbl, "derivative time (Td, min)"=w1044:dbl)
              n435 = Unbundle(w1041) -> ("proportional gain (Kc)"=w1051:dbl, "integral time (Ti, min)"=w1045:dbl, "derivative time (Td, min)"=w1043:dbl)
              n436 = Build Array(w1050, w1051) -> (w1049:dbl[])
              n437 = Build Array(w1046, w1045) -> (w1048:dbl[])
              n438 = call-poly <vilib>:"Mean.vi"("X"=w1049) -> ("mean"=w1038:dbl)  [unwired: 1 out]
              n439 = Build Array(w1044, w1043) -> (w1047:dbl[])
              n440 = call-poly <vilib>:"Mean.vi"("X"=w1048) -> ("mean"=w1040:dbl)  [unwired: 1 out]
              n441 = call-poly <vilib>:"Mean.vi"("X"=w1047) -> ("mean"=w1039:dbl)  [unwired: 1 out]
              n442 = Bundle("mean"=w1038, "mean"=w1040, "mean"=w1039) -> (w1037:cluster{"mean":dbl, "mean":dbl, "mean":dbl})  [unwired: 1 in]
            }
            frame 3 {
              # "Maximum Fixed"
              n443 = call-poly <vilib>:"PID Gain Schedule.vi"("PID gain schedule"=w1053, "gain scheduling value"=w1052) -> ("PID gains out"=w1054:T1)  [unwired: 2 in, 1 out]
            }
          }
        }
      }
      "Suggested PID gains OFF" <- w826
      n444 = case "ON Flux PID Gain Parameters: Interpolated vs. Fixed" shown="1" w832 {
        tunnel: w833 -> [w1057 w1202]
        tunnel: [w1059 w1204] -> w827
        tunnel: w831 -> [w1060 w1205]
        tunnel: w837 -> [w1058 w1201]
        tunnel: w836 -> [w1056 w1203]
        tunnel: w825 -> [w1055 w1200]
        frame 0, Default {
          # "Interpolated Schedule"
          n445 = case "PID Paramter Aggressiveness" shown="0, Default" w1060 {
            tunnel: [w1063 w1095 w1129 w1170] -> w1059
            tunnel: w1058 -> [_ w1093 w1126 _]
            tunnel: w1057 -> [w1062 w1094 w1125 w1169]
            tunnel: w1056 -> [_ _ w1127 w1168]
            tunnel: w1055 -> [w1061 _ _ _]
            frame 0, Default {
              w1073 = dbl[] []
              # "Rebundling PID Parameters without Names\nbut it should work the same"
              # "Optimized Interpolated"
              n446 = Array Size(array=w1061) -> (size(s)=w1075:i32)
              n447 = for {
                N: w1075 -> [_]
                tunnel: w1062 -> [w1091]
                shift-right: [w1089] -> w1072
                shift-left: dbl[] [] -> [w1090]
                tunnel: [w1091] -> w1065
                shift-right: [w1087] -> w1069
                shift-left: w1073 -> [w1088]
                shift-right: [w1085] -> w1071
                shift-left: w1073 -> [w1084]
                shift-right: [w1086] -> w1064
                shift-left: w1073 -> [w1083]
                tunnel: w1061 -> [w1082]
                i -> [w1092]
                n448 = Index Array(array=w1082, index=w1092) -> (element=w1081:T7)
                n449 = Unbundle(w1081) -> ("PID gains"=w1079:T1, "max value"=w1080:dbl)
                n450 = Unbundle(w1079) -> ("proportional gain (Kc)"=w1076:dbl, "integral time (Ti, min)"=w1078:dbl, "derivative time (Td, min)"=w1077:dbl)
                n451 = Build Array (concatenate)(w1090, w1080) -> (w1089:dbl[])
                n452 = Build Array (concatenate)(w1088, w1076) -> (w1087:dbl[])
                n453 = Build Array (concatenate)(w1084, w1078) -> (w1085:dbl[])
                n454 = Build Array (concatenate)(w1083, w1077) -> (w1086:dbl[])
              }
              n455 = Threshold 1D Array(2:w1065, 3:w1072) -> (0:w1070:dbl)  [unwired: 1 in]
              n456 = Interpolate 1D Array(1:w1070, 2:w1069) -> (0:w1068:dbl)
              n457 = Interpolate 1D Array(1:w1070, 2:w1071) -> (0:w1067:dbl)
              n458 = Interpolate 1D Array(1:w1070, 2:w1064) -> (0:w1066:dbl)
              n459 = Bundle(w1068, w1067, w1066) -> (w1063:cluster{dbl, dbl, dbl})  [unwired: 1 in]
            }
            frame 1 {
              w1105 = dbl[] []
              # "Rebundling PID Parameters without Names\nbut it should work the same"
              # "Minimum Interpolated"
              n460 = Array Size(array=w1093) -> (size(s)=w1107:i32)
              n461 = for {
                N: w1107 -> [_]
                tunnel: w1094 -> [w1123]
                shift-right: [w1121] -> w1104
                shift-left: dbl[] [] -> [w1122]
                tunnel: [w1123] -> w1097
                shift-right: [w1119] -> w1101
                shift-left: w1105 -> [w1120]
                shift-right: [w1117] -> w1103
                shift-left: w1105 -> [w1116]
                shift-right: [w1118] -> w1096
                shift-left: w1105 -> [w1115]
                tunnel: w1093 -> [w1114]
                i -> [w1124]
                n462 = Index Array(array=w1114, index=w1124) -> (element=w1113:T7)
                n463 = Unbundle(w1113) -> ("PID gains"=w1111:T1, "max value"=w1112:dbl)
                n464 = Unbundle(w1111) -> ("proportional gain (Kc)"=w1108:dbl, "integral time (Ti, min)"=w1110:dbl, "derivative time (Td, min)"=w1109:dbl)
                n465 = Build Array (concatenate)(w1122, w1112) -> (w1121:dbl[])
                n466 = Build Array (concatenate)(w1120, w1108) -> (w1119:dbl[])
                n467 = Build Array (concatenate)(w1116, w1110) -> (w1117:dbl[])
                n468 = Build Array (concatenate)(w1115, w1109) -> (w1118:dbl[])
              }
              n469 = Threshold 1D Array(2:w1097, 3:w1104) -> (0:w1102:dbl)  [unwired: 1 in]
              n470 = Interpolate 1D Array(1:w1102, 2:w1101) -> (0:w1100:dbl)
              n471 = Interpolate 1D Array(1:w1102, 2:w1103) -> (0:w1099:dbl)
              n472 = Interpolate 1D Array(1:w1102, 2:w1096) -> (0:w1098:dbl)
              n473 = Bundle(w1100, w1099, w1098) -> (w1095:cluster{dbl, dbl, dbl})  [unwired: 1 in]
            }
            frame 2 {
              w1137 = dbl[] []
              # "Average Interpolated"
              n474 = Array Size(array=w1126) -> (size(s)=w1139:i32)
              n475 = for {
                N: w1139 -> [_]
                tunnel: w1126 -> [w1167]
                shift-right: [w1163] -> w1135
                shift-left: dbl[] [] -> [w1164]
                shift-right: [w1161] -> w1132
                shift-left: w1137 -> [w1162]
                shift-right: [w1159] -> w1133
                shift-left: w1137 -> [w1158]
                shift-right: [w1160] -> w1134
                shift-left: w1137 -> [w1157]
                tunnel: w1127 -> [w1154]
                i -> [w1153]
                n476 = Index Array(array=w1167, index=w1153) -> (element=w1166:T7)
                n477 = Index Array(array=w1154, index=w1153) -> (element=w1156:T7)
                n478 = Unbundle(w1166) -> ("PID gains"=w1165:T1)  [unwired: 1 out]
                n479 = Unbundle(w1156) -> ("PID gains"=w1152:T1, "max value"=w1155:dbl)
                n480 = Unbundle(w1165) -> ("proportional gain (Kc)"=w1150:dbl, "integral time (Ti, min)"=w1146:dbl, "derivative time (Td, min)"=w1144:dbl)
                n481 = Build Array (concatenate) "Flux Cutoff"(w1164, w1155) -> (w1163:dbl[])
                n482 = Unbundle(w1152) -> ("proportional gain (Kc)"=w1151:dbl, "integral time (Ti, min)"=w1145:dbl, "derivative time (Td, min)"=w1141:dbl)
                n483 = Build Array(w1150, w1151) -> (w1149:dbl[])
                n484 = Build Array(w1146, w1145) -> (w1148:dbl[])
                n485 = call-poly <vilib>:"Mean.vi"("X"=w1149) -> ("mean"=w1140:dbl)  [unwired: 1 out]
                n486 = Build Array(w1144, w1141) -> (w1147:dbl[])
                n487 = call-poly <vilib>:"Mean.vi"("X"=w1148) -> ("mean"=w1143:dbl)  [unwired: 1 out]
                n488 = call-poly <vilib>:"Mean.vi"("X"=w1147) -> ("mean"=w1142:dbl)  [unwired: 1 out]
                n489 = Build Array (concatenate) "K_c"(w1162, w1140) -> (w1161:dbl[])
                n490 = Build Array (concatenate) "T_i"(w1158, w1143) -> (w1159:dbl[])
                n491 = Build Array (concatenate) "T_d"(w1157, w1142) -> (w1160:dbl[])
              }
              n492 = Threshold 1D Array(2:w1125, 3:w1135) -> (0:w1136:dbl)  [unwired: 1 in]
              n493 = Interpolate 1D Array(1:w1136, 2:w1132) -> (0:w1131:dbl)
              n494 = Interpolate 1D Array(1:w1136, 2:w1133) -> (0:w1130:dbl)
              n495 = Interpolate 1D Array(1:w1136, 2:w1134) -> (0:w1128:dbl)
              n496 = Bundle(w1131, w1130, w1128) -> (w1129:cluster{dbl, dbl, dbl})  [unwired: 1 in]
            }
            frame 3 {
              w1180 = dbl[] []
              # "Maximum Interpolated"
              # "Rebundling PID Parameters without Names\nbut it should work the same"
              n497 = Array Size(array=w1168) -> (size(s)=w1182:i32)
              n498 = for {
                N: w1182 -> [_]
                tunnel: w1169 -> [w1198]
                shift-right: [w1196] -> w1179
                shift-left: dbl[] [] -> [w1197]
                tunnel: [w1198] -> w1172
                shift-right: [w1194] -> w1176
                shift-left: w1180 -> [w1195]
                shift-right: [w1192] -> w1178
                shift-left: w1180 -> [w1191]
                shift-right: [w1193] -> w1171
                shift-left: w1180 -> [w1190]
                tunnel: w1168 -> [w1189]
                i -> [w1199]
                n499 = Index Array(array=w1189, index=w1199) -> (element=w1188:T7)
                n500 = Unbundle(w1188) -> ("PID gains"=w1186:T1, "max value"=w1187:dbl)
                n501 = Unbundle(w1186) -> ("proportional gain (Kc)"=w1183:dbl, "integral time (Ti, min)"=w1185:dbl, "derivative time (Td, min)"=w1184:dbl)
                n502 = Build Array (concatenate)(w1197, w1187) -> (w1196:dbl[])
                n503 = Build Array (concatenate)(w1195, w1183) -> (w1194:dbl[])
                n504 = Build Array (concatenate)(w1191, w1185) -> (w1192:dbl[])
                n505 = Build Array (concatenate)(w1190, w1184) -> (w1193:dbl[])
              }
              n506 = Threshold 1D Array(2:w1172, 3:w1179) -> (0:w1177:dbl)  [unwired: 1 in]
              n507 = Interpolate 1D Array(1:w1177, 2:w1176) -> (0:w1175:dbl)
              n508 = Interpolate 1D Array(1:w1177, 2:w1178) -> (0:w1174:dbl)
              n509 = Interpolate 1D Array(1:w1177, 2:w1171) -> (0:w1173:dbl)
              n510 = Bundle(w1175, w1174, w1173) -> (w1170:cluster{dbl, dbl, dbl})  [unwired: 1 in]
            }
          }
        }
        frame 1 {
          # "Fixed Schedule"
          n511 = case "PID Paramter Aggressiveness" shown="2" w1205 {
            tunnel: [w1206 w1211 w1215 w1232] -> w1204
            tunnel: w1203 -> [_ _ w1212 w1231]
            tunnel: w1202 -> [w1207 w1210 w1213 w1230]
            tunnel: w1201 -> [_ w1209 w1214 _]
            tunnel: w1200 -> [w1208 _ _ _]
            frame 0 {
              # "Optimized Fixed"
              n512 = call-poly <vilib>:"PID Gain Schedule.vi"("PID gain schedule"=w1208, "gain scheduling value"=w1207) -> ("PID gains out"=w1206:T1)  [unwired: 2 in, 1 out]
            }
            frame 1, Default {
              # "Minimum Fixed"
              n513 = call-poly <vilib>:"PID Gain Schedule.vi"("PID gain schedule"=w1209, "gain scheduling value"=w1210) -> ("PID gains out"=w1211:T1)  [unwired: 2 in, 1 out]
            }
            frame 2 {
              # "Averaged Fixed"
              n514 = call-poly <vilib>:"PID Gain Schedule.vi"("PID gain schedule"=w1214, "gain scheduling value"=w1213) -> ("PID gains out"=w1220:T1)  [unwired: 2 in, 1 out]
              n515 = call-poly <vilib>:"PID Gain Schedule.vi"("PID gain schedule"=w1212, "gain scheduling value"=w1213) -> ("PID gains out"=w1219:T1)  [unwired: 2 in, 1 out]
              n516 = Unbundle(w1220) -> ("proportional gain (Kc)"=w1228:dbl, "integral time (Ti, min)"=w1224:dbl, "derivative time (Td, min)"=w1222:dbl)
              n517 = Unbundle(w1219) -> ("proportional gain (Kc)"=w1229:dbl, "integral time (Ti, min)"=w1223:dbl, "derivative time (Td, min)"=w1221:dbl)
              n518 = Build Array(w1228, w1229) -> (w1227:dbl[])
              n519 = Build Array(w1224, w1223) -> (w1226:dbl[])
              n520 = call-poly <vilib>:"Mean.vi"("X"=w1227) -> ("mean"=w1216:dbl)  [unwired: 1 out]
              n521 = Build Array(w1222, w1221) -> (w1225:dbl[])
              n522 = call-poly <vilib>:"Mean.vi"("X"=w1226) -> ("mean"=w1218:dbl)  [unwired: 1 out]
              n523 = call-poly <vilib>:"Mean.vi"("X"=w1225) -> ("mean"=w1217:dbl)  [unwired: 1 out]
              n524 = Bundle("mean"=w1216, "mean"=w1218, "mean"=w1217) -> (w1215:cluster{"mean":dbl, "mean":dbl, "mean":dbl})  [unwired: 1 in]
            }
            frame 3 {
              # "Maximum Fixed"
              n525 = call-poly <vilib>:"PID Gain Schedule.vi"("PID gain schedule"=w1231, "gain scheduling value"=w1230) -> ("PID gains out"=w1232:T1)  [unwired: 2 in, 1 out]
            }
          }
        }
      }
      "Suggested PID gains ON" <- w827
      n526 = shared-variable "NI-GenericDesktopPC-3A84958E\\Kopco PS Project Target Variables Library.lvlib\\Digital Trigger"() -> (w808:bool)  [unwired: 1 in, 1 out]
      n527 = shared-variable "NI-GenericDesktopPC-3A84958E\\Kopco PS Project Target Variables Library.lvlib\\Data Upload"() -> (w807:bool)  [unwired: 1 in, 1 out]
      n528 = case shown="True" w808 {
        frame False {
        }
        frame True {
          n529 = shared-variable "NI-GenericDesktopPC-3A84958E\\Kopco PS Project Target Variables Library.lvlib\\Digital Trigger"(FALSE ("Digital Trigger")) -> ()  [unwired: 1 in, 1 out]
        }
      }
      n530 = case shown="True" w807 {
        frame False {
        }
        frame True {
          n531 = shared-variable "NI-GenericDesktopPC-3A84958E\\Kopco PS Project Target Variables Library.lvlib\\Data Upload"(FALSE ("Digital Trigger")) -> ()  [unwired: 1 in, 1 out]
        }
      }
    }
    frame #17 {
      # "Bound to \"PID Parameters Selected\"\nshared global variable"
      # "Bound to \"Data Logger Running\"\nshared global variable."
      # "Flux ON/OFF Logical"
      # "AO values of current"
      # "Sampling Rate"
      # "Flux Control Sequence"
      # "Mini DeGauss AO Sequence, Normalized"
      # "Mini DeGauss Logical"
      # "Ask if you want to tweak the current parameters. This is useful in \ninterpolation cases, and when values change over time"
      # "Step 4 Specifying PID Parameters"
      n532 = flat-sequence {
        tunnel: w1246 -> [w1251]
        tunnel: w1247 -> [w1254]
        tunnel: [w1255] -> w1244
        tunnel: [w1253] -> w1236
        tunnel: [w1252] -> w1235
        tunnel: [w1265] -> w1245
        tunnel: [w1263] -> w1243
        tunnel: [w1262] -> w1242
        tunnel: w1244 -> [w1261]
        tunnel: w1236 -> [w1264]
        tunnel: w1235 -> [w1260]
        frame #0 {
          n533 = while {
            tunnel: ["Start Null Flux Adjustment 2"] -> _
            tunnel: ["Keep Null Flux Running \n       Until Next Step? 2"] -> w1255
            tunnel: w1254 -> [w1257]
            tunnel: [w1257] -> w1253
            tunnel: [w1256] -> w1252
            tunnel: w1251 -> [w1256]
            stop <- "Start Null Flux Adjustment 2" stop-if-true
          }
        }
        frame #1 {
          n534 = case shown="False" w1261 {
            tunnel: [TRUE TRUE] -> w1265
            tunnel: w1264 -> [w1266 _]
            tunnel: [w1266 "Tweaked PID gains ON"] -> w1263
            tunnel: [w1267 "Tweaked PID gains OFF"] -> w1262
            tunnel: w1260 -> [w1267 _]
            frame False {
              # "No Change in PID Parameters"
            }
            frame True {
            }
          }
        }
      }
      n535 = shared-variable "NI-GenericDesktopPC-3A84958E\\Kopco PS Project Target Variables Library.lvlib\\PID Parameters Selected"(w1245) -> ()  [unwired: 1 in, 1 out]
      "PID gains ON Chosen" <- w1243
      "PID gains OFF Chosen" <- w1242
    }
    frame #18 {
      w1297 = -1 items=["default"=-1, "RSE"=10083, "NRSE"=10078, "Differential"=10106, "Pseudodifferential"=12529] ("Terminal Configuration")
      w1302 = "Dev2/ao0"  # Power Supply Control
      w1301 = 12522 items=["Finite Samples"=10178, "Continuous Samples"=10123, "Hardware Timed Single Point"=12522]  # Sample Mode
      w1307 = 10106 items=["default"=-1, "RSE"=10083, "NRSE"=10078, "Differential"=10106, "Pseudodifferential"=12529] ("Terminal Configuration")
      w1310 = 12522 items=["Finite Samples"=10178, "Continuous Samples"=10123, "Hardware Timed Single Point"=12522]  # Sample Mode
      # "1/4 wave to get the main points of the\n mini DeGauss waveform 3/12/2018"
      # "Reversed order of AI7 & AI3 on 4/11/2018 to \nminimize leakage to Channel 7"
      # "# of samples of Mini DeGauss"
      # "Fixed by WIM on 3/5/2018 to keep the old AO value"
      # "Step 5 Preparing DAQ for Waveform"
      # "Total Number of Samples"
      n536 = shared-variable "NI-GenericDesktopPC-3A84958E\\Kopco PS Project Target Variables Library.lvlib\\Channels AI List"() -> (w1273:string)  [unwired: 1 in, 1 out]
      n537 = shared-variable "NI-GenericDesktopPC-3A84958E\\Kopco PS Project Target Variables Library.lvlib\\Sampling Rate"() -> (w1272:dbl)  [unwired: 1 in, 1 out]
      n538 = call-poly <vilib>:"DAQmx Create Virtual Channel.vi"("maximum value"=5.0 ("Max Voltage"), "minimum value"=0.0 ("Min Voltage"), "input terminal configuration"=w1307, "physical channels"=w1273) -> ("task out"=w1308:refnum<k21>, "error out"=w1309:errorcluster)  [unwired: 10 in]
      n539 = call-poly <vilib>:"DAQmx Create Virtual Channel.vi"("maximum value"=10.0, "minimum value"=-10.0, "output terminal configuration"=w1297, "physical channels"=w1302) -> ("task out"=w1304:refnum<k21>, "error out"=w1303:errorcluster)  [unwired: 10 in]
      n540 = shared-variable "NI-GenericDesktopPC-3A84958E\\Kopco PS Project Target Variables Library.lvlib\\Zero Flux Calibrated Core"() -> (w1287:dbl)  [unwired: 1 in, 1 out]
      n541 = call-poly <vilib>:"DAQmx Timing.vi"("task/channels in"=w1308, "sample mode"=w1310, "rate"=w1272, "error in"=w1309) -> ("task out"=w1300:refnum<k21>, "error out"=w1296:errorcluster)  [unwired: 10 in]
      n542 = call "Get Terminal Name with Device Prefix.vi"("error in"=w1296, "Local Terminal Name"="ai/SampleClock", "task/channels in"=w1300) -> ("error out"=w1289:errorcluster, "Terminal Name with Device Prefix"=w1295:tag, "task out"=w1290:refnum<k21>)  [unwired: 6 in]
      n543 = call-poly <vilib>:"DAQmx Timing.vi"("task/channels in"=w1304, "sample mode"=w1301, "rate"=w1272, "source"=w1295, "error in"=w1303) -> ("task out"=w1292:refnum<k21>, "error out"=w1293:errorcluster)  [unwired: 9 in]
      n544 = call <vilib>:"DAQmx Start Task.vi"("task/channels in"=w1292, "error in"=w1293) -> ("task out"=w1283:refnum<k21>, "error out"=w1282:errorcluster)  [unwired: 12 in]
      n545 = Merge Errors(w1289, w1282) -> (w1291:errorcluster)
    }
    frame #19 {
      # "1/4 wave to get the main points of the mini DeGauss waveform 3/12/2018"
      n546 = while "Digital Trigger from Master Data Logger" {
        tunnel: [w1359] -> w1341
        tunnel: w1342 -> [w1359]
        tunnel: w1340 -> [w1358]
        tunnel: [w1358] -> w1339
        tunnel: w1338 -> [w1357]
        tunnel: [w1357] -> w1337
        tunnel: [w1356] -> w1336
        tunnel: w1335 -> [w1356]
        tunnel: w1334 -> [w1355]
        tunnel: [w1355] -> w1333
        tunnel: w1332 -> [w1354]
        tunnel: [w1354] -> w1331
        tunnel: w1330 -> [w1353]
        tunnel: [w1353] -> w1329
        tunnel: w1328 -> [w1352]
        tunnel: [w1352] -> w1327
        tunnel: w1326 -> [w1351]
        tunnel: [w1351] -> w1325
        tunnel: w1324 -> [w1350]
        tunnel: [w1350] -> w1323
        tunnel: w1322 -> [w1349]
        tunnel: [w1349] -> w1321
        tunnel: w1320 -> [w1348]
        tunnel: [w1348] -> w1319
        tunnel: w1318 -> [w1347]
        tunnel: [w1347] -> w1317
        tunnel: w1316 -> [w1346]
        tunnel: [w1346] -> w1315
        tunnel: w1314 -> [w1343]
        tunnel: w1313 -> [w1344]
        tunnel: [w1344] -> w1312
        tunnel: [w1343] -> w1311
        stop <- w1360 stop-if-true
        # "Bound to Digital Trigger Real-Time Shared Variable"
        n547 = shared-variable "NI-GenericDesktopPC-3A84958E\\Kopco PS Project Target Variables Library.lvlib\\Digital Trigger"() -> (w1360:bool)  [unwired: 1 in, 1 out]
        "DigitalTrigger" <- w1360
        n548 = Wait (ms)(milliseconds to wait=u32 1) -> ()  [unwired: 1 out]
      }
    }
    frame #20 {
      w1373 = 0  # Last Current AO Index
      w1378 = 0  # 0-14 Mini DeGauss Sample Counter Initialized
      w1400 = T8 1 items=["All Elements Read From Stream", "All Elements Available for Reading"] ("wait condition")
      w1377 = 30  # # of samples pushed  to PID loop
      w1424 = 0  # 0-29 PID Sample Counter Initialized
      # "Reset Digital trigger in case program gets stuck"
      # "Boxes left outside to minimize freezing. Otherwise, you can see it counting in real-time"
      # "Moved Outside 3/31/2018"
      # "# of samples of Mini DeGauss"
      # "Bound to \"DataUpload\" shared variable"
      # "Abs(AO_nf) + Abs(AO_on,last)"
      # "AO_Last"
      # "Set PID \nReinitialize as true\ninitialially"
      # "Mini DeGauss AO Sequence, Normalized"
      # "Mini DeGauss PID CTRL ON/OFF Logical"
      # "AO,last"
      # "Step 5 Pushing Data to Datalogger"
      # "Step 5 Carrying out Waveform"
      # "ON PID Gain"
      # "OFF PID Gains"
      # "Flux ON/OFF CTRL Setpoint Sequence Logical"
      # "Increased buffer size to 100Mil on 1/1/2018"
      # "For 2 minutes"
      # "Calibrated Zero"
      # "PID Sampling interval, dt"
      # "Total Number of Samples"
      # "Note 1: Even though the parameters can be\nbrought into the loop \nand changed in real time. We want to avoid this\nNote 2: These parameters are for control in the linear range 0-175 GS absolute.\nFor non-linear range, you will need PID Gain Scheduling VI"
      # "Sample Rate (Hz or s^-1)\nor Step Duration (Each step is one second)"
      # "Offset by 1 removed \non 8/3/2017.\nIt solved problem. All\nData is there!"
      # "PS does not turn off unless two values are written."
      # "Maybe use it to replace the last value?"
      # "Removed Digital Trigger DAQmx and replaced\nwith real-time global variable before that"
      # "Flux Control Setpoint Sequence"
      n549 = shared-variable "NI-GenericDesktopPC-3A84958E\\Kopco PS Project Target Variables Library.lvlib\\Digital Trigger"(FALSE ("DigitalTrigger")) -> ()  [unwired: 1 in, 1 out]
      n550 = Unbundle(w1387) -> ("proportional gain (Kc)"=w1386:dbl, "integral time (Ti, min)"=w1385:dbl, "derivative time (Td, min)"=w1384:dbl)
      n551 = Build Array "PID Parameters OFF"(w1386, w1385, w1384) -> (w1388:dbl[])
      n552 = Unbundle(w1382) -> ("proportional gain (Kc)"=w1419:dbl, "integral time (Ti, min)"=w1418:dbl, "derivative time (Td, min)"=w1417:dbl)
      n553 = Build Array "PID Parameters ON"(w1419, w1418, w1417, w1377, w1380) -> (w1416:dbl[])
      n554 = Reciprocal "Sample interval"(x=w1380) -> (1/x=w1420:dbl)
      n555 = shared-variable "NI-GenericDesktopPC-3A84958E\\Kopco PS Project Target Variables Library.lvlib\\PID Parameters OFF"(w1388) -> ()  [unwired: 1 in, 1 out]
      n556 = shared-variable "NI-GenericDesktopPC-3A84958E\\Kopco PS Project Target Variables Library.lvlib\\PID Parameters ON"(w1416) -> ()  [unwired: 1 in, 1 out]
      n557 = call-poly <vilib>:"DAQmx Create Timing Source.vi"("task/channels in"=w1428, "sleep time (us)"=1.0, "error in"=w1429) -> ("task out"=w1392:refnum<k21>, "timing source out"=w1363:string, "error out"=w1412:errorcluster)  [unwired: 10 in]
      n558 = Multiply "PID Sampling Interval, dt"(x=w1377, y=w1420) -> (x*y=w1415:dbl)
      n559 = Create Network Stream Writer Endpoint(7:100000000 ("writer buffer size"), 9:0.0 ("Double"), 11:"FluxWriter" ("writer name")) -> (0:w1404:errorcluster, 3:w1403:refnum<k21>)  [unwired: 4 in]
      n560 = Initialize Array "Initialize Array\nof samples to PID"(0.0 ("sleep time (us)"), w1377) -> (w1413:dbl[])
      n561 = shared-variable "NI-GenericDesktopPC-3A84958E\\Kopco PS Project Target Variables Library.lvlib\\Sensor Sensitivity Core"() -> (w1361:dbl)  [unwired: 1 in, 1 out]
      n562 = Array Size(array=w1421) -> (size(s)=w1422:i32)
      n563 = Subtract(x=w1422, y=0) -> (x-y=w1414:i32)
      n564 = node-c288(w1363) -> (w1409:T3)  [unwired: 3 in]
      n565 = Quotient & Remainder(x=w1377, y=2) -> (floor(x/y)=w1372:i32)  [unwired: 1 out]
      n566 = timed-loop "Lower priority deterministic Code for Data Collection to Data Logger" {
        timing: w1409 -> [_]
        timing-out: [_] -> w1408
        tunnel: w1393 -> [w1432]
        tunnel: w1404 -> [w1445]
        tunnel: [w1433] -> w1398
        tunnel: [w1443] -> w1399
        tunnel: w1403 -> [w1444]
        shift-right: [w1435] -> _
        shift-left: -1 ("y") -> [w1434]
        tunnel: [w1432] -> w1367
        tunnel: [w1431] -> w1366
        i -> [w1431]
        stop <- w1439 stop-if-true
        # "Switch OFF Null Flux currently running indicator. Placed in non-deterministic loop so as not to"
        # "Using variable bound\nto the toggle generate the error message\nthat remote endpoint is destroyed."
        n567 = node-c288() -> ()  [unwired: 1 in, 1 out]
        n568 = shared-variable ".\\Kopco PS Project Target Variables Library.lvlib\\Data RT Index"() -> (w1435:i64)  [unwired: 1 in, 1 out]
        n569 = shared-variable ".\\Kopco PS Project Target Variables Library.lvlib\\Data RT Current"() -> (w1441:dbl)  [unwired: 1 in, 1 out]
        n570 = shared-variable ".\\Kopco PS Project Target Variables Library.lvlib\\Data RT Exposure"() -> (w1440:dbl)  [unwired: 1 in, 1 out]
        n571 = shared-variable ".\\Kopco PS Project Target Variables Library.lvlib\\Data RT Flux"() -> (w1442:dbl)  [unwired: 1 in, 1 out]
        n572 = Greater?(x=w1431, y=w1434) -> ()  [unwired: 1 out]
        n573 = shared-variable "NI-GenericDesktopPC-3A84958E\\Kopco PS Project Target Variables Library.lvlib\\Null Flux Running Middle"(FALSE ("Null Flux Running Middle")) -> ()  [unwired: 1 in, 1 out]
        n574 = Greater Or Equal?(x=w1431, y=w1432) -> (x >= y?=w1439:bool)
        n575 = Build Array(w1435, w1442, w1441, w1440) -> (w1438:dbl[])
        n576 = shared-variable-write(w1444, w1445, w1438) -> (w1443:refnum<k21>, w1433:errorcluster)  [unwired: 1 in, 1 out]
        n577 = Not(x=w1439) -> (.not. x?=w1437:bool)
        n578 = shared-variable ".\\Kopco PS Project Target Variables Library.lvlib\\Data Upload"(w1437) -> ()  [unwired: 1 in, 1 out]
        n579 = node-c288() -> ()  [unwired: 1 in, 1 out]
      }
      "# of Data Points" <- w1366
      "Loop Index" <- w1367
      n580 = node-c288(w1363) -> (w1427:T3)  [unwired: 9 in]
      n581 = timed-loop "PID Control Loop" {
        tunnel: [w1508] -> _
        tunnel: w1425 -> [w1511]
        tunnel: [w1491] -> w1411
        tunnel: w1421 -> [w1509]
        timing: w1427 -> [_]
        timing-out: [_] -> w1426
        shift-right: [w1457] -> _
        shift-left: w1374 -> [w1484]
        shift-right: [w1505] -> _
        shift-left: w1413 -> [w1503]
        tunnel: w1413 -> [w1502]
        shift-right: [w1501] -> _
        shift-left: w1424 -> [w1500]
        tunnel: w1422 -> [w1504]
        tunnel: w1414 -> [_]
        tunnel: w1377 -> [w1482]
        tunnel: w1382 -> [w1488]
        tunnel: w1415 -> [w1494]
        tunnel: w1412 -> [w1493]
        tunnel: [w1492] -> w1396
        tunnel: [w1491] -> w1383
        tunnel: w1392 -> [w1490]
        tunnel: w1391 -> [w1489]
        tunnel: w1389 -> [w1487]
        tunnel: w1387 -> [w1486]
        tunnel: w1381 -> [w1485]
        tunnel: w1379 -> [w1483]
        shift-right: [w1480] -> _
        shift-left: w1378 -> [w1478]
        tunnel: w1372 -> [w1479]
        shift-right: [w1476] -> _
        shift-left: TRUE -> [w1475]
        tunnel: w1374 -> [w1474]
        shift-right: [w1472] -> _
        shift-left: w1374 -> [w1473]
        shift-right: [w1470] -> _
        shift-left: w1373 -> [w1471]
        tunnel: w1371 -> [w1469]
        tunnel: [w1465] -> w1369
        tunnel: "8. Keep Final Flux Running at End?" -> [w1464]
        tunnel: w1364 -> [w1456]
        tunnel: w1362 -> [w1455]
        tunnel: w1361 -> [w1454]
        i -> [w1466]
        stop <- w1467 continue-if-true
        # "Reversed order of AI7 & AI3 on 4/11/2018 to \nminimize leakage to Channel 7"
        # "No PID Control/DeGauss\nwhen control sequence is exceeded 3/31/2018"
        # "Stop this loop once data is uploaded"
        # "Calibrated Zero"
        # "AO_Null Flux"
        # "Rewrite to AO for now to see what it actually outputs.,  3/8/2018."
        # "AO last"
        # "AO"
        # "PID Sampling interval, dt"
        # "Number of samples pushed to PID\nper time"
        # "Current Flux\nSetpoint Value"
        # "Flux AI Reading"
        # "Array size"
        n582 = node-c288() -> ()  [unwired: 1 in, 1 out]
        n583 = Index Array "Current\nFlux Setpoint"(array=w1509, index=w1466) -> (element=w1507:dbl)
        n584 = Less Or Equal? "Less than 30 Samples"(x=w1500, y=w1482) -> (x <= y?=w1459:bool)
        n585 = call-poly <vilib>:"DAQmx Read.vi"("task/channels in"=w1490, "error in"=w1493) -> ("task out"=w1508:refnum<k21>, "data"=w1497:dbl[], "error out"=w1510:errorcluster)  [unwired: 11 in]
        n586 = Less Or Equal? "Less than 15 Samples"(x=w1478, y=w1479) -> (x <= y?=w1481:bool)
        n587 = Greater Or Equal? "Exceeded Datapoints?"(x=w1466, y=w1504) -> (x >= y?=w1458:bool)
        n588 = Delete From Array "AI5 Flux \nChannel"(array=w1497, index=1) -> (deleted portion=w1496:dbl)  [unwired: 1 in, 1 out]
        n589 = Delete From Array "AI3 Current \nChannel"(array=w1497, index=4) -> (deleted portion=w1495:dbl)  [unwired: 1 in, 1 out]
        n590 = Delete From Array "AI7 Exposure\n Channel"(array=w1497, index=2) -> (deleted portion=w1453:dbl)  [unwired: 1 in, 1 out]
        n591 = Index Array "Mini-DeGauss \nON/OFF Status?"(array=w1485, index=w1466) -> (element=w1463:bool)
        n592 = case "DeGauss Sequence ON/OFF?" shown="False" w1463 {
          tunnel: w1507 -> [w1546 _]
          tunnel: w1484 -> [w1545 _]
          tunnel: [w1544 w1605] -> w1505
          tunnel: w1459 -> [w1521 _]
          tunnel: w1503 -> [w1543 w1604]
          tunnel: w1502 -> [w1542 w1603]
          tunnel: [w1524 w1607] -> w1501
          tunnel: w1500 -> [w1541 _]
          tunnel: w1496 -> [w1540 _]
          tunnel: w1494 -> [w1539 _]
          tunnel: [w1525 w1601] -> w1477
          tunnel: w1489 -> [w1538 _]
          tunnel: w1466 -> [w1528 w1595]
          tunnel: w1488 -> [w1537 _]
          tunnel: w1487 -> [w1536 _]
          tunnel: w1486 -> [w1535 _]
          tunnel: w1483 -> [_ w1602]
          tunnel: w1481 -> [_ w1600]
          tunnel: [w1534 w1599] -> w1480
          tunnel: w1478 -> [_ w1598]
          tunnel: [w1532 TRUE] -> w1476
          tunnel: w1475 -> [w1533 _]
          tunnel: w1474 -> [w1531 w1596]
          tunnel: [w1528 w1592] -> w1470
          tunnel: w1473 -> [w1523 w1594]
          tunnel: [w1529 w1591] -> w1472
          tunnel: w1471 -> [_ w1593]
          tunnel: w1469 -> [_ w1590]
          tunnel: w1458 -> [_ w1589]
          tunnel: w1458 -> [w1522 _]
          tunnel: w1456 -> [w1519 _]
          tunnel: w1455 -> [w1518 _]
          tunnel: w1454 -> [w1516 _]
          frame False {
            w1534 = 0  # Reset Mini DeGausss Sample Counter
            # "Update Last Current AO Index with \nCurrent Sample Index"
            # "Change the Magnitude\nof miniDeGauss:\nAbs(AO_nf) + Abs(AO_on,last) \nUse Max between that and the \ndifference. Difference will be\nminimal in OFF segments, but\nmaximal in ON segments."
            # "Loop Index"
            n593 = Index Array "Flux ON/OFF \nStatus?"(array=w1536, index=w1528) -> (element=w1527:bool)
            n594 = case "Control Sequence Exceeded?" shown="True" w1522 {
              tunnel: [w1547 TRUE] -> w1520
              tunnel: w1521 -> [w1547 _]
              frame False {
              }
              frame True {
                # "No PID Control"
              }
            }
            n595 = case "PID Gain Selector" shown="True" w1527 {
              tunnel: [w1557 w1559] -> w1515
              tunnel: w1537 -> [_ w1559]
              tunnel: w1535 -> [w1557 _]
              tunnel: w1519 -> [_ w1558]
              tunnel: w1518 -> [w1556 _]
              tunnel: [w1556 w1558] -> w1517
              frame False {
                # "Off Sequence"
              }
              frame True {
                # "ON Sequence"
              }
            }
            n596 = case "PID Control ON/OFF?" shown="False" w1520 {
              tunnel: w1539 -> [w1574 _]
              tunnel: w1546 -> [w1573 _]
              tunnel: [w1572 w1588] -> w1526
              tunnel: w1545 -> [_ w1588]
              tunnel: [w1579 w1586] -> w1544
              tunnel: w1543 -> [w1576 w1585]
              tunnel: w1542 -> [w1578 _]
              tunnel: [w1577 w1587] -> w1524
              tunnel: w1541 -> [_ w1584]
              tunnel: w1540 -> [_ w1583]
              tunnel: w1538 -> [w1565 _]
              tunnel: w1533 -> [w1570 w1582]
              tunnel: [FALSE w1582] -> w1532
              tunnel: w1531 -> [w1568 w1581]
              tunnel: [w1568 w1581] -> w1530
              tunnel: w1517 -> [w1567 _]
              tunnel: w1516 -> [w1564 _]
              tunnel: w1515 -> [_ _]
              frame False {
                w1577 = 0  # PID Sample Counter
                # "Offset was added to AO output\nby PID to eliminate the problem of\noutputing 0V for AO when there is \nlittle to no change in PV, which caused\na dip in response until PID recovers."
                # "Tried adding AO 0 to PID AO output. It works find with Null Flux, but \nnot with the anything where AO is not zero. It becomes like a run-away reaction. \nIt turns out that was because I added the indexed Flux value instead of the Null Flux AO.\nProblem Solved"
                # "flux setpoint"
                # "dt"
                # "Reset Array"
                n597 = call-poly <vilib>:"Mean.vi"("X"=w1576) -> ("mean"=w1566:dbl)  [unwired: 1 out]
                n598 = Subtract "PV-SP"(x=w1566, y=w1565) -> (x-y=w1562:dbl)
                n599 = Absolute Value(x=w1562) -> (abs(x)=w1560:dbl)
                n600 = Divide(x=w1560, y=w1564) -> (x/y=w1563:dbl)
                n601 = call-poly <vilib>:"PID Gain Schedule.vi"("PID gain schedule"=w1567, "gain scheduling value"=w1563) -> ("PID gains out"=w1561:T1)  [unwired: 2 in, 1 out]
                n602 = call-poly <vilib>:"PID.vi"("reinitialize? (F)"=w1570, "output range"=T6 {"Max/Min \ncontroller outputs"=10.0, "output low"=-10.0}, "dt (s)"=w1574, "PID gains"=w1561, "process variable"=w1562, "setpoint"=w1573) -> ("output"=w1571:dbl)  [unwired: 4 in, 1 out]
                n603 = Replace Array Subset "Reset Flux Array \nfed to PID"(array=w1576, new element=w1578, index=0) -> (w1579:dbl[])
                n604 = Add "Offset"(x=w1568, y=w1571) -> (x+y=w1572:dbl)
              }
              frame True {
                # "PID Sample Counter Index"
                # "AO last"
                # "Flux AI Reading"
                n605 = Increment "Increment\nto next\nindex"(x=w1584) -> (x+1=w1587:i32)
                n606 = Replace Array Subset "Replace ith item \nin Array fed to PID"(array=w1585, new element=w1583, index=w1584) -> (w1586:dbl[])
              }
            }
            n607 = case "Mini DeGauss Magnitude\nSelector" shown="True" w1527 {
              tunnel: w1530 -> [_ w1555]
              tunnel: [w1550 w1552] -> w1529
              tunnel: [w1549 w1551] -> w1525
              tunnel: w1526 -> [w1549 w1551]
              tunnel: w1523 -> [w1550 _]
              frame False {
              }
              frame True {
                n608 = Absolute Value "Abs[AO_on,last]"(x=w1551) -> (abs(x)=w1554:dbl)
                n609 = Absolute Value "Abs[AO_nf]"(x=w1555) -> (abs(x)=w1553:dbl)
                n610 = Add(x=w1554, y=w1553) -> (x+y=w1552:dbl)
              }
            }
          }
          frame True {
            w1607 = 0  # PID Sample Counter
            # "Leave Index unchanged\nDuring Mini DeGauss\nsequence"
            # "current sample index"
            # "Abs(AO_nf) + Abs(AO_on,last)"
            # "Null Flux AO"
            # "NO PID sequence. DeGaussing Sequence"
            n611 = case "Mini DeGauss Updated AO?" shown="True" w1600 {
              tunnel: w1602 -> [_ w1626]
              tunnel: [w1610 w1624] -> w1601
              tunnel: [w1612 w1625] -> w1599
              tunnel: w1598 -> [w1611 _]
              tunnel: w1595 -> [_ w1623]
              tunnel: w1596 -> [w1610 w1617]
              tunnel: w1594 -> [w1608 w1619]
              tunnel: w1593 -> [w1609 w1621]
              tunnel: [w1609 w1621] -> w1592
              tunnel: [w1608 w1620] -> w1591
              tunnel: w1590 -> [_ w1618]
              tunnel: w1589 -> [_ w1615]
              frame False {
                n612 = Increment "Increment\nto next\nindex"(x=w1611) -> (x+1=w1612:i32)
              }
              frame True {
                w1625 = 0  # Reset Mini DeGausss Sample Counter
                # "No PID Control/DeGauss\nwhen control sequence is exceeded 3/31/2018"
                # "Removed the offset\nand kept amplitude the same"
                # "Take the value once every 15 samples\nInitial curve is sampled at a lot more to \nminimize aliasing of the proper waveform"
                n613 = Index Array "Mini-DeGauss \nON/OFF Status?"(array=w1626, index=w1623) -> (element=w1616:dbl)
                n614 = Subtract "Reset"(x=w1623, y=w1621) -> (x-y=w1622:i32)
                n615 = Greater Or Equal? "Index of Cut off"(x=w1622, y=w1618) -> (x >= y?=w1613:bool)
                n616 = case "Control Sequence Exceeded?" shown="True" w1615 {
                  tunnel: [w1627 TRUE] -> w1614
                  tunnel: w1613 -> [w1627 _]
                  frame False {
                  }
                  frame True {
                    # "No PID Control"
                  }
                }
                n617 = case shown="True" w1614 {
                  tunnel: [w1630 w1632] -> w1624
                  tunnel: w1617 -> [_ w1632]
                  tunnel: w1616 -> [w1630 _]
                  tunnel: [w1629 w1631] -> w1620
                  tunnel: w1619 -> [w1629 w1631]
                  frame False {
                  }
                  frame True {
                  }
                }
              }
            }
            n618 = Replace Array Subset "Reset Flux Array \nfed to PID"(array=w1604, new element=w1603, index=0) -> (w1605:dbl[])
          }
        }
        n619 = shared-variable ".\\Kopco PS Project Target Variables Library.lvlib\\Data RT Exposure"(w1453) -> ()  [unwired: 1 in, 1 out]
        n620 = shared-variable ".\\Kopco PS Project Target Variables Library.lvlib\\Data RT Current"(w1495) -> ()  [unwired: 1 in, 1 out]
        n621 = shared-variable ".\\Kopco PS Project Target Variables Library.lvlib\\Data RT Flux"(w1496) -> ()  [unwired: 1 in, 1 out]
        n622 = shared-variable ".\\Kopco PS Project Target Variables Library.lvlib\\Data RT Index"(w1466) -> ()  [unwired: 1 in, 1 out]
        n623 = case shown="True" w1458 {
          tunnel: [w1634 w1636] -> w1457
          tunnel: w1477 -> [w1634 w1637]
          tunnel: [w1633 w1635] -> w1465
          tunnel: w1464 -> [w1633 w1635]
          frame False {
          }
          frame True {
            (unwired) FALSE ("y")
            # "A Toggle fixed the problem!"
            n624 = case shown="False" w1635 {
              tunnel: [0.0 ("output") w1639] -> w1636
              tunnel: w1637 -> [_ w1639]
              frame False {
                # "Reset AO at the end"
              }
              frame True {
                # "Keep Flux the same"
              }
            }
          }
        }
        n625 = call-poly <vilib>:"DAQmx Write.vi"("task/channels in"=w1511, "data"=w1457, "error in"=w1510) -> ("task out"=w1491:refnum<k21>, "error out"=w1492:errorcluster)  [unwired: 10 in, 1 out]
        n626 = case shown="True" w1458 {
          tunnel: [FALSE w1514] -> w1460
          frame False {
          }
          frame True {
            n627 = shared-variable ".\\Kopco PS Project Target Variables Library.lvlib\\Data Upload"() -> (w1513:bool)  [unwired: 1 in, 1 out]
            n628 = Not "No longer uploading"(x=w1513) -> (.not. x?=w1514:bool)
          }
        }
        n629 = Unbundle By Name(w1492) -> ("status"=w1468:bool)  [unwired: 2 out]
        n630 = Not(x=w1460) -> (.not. x?=w1461:bool)
        n631 = Not(x=w1468) -> (.not. x?=w1462:bool)
        n632 = And(x=w1462, y=w1461) -> (x .and. y?=w1467:bool)
        n633 = node-c288() -> ()  [unwired: 1 in, 1 out]
      }
      n634 = node-c288(w1408) -> (w1390:errorcluster)
      n635 = Flush Stream(8:w1398, 10:w1400, 11:w1399) -> (0:w1401:errorcluster, 3:w1402:refnum<k21>)  [unwired: 1 in, 1 out]
      n636 = Destroy Stream Endpoint(8:w1401, 11:w1402) -> (0:w1395:errorcluster)
      n637 = node-c288(w1426) -> (w1397:errorcluster)
      n638 = shared-variable "NI-GenericDesktopPC-3A84958E\\Kopco PS Project Target Variables Library.lvlib\\Null Flux Running End"(w1369) -> ()  [unwired: 1 in, 1 out]
      n639 = Merge Errors(w1397, w1396, w1390, w1395) -> (w1394:errorcluster)
    }
    frame #21 {
      # "Bound to \"Null Flux Running End\""
      n640 = call <vilib>:"DAQmx Stop Task.vi"("task/channels in"=w1648, "error in"=w1647) -> ("task out"=w1654:refnum<k21>, "error out"=w1653:errorcluster)  [unwired: 12 in]
      n641 = call <vilib>:"DAQmx Clear Task.vi"("task in"=w1654, "error in"=w1653) -> ("error out"=w1650:errorcluster)  [unwired: 13 in]
      n642 = call <vilib>:"DAQmx Stop Task.vi"("task/channels in"=w1649, "error in"=w1650) -> ("task out"=w1652:refnum<k21>, "error out"=w1651:errorcluster)  [unwired: 12 in]
      n643 = call <vilib>:"DAQmx Clear Task.vi"("task in"=w1652, "error in"=w1651) -> ()  [unwired: 13 in, 1 out]
    }
  }
